vi "MC_8_9_12a_PD.vi"() -> ()   [LabVIEW 2011]
uses:
  <vilib>/Utility/file.llb/Read From Spreadsheet File (string).vi
  <vilib>/Utility/inputDevices.llb/keyboardAcquire.vi
  <vilib>/Utility/file.llb/Write To Spreadsheet File (DBL).vi
  <vilib>/Utility/file.llb/Write To Spreadsheet File (string).vi
  <vilib>/regexp/Match Regular Expression.xnode
panel:
  out "Opj X Axis":string
  in  "Room Temp":dbl=294.0
  out "No Image 2":path=path "\\\\acad1\\physics/Jurchescu-group/JW-PD/Image Not Found.png"
  out "Save1 Array":string[][](array[string])
  out "Lin Vd":dbl
  out "Lin-Vg Array-Used":dbl[](array[numeric])
  out "Lin Id-Used":dbl[](array[numeric])
  out "Comments":string
  out "Folder Index":dbl caption="Length"
  out "Current \nRecord":string[](array[string])
  out "Transformer \nHeaders":string[](array[string])
  out "Current Device ID":string
  out "Column":string
  out "Row":string
  out "Rec: Concentration":dbl
  out "Rec: Solvent":string
  out "Rec: Method":string
  in  "?":T1(tab)
  in  "Transport File":path
  out "Transport Folder":path
  out "Rec: Material":string
  in  "Treatment Concentration (mM):":dbl=nan
  in  "Surface Treatment:":string="NaN"
  in  "# Drops*:":dbl=inf
  in  "Solution Temp (C):":dbl=nan
  in  "Relative Humidity (%):":dbl=nan
  in  "Room Temp (F):":dbl=nan
  in  "Time (s):":dbl=nan
  out "Accel (RPM/s):":dbl
  in  "RPM:":dbl=nan
  in  "Wait Time (s):":dbl=nan
  in  "Sample #:":dbl=1.0
  in  "Fabricator:":string="NaN"
  in  "Transfer File":path
  out "Transfer Folder":path
  in  "Image Folder":path
  out "Image File":path=path "D:/UserData/Desktop/Jeremy/WFU/Research/Programs/VI mods/Image Not Found.png"
  in  "Ramp (s):":dbl=3.0
  out "Calc: On/Off":dbl caption="On/Off-Sat" format="%#.2e"
  out "Calc: Off I-Sat":dbl caption="Off I-Sat" format="%#.2e"
  in  "Manuel-Dielectric":bool
  in  "Manuel-Length":bool
  out "Calc: VT-Lin":dbl
  out "New: VT-Lin":dbl
  out "Rec: VT-Lin":dbl caption="VT-Lin" format="%#_3g"
  out "Calc: Trap Density-STS":dbl format="%#.2e"
  out "New: Trap Density-STS":dbl format="%#.2e"
  out "Rec: Trap Density-STS":dbl caption="N-Sat (STS)" format="%#.2e"
  out "Calc: Trap Density-VT":dbl format="%#.2e"
  out "New: Trap Density-VT":dbl format="%#.2e"
  out "Rec: Trap Density-VT":dbl caption="N-Sat (VT)" format="%#.2e"
  out "Calc: Mobility-Lin":dbl format="%#.2e"
  out "New: Mobility-Lin":dbl format="%#_4e"
  out "Rec: Mobility-Lin":dbl caption="Mobility-Lin" format="%#_3e"
  out "Calc: Mobility-Sat":dbl format="%#.2e"
  out "Rec: Length":dbl caption="Length" format="%#_3g"
  out "Rec: Width":dbl caption="Width" format="%#_4g"
  out "Rec: Dielectric (d)":dbl caption="Dielectric (d)" format="%#_3g"
  in  "Cancel Button":bool
  in  "Up Button":bool
  in  "Down Button":bool
  out "Data Name:":string
  in  "Save Changes?":bool
  in  "New: Dielectric":dbl
  in  "New: Length":dbl
  in  "New: Width":dbl
  out "New: Mobility-Sat":dbl format="%#.2e"
  in  "Blank Button":bool
  in  "Zoom":i16(slide)=-3 scale=-5.0..5.0
  out "Image Out 2":T2(plugin-control)
  out "Image Out":T2(plugin-control)
  in  "Magnification":u16(ring) items=["5x", "10x", "20x", "50x", "80x"]
  out "Total Width":dbl
  out "Distances":dbl[](array[numeric])
  in  "Undo Button":bool
  in  "Remove Button":bool
  out "Rec: Mobility-Sat":dbl caption="Mobility-Sat" format="%#.2e"
  out "Index":string
  out "Image Name":string
  in  "Export":bool
  out "Calc: VT-Sat":dbl format="%#.2g"
  out "New: VT-Sat":dbl format="%#.2g"
  in  "Manual-Width":bool caption="Manual"
  out "Calc: STS":dbl format="%#.2g"
  out "New: STS":dbl format="%#.2g"
  out "Rec: VT-Sat":dbl caption="VT-Sat" format="%#.2g"
  out "Rec: STS":dbl caption="STS-Sat" format="%#.2g"
  out "Rec: On/Off":dbl caption="On/Off-Sat" format="%#.2e"
  in  "Save Changes? 2":bool
  in  "Save Changes? 3":bool
  out "Date Recorded":string="Date Recorded" caption="Measured"
  out "Date Created":string caption="Fabricated"
  out "Rec: Temp":dbl caption="Sample Temp" format="%.1f"
  in  "New: Temp":dbl format="%.1f"
  out "Rec: Off I-Sat":dbl caption="Off I-Sat" format="%#.2e"
  in  "Independant Variable":string(combo)="Length (um):"
  in  "Transfer Plots":enum32{"Linear", "Saturation"}(tab)=enum."Saturation"
  out "XY Graph-Lin":cluster{dbl[], dbl[]}[](graph)
  in  "Slide":dbl(slide) step=1.0 scale=-22.0..89.0 scale format="%#_1p"
  out "XY Graph":cluster{dbl[], dbl[]}[](graph)
  in  "Previous Button":bool
  in  "Next Button":bool
  in  "NumPts":dbl=5.0
  in  "Log Plots":enum32{"Linear", "Saturation"}(tab)=enum."Saturation"
  in  "Slide 2":dbl(slide) step=1.0 scale=-1.0..82.0 scale format="%#_1p"
  out "XY Graph 2":cluster{dbl[], dbl[]}[](graph)
  in  "Previous Button 2":bool
  in  "Next Button 2":bool
  in  "NumPts 2":dbl=5.0 caption="NumPts"
  in  "Manual-Temp":bool caption="Manual"
  in  "Origin Project File":path=path "\\\\acad1\\physics/Jurchescu-group/JW-PD/Group Library/Origin Project Files/DeviceData_7_31_12b_JW.opj"
  in  "No Image File":path=path "\\\\acad1\\physics/Jurchescu-group/JW-PD/Mega Awesome/Image Not Found.png"
  out "String":string
  out "Index 2":dbl
  out "Sat Id-Log-Used":dbl[](array[numeric])
  out "Vg Array-Log-Used":dbl[](array[numeric])
  out "ROI Descriptor out":T3 {"Contours"."Type" items=["No Selection", "Point", "Line", "Rectangle", "Oval", "Polygon", "Freehand Region", "Annulus", "Unused2", "Unused3", "Broken Line", "Freehand Line", "Rotated Rectangle"]}
  out "ROI Descriptor":T3 {"Contours"."Type" items=["No Selection", "Point", "Line", "Rectangle", "Oval", "Polygon", "Freehand Region", "Annulus", "Unused2", "Unused3", "Broken Line", "Freehand Line", "Rotated Rectangle"]}
  out "Numeric 3":dbl
  out "Array 6":dbl[][](array[numeric])
  out "Cluster":T4
  out "Array 5":dbl[](array[numeric])
  out "Array 4":dbl[](array[numeric])
  out "Array 3":dbl[](array[numeric])
  out "Numeric 2":dbl
  out "Numeric":dbl
  out "Sat Id-Used":dbl[](array[numeric])
  out "Sat Vg Array-Used":dbl[](array[numeric])
  out "MobVi Index":dbl
  in  "Row Start":dbl=20.0
  # "Data Locations"
  # "Transport Location"
  # "Transfer Location"
  # "Image Location"
  # "Sample Properties"
  # "*     Inf = Full coverage\n   NaN = Unknown or Not Applicable"
  # "Recorded"
  # "Calculated"
  # "Re-Calculated"
  # "Manual"
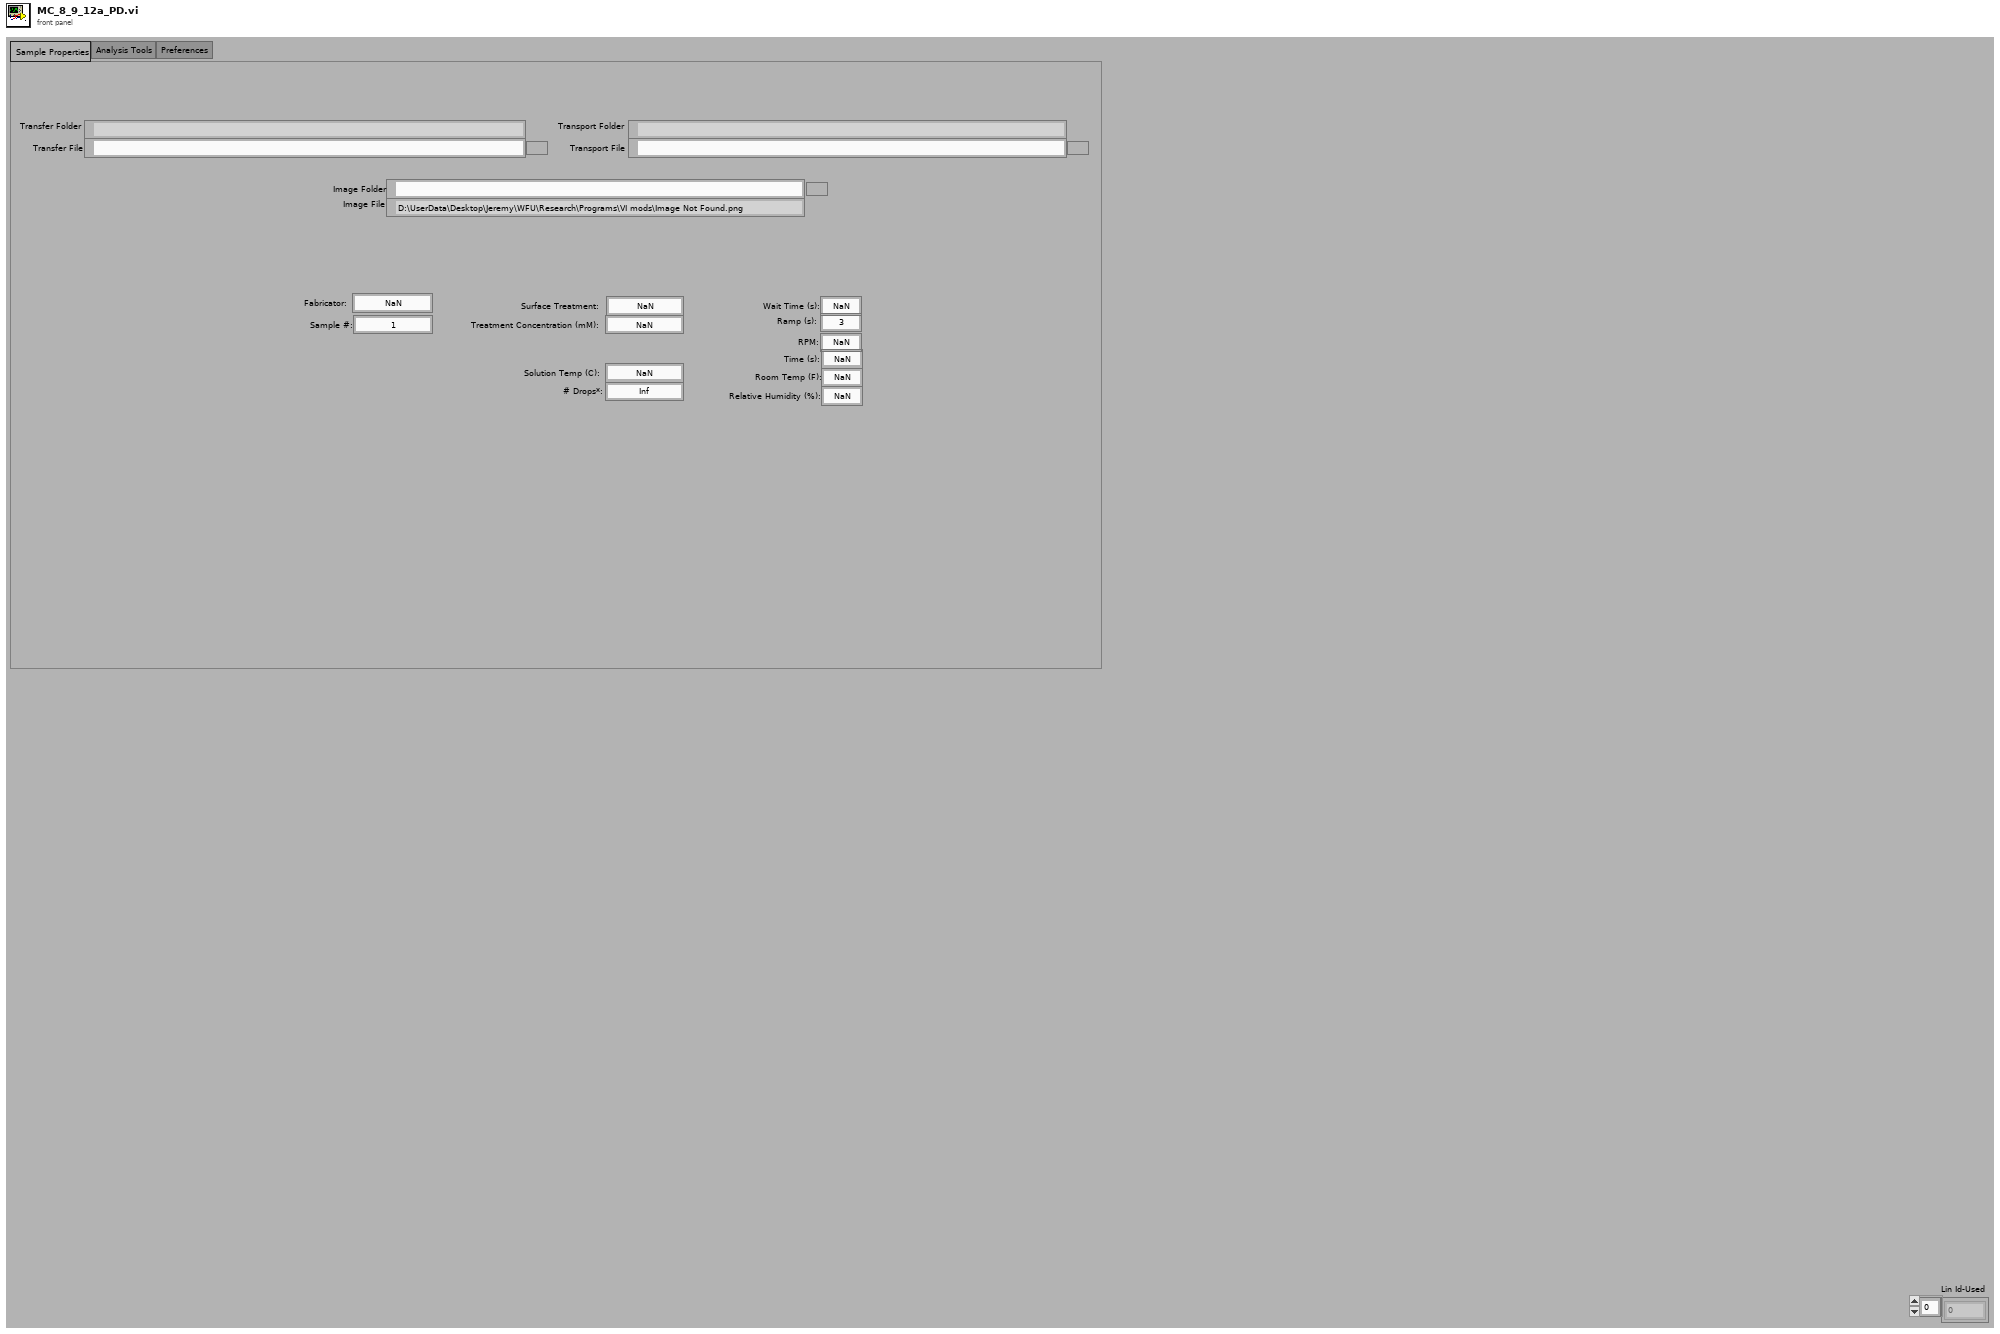
[diagram p1: front panel]
types:
  T1 = enum32{"Sample Properties", "Analysis Tools", "Preferences", "Current Database"}
  T2 = typedef "IMAQ Image.ctl" = refnum<image>
  T3 = typedef "ROI Descriptor" = cluster{"Global Rectangle":i32[], "Contours":cluster{"ID":enum32{"External", "Internal"}, "Type":u32, "Coordinates":i32[]}[]}
  T4 = cluster{"Numeric":dbl, "Numeric 2":dbl, "Numeric 3":dbl, "Numeric 4":dbl}
  T5 = cluster{"Mobility-Sat":dbl, "Moblitity-Lin":dbl, "On/Off":dbl, "Off Current":dbl, "Vt-Sat":dbl, "STS":dbl, "Trap Density-VT":dbl, "Trap Density-STS":dbl}
  T6 = cluster{"Date Recorded":string, "Index":string, "Length":dbl, "Width":dbl, "Sample Temp":dbl}
  T7 = cluster{"Date Created":string, "Material":string, "Solvent":string, "Concentration":dbl, "Method":string, "Dielectric (nm)":dbl, "Treatment":string, "Comments":string}
  T8 = cluster{"Mobility-Sat":dbl, "Vt-Sat":dbl, "Mobility-Lin":dbl, "Vt-Lin":dbl, "Off I-Sat":dbl, "On/Off I-Sat":dbl}
  T9 = cluster{"[0]":cluster{dbl[], dbl[]}, "[1]":cluster{dbl[], dbl[]}, "[2]":cluster{dbl[], dbl[]}, "[3]":cluster{dbl[], dbl[]}, "[4]":cluster{dbl[], dbl[]}, "[5]":cluster{dbl[], dbl[]}, "[6]":cluster{dbl[], dbl[]}, "[7]":cluster{dbl[], dbl[]}, "[8]":cluster{dbl[], dbl[]}}
  T10 = cluster{"Global Rectangle":i32[], "Contours":cluster{"Contour Type":u32, "ROI Type":u32, "Points":i32[]}[]}
  T11 = typedef "LVBoundsTypeDef.ctl" = cluster{"Width":u32, "Height":u32}
  T12 = enum16{"0", "1", "2", "3", "4", "5", "6", "7", "8", "9", "A", "B", "C", "D", "E", "F", "G", "H", "I", "J", "K", "L", "M", "N", "O", "P", "Q", "R", "S", "T", "U", "V", "W", "X", "Y", "Z", "F1", "F2", "F3", "F4", "F5", "F6", "F7", "F8", "F9", "F10", "F11", "F12", "F13", "F14", "F15", "ADD", "BACK", "BACKSLASH", "CAPITAL", "COMMA", "DECIMAL", "DELETE", "DIVIDE", "DOWN", "END", "EQUALS", "ESCAPE", "GRAVE (`)", "HOME", "INSERT", "LBRACKET", "LCONTROL", "LEFT", "L ALT", "LSHIFT", "LWIN", "MINUS", "MULTIPLY", "NEXT", "NUMLOCK", "NUMPAD_0", "NUMPAD_1", "NUMPAD_2", "NUMPAD_3", "NUMPAD_4", "NUMPAD_5", "NUMPAD_6", "NUMPAD_7", "NUMPAD_8", "NUMPAD_9", "PAUSE", "PERIOD", "PRIOR (PG UP)", "RBRACKET", "RCONTROL", "RETURN", "RIGHT", "R ALT", "RSHIFT", "RWIN", "SCROLL", "SEMICOLON", "SLASH", "SPACE", "SUBTRACT", "TAB", "UP", "ENTER (num pad)", "' (quote)"}[]
  T13 = enum16{"0", "1", "2", "3", "4", "5", "6", "7", "8", "9", "A", "B", "C", "D", "E", "F", "G", "H", "I", "J", "K", "L", "M", "N", "O", "P", "Q", "R", "S", "T", "U", "V", "W", "X", "Y", "Z", "F1", "F2", "F3", "F4", "F5", "F6", "F7", "F8", "F9", "F10", "F11", "F12", "F13", "F14", "F15", "ADD", "BACK", "BACKSLASH", "CAPITAL", "COMMA", "DECIMAL", "DELETE", "DIVIDE", "DOWN", "END", "EQUALS", "ESCAPE", "GRAVE (`)", "HOME", "INSERT", "LBRACKET", "LCONTROL", "LEFT", "L ALT", "LSHIFT", "LWIN", "MINUS", "MULTIPLY", "NEXT", "NUMLOCK", "NUMPAD_0", "NUMPAD_1", "NUMPAD_2", "NUMPAD_3", "NUMPAD_4", "NUMPAD_5", "NUMPAD_6", "NUMPAD_7", "NUMPAD_8", "NUMPAD_9", "PAUSE", "PERIOD", "PRIOR (PG UP)", "RBRACKET", "RCONTROL", "RETURN", "RIGHT", "R ALT", "RSHIFT", "RWIN", "SCROLL", "SEMICOLON", "SLASH", "SPACE", "SUBTRACT", "TAB", "UP", "ENTER (num pad)", "' (quote)"}
  T14 = cluster{"Contour Type":u32, "ROI Type":u32, "Points":i32[]}[]
  T15 = cluster{i32[], cluster{"Contour Type":u32, "ROI Type":u32, "Points":i32[]}[]}
  T16 = cluster{"Independant  Variable Indicator":string, "Parameter String Indicator":string}
  T17 = cluster{string, sgl, bool, bool, bool, bool, bool, bool, i32}
  T18 = cluster{i32, cluster{string, sgl, bool, bool, bool, bool, bool, bool, i32}, i32, i32}
  T19 = cluster{"Contour Type":u32, "ROI Type":u32, "Points":i32[]}
  T20 = cluster{"Points[0]":i32, "Points[1]":i32, "Points[2]":i32, "Points[3]":i32, "Points[4]":i32, "Points[5]":i32, "Points[6]":i32, "Points[7]":i32, "Points[8]":i32}
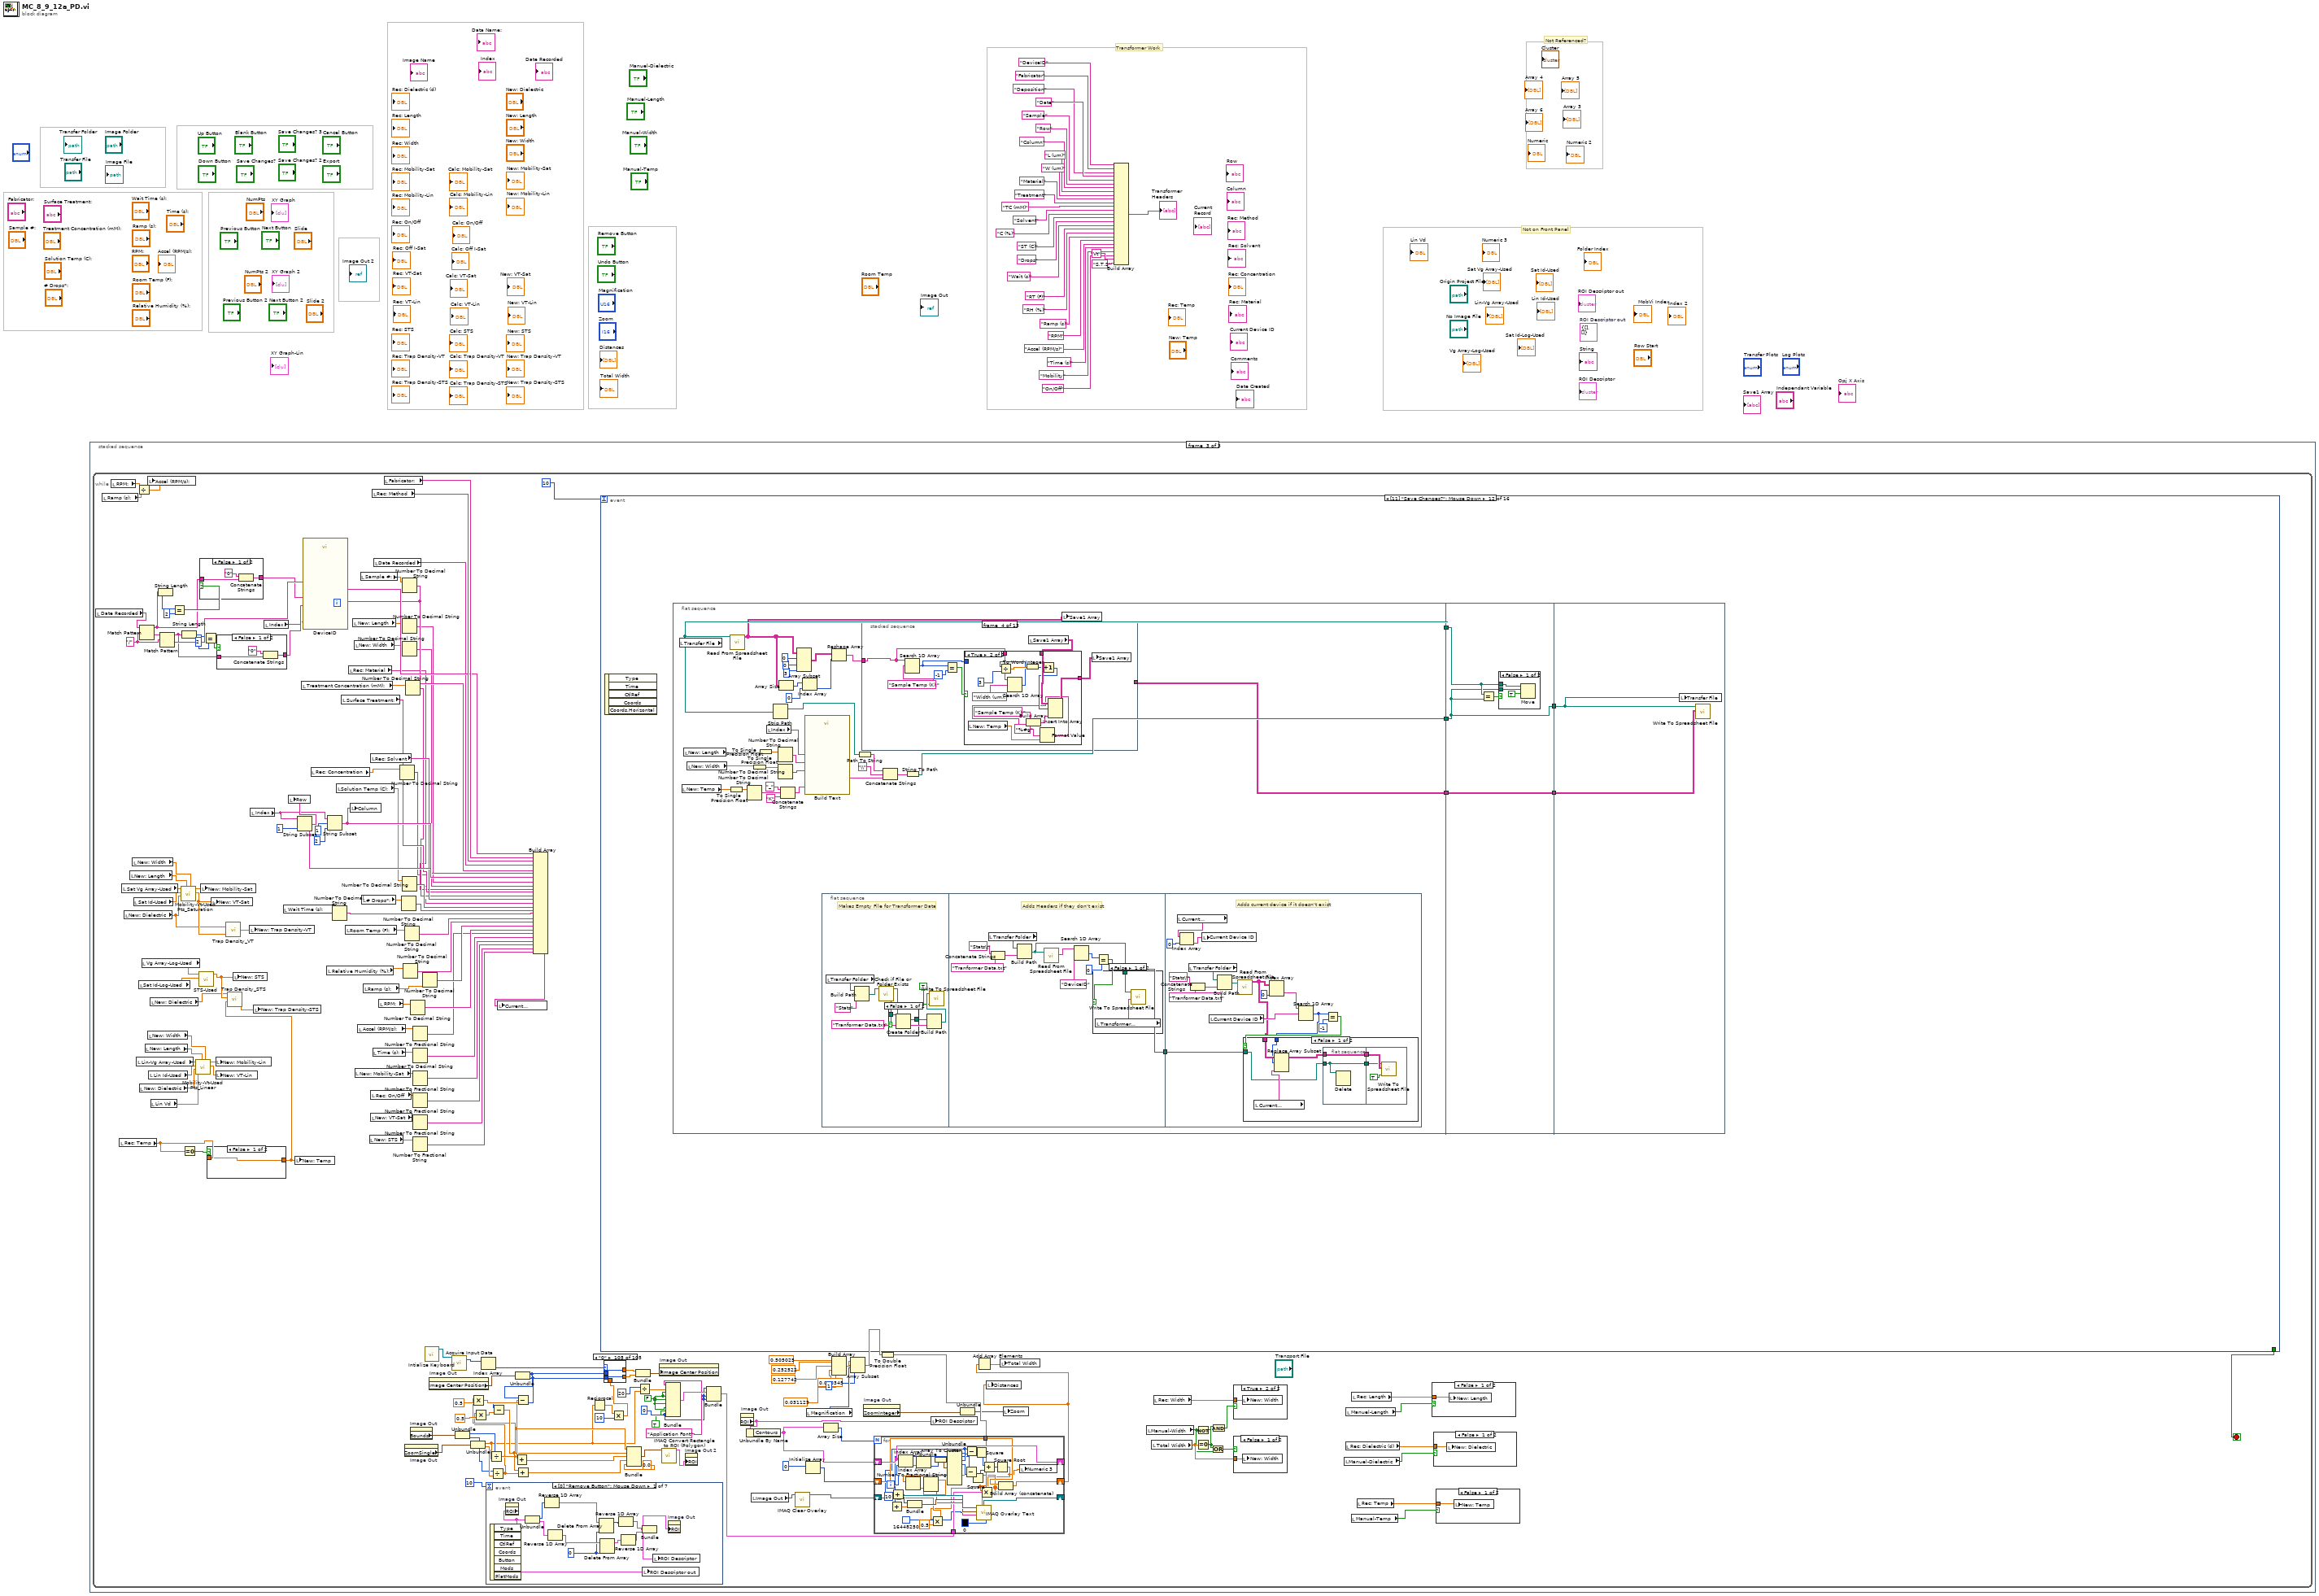
[diagram p0: block diagram]
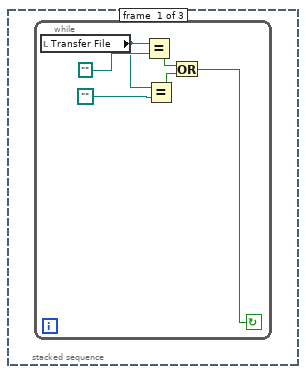
[diagram p2: hidden frame]
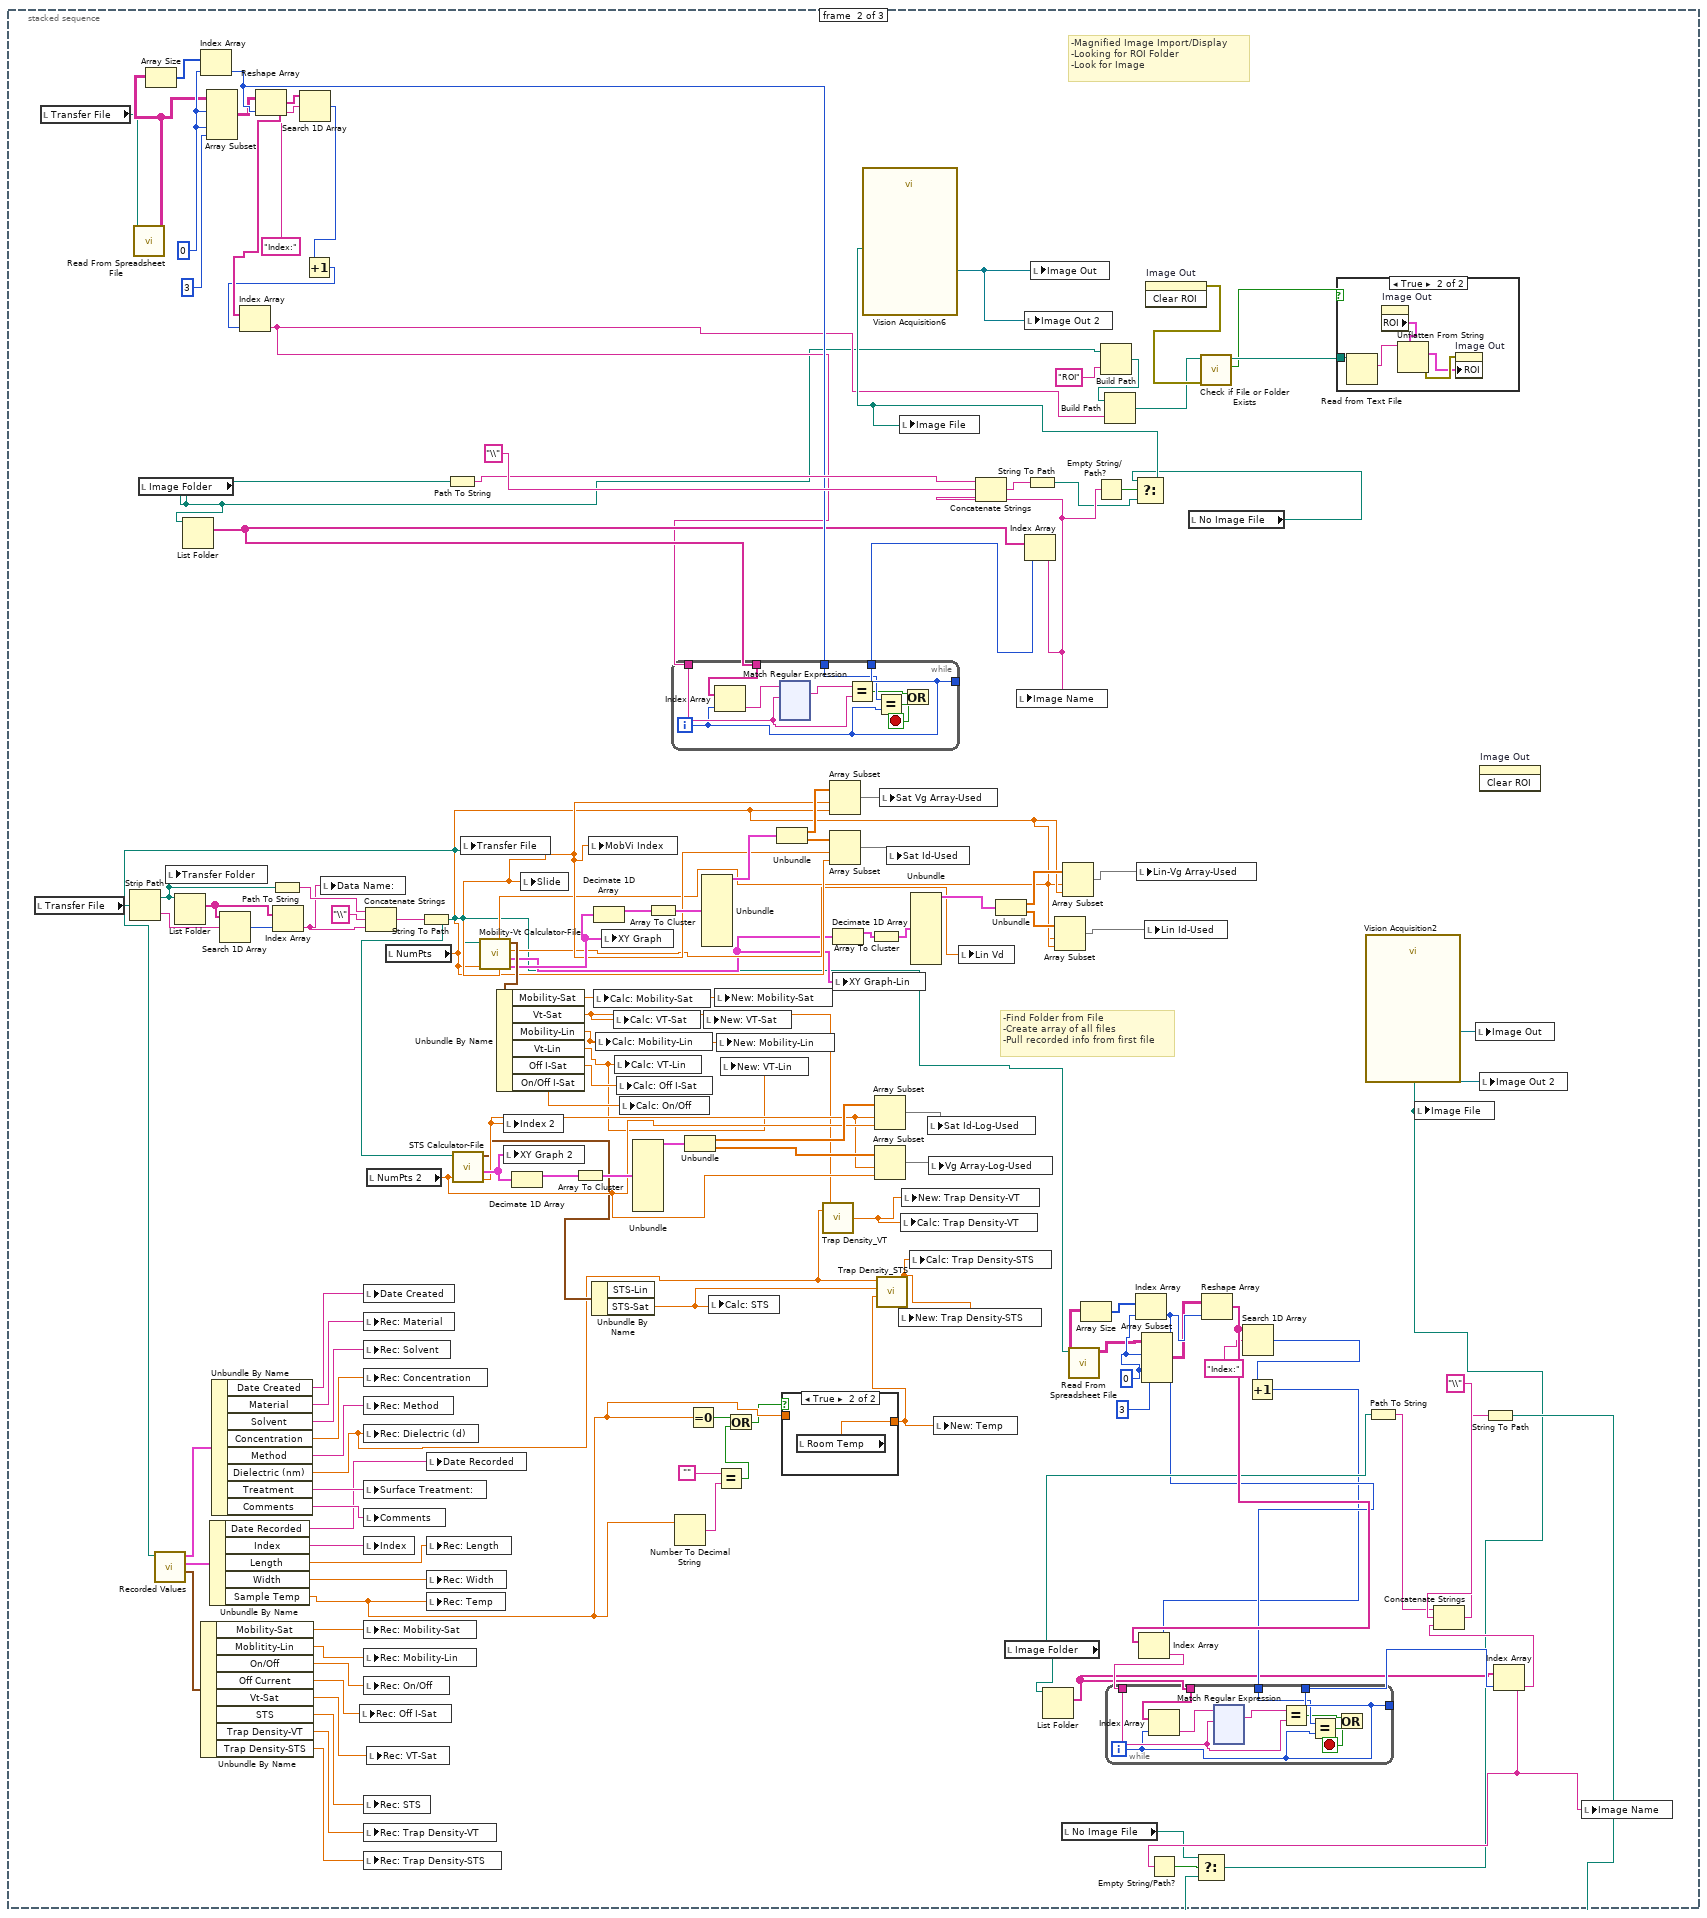
[diagram p3: hidden frame]
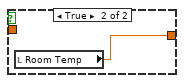
[diagram p7: hidden frame]
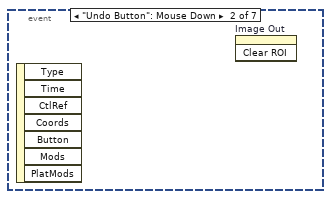
[diagram p14: hidden frame]
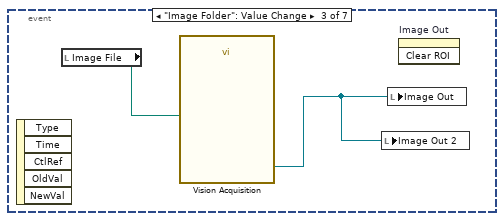
[diagram p15: hidden frame]
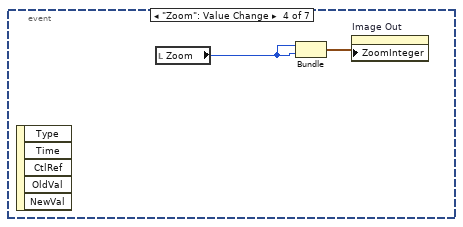
[diagram p16: hidden frame]
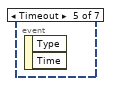
[diagram p17: hidden frame]
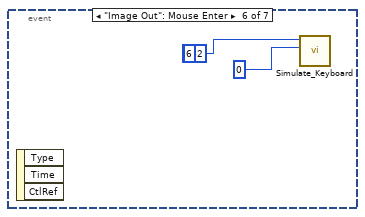
[diagram p18: hidden frame]
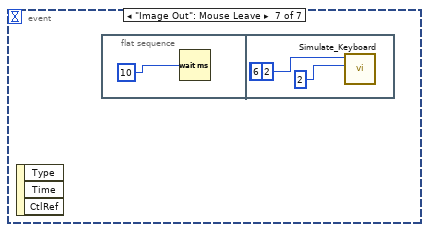
[diagram p19: hidden frame]
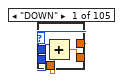
[diagram p20: hidden frame]
diagram:
  (unwired) T3 {"Global Rectangle"=[], "Contours"=[]}  # ROI Descriptor out
  # "Not Referenced?"
  # "Transformer Work"
  # "Not on Front Panel"
  n1 = stacked-sequence {
    frame #0 {
      n2 = while {
        stop <- w29 continue-if-true
        n3 = local read "Transfer File"() -> (w31:path)
        n4 = Equal?(x=w31, y=path "") -> (x = y?=w33:bool)
        n5 = Equal?(x=w31, y=path "") -> (x = y?=w32:bool)
        n6 = Or(x=w33, y=w32) -> (x .or. y?=w29:bool)
      }
    }
    frame #1 {
      w133 = 0
      w157 = 0
      # "-Find Folder from File\n-Create array of all files\n-Pull recorded info from first file"
      # "-Magnified Image Import/Display\n-Looking for ROI Folder\n-Look for Image"
      n7 = local read "Transfer File"() -> (w137:path)
      n8 = local read "Transfer File"() -> (w152:path)
      n9 = Strip Path(path=w137) -> (stripped path=w138:path, name=w124:string)
      n10 = call-poly <vilib>:"Read From Spreadsheet File.vi"("file path (dialog if empty)"=w152) -> ("all rows"=w155:string[][])  [unwired: 6 in, 4 out]
      n11 = local read "Image Folder"() -> (w94:path)
      n12 = Array Size(array=w155) -> (size(s)=w156:i32[])
      n13 = local write "Transfer Folder"(w138) -> ()
      n14 = List Folder(path=w138) -> (filenames=w128:string[])  [unwired: 3 in, 3 out]
      n15 = List Folder(path=w94) -> (filenames=w161:string[])  [unwired: 3 in, 3 out]
      n16 = Index Array(array=w156, index=w157) -> (element=w163:i32)
      n17 = Array Subset(array=w155, index (row)=w157, index (col)=w157, length (col)=3) -> (w154:string[][])  [unwired: 1 in]
      n18 = Search 1D Array(1D array=w128, element=w124) -> (index of element=w127:i32)  [unwired: 1 in]
      n19 = Reshape Array(w154, w163) -> (w168:string[])
      n20 = Path To String(path=w138) -> (string=w123:string)
      n21 = Index Array(array=w128, index=w127) -> (element=w93:string)
      n22 = Search 1D Array(1D array=w168, element="Index:") -> (index of element=w160:i32)  [unwired: 1 in]
      n23 = Increment(x=w160) -> (x+1=w159:i32)
      n24 = Index Array(array=w168, index=w159) -> (element=w95:string)
      n25 = local write "Data Name:"(w93) -> ()
      n26 = Concatenate Strings(w123, "\\", w93) -> (w125:string)
      n27 = local read "NumPts 2"() -> (w68:dbl)
      n28 = local read "NumPts"() -> (w59:dbl)
      n29 = String To Path(string=w125) -> (path=w52:path)
      n30 = call "Recorded Values.vi"("Path"=w52) -> ("Recorded Char"=w91:T5, "Recorded Prop"=w90:T6, "Fabrication Prop"=w92:T7)  [unwired: 8 in]
      n31 = Unbundle By Name(w91) -> ("Mobility-Sat"=w79:dbl, "Moblitity-Lin"=w78:dbl, "On/Off"=w77:dbl, "Off Current"=w76:dbl, "Vt-Sat"=w38:dbl, "STS"=w75:dbl, "Trap Density-VT"=w74:dbl, "Trap Density-STS"=w73:dbl)
      n32 = Unbundle By Name(w90) -> ("Date Recorded"=w83:string, "Index"=w82:string, "Length"=w81:dbl, "Width"=w80:dbl, "Sample Temp"=w44:dbl)
      n33 = Unbundle By Name(w92) -> ("Date Created"=w72:string, "Material"=w89:string, "Solvent"=w88:string, "Concentration"=w87:dbl, "Method"=w86:string, "Dielectric (nm)"=w48:dbl, "Treatment"=w85:string, "Comments"=w84:string)
      n34 = local write "Rec: Off I-Sat"(w76) -> ()
      n35 = local write "Date Created"(w72) -> ()
      n36 = local write "Rec: Material"(w89) -> ()
      n37 = local write "Rec: Solvent"(w88) -> ()
      n38 = local write "Rec: Concentration"(w87) -> ()
      n39 = local write "Rec: Method"(w86) -> ()
      n40 = local write "Rec: Dielectric (d)"(w48) -> ()
      n41 = local write "Surface Treatment:"(w85) -> ()
      n42 = local write "Comments"(w84) -> ()
      n43 = local write "Index"(w82) -> ()
      n44 = local write "Rec: Mobility-Sat"(w79) -> ()
      n45 = local write "Rec: Mobility-Lin"(w78) -> ()
      n46 = local write "Rec: On/Off"(w77) -> ()
      n47 = local write "Rec: STS"(w75) -> ()
      n48 = local write "Rec: Trap Density-VT"(w74) -> ()
      n49 = local write "Rec: Trap Density-STS"(w73) -> ()
      n50 = local write "Rec: VT-Sat"(w38) -> ()
      n51 = local write "Date Recorded"(w83) -> ()
      n52 = local write "Rec: Length"(w81) -> ()
      n53 = local write "Rec: Width"(w80) -> ()
      n54 = local write "Rec: Temp"(w44) -> ()
      n55 = Path To String(path=w94) -> (string=w165:string)
      n56 = call "STS Calculator-File.vi"("NumPts"=w68, "Path"=w52) -> ("STS Index-Sat"=w66:dbl, "XY Graph-Sat"=w67:cluster{dbl[], dbl[]}[], "Ouput"=w65:cluster{"STS-Sat":dbl, "STS-Lin":dbl})  [unwired: 5 in, 2 out]
      n57 = local write "Transfer File"(w52) -> ()
      n58 = call "Mobility-Vt Calculator-File.vi"("NumPts"=w59, "Path"=w52) -> ("XY Graph-Sat"=w70:cluster{dbl[], dbl[]}[], "XY Graph-Lin"=w54:cluster{dbl[], dbl[]}[], "Lin Vd"=w55:dbl, "Output"=w71:T8, "Index-Sat"=w69:dbl, "Index-Lin"=w58:dbl)  [unwired: 4 in]
      n59 = Unbundle By Name(w71) -> ("Mobility-Sat"=w47:dbl, "Vt-Sat"=w46:dbl, "Mobility-Lin"=w37:dbl, "Vt-Lin"=w35:dbl, "Off I-Sat"=w53:dbl, "On/Off I-Sat"=w36:dbl)
      n60 = local write "Index 2"(w66) -> ()
      n61 = local write "XY Graph 2"(w67) -> ()
      n62 = Decimate 1D Array(w67) -> (w115:cluster{dbl[], dbl[]}[])  [unwired: 1 out]
      n63 = local write "Slide"(w69) -> ()
      n64 = Array To Cluster(array=w115) -> (cluster=w117:T9)
      n65 = local write "MobVi Index"(w69) -> ()
      n66 = Unbundle By Name(w65) -> ("STS-Sat"=w51:dbl)  [unwired: 1 out]
      n67 = Decimate 1D Array(w70) -> (w151:cluster{dbl[], dbl[]}[])  [unwired: 1 out]
      n68 = local write "Calc: Mobility-Sat"(w47) -> ()
      n69 = local write "Calc: Mobility-Lin"(w37) -> ()
      n70 = local write "XY Graph"(w70) -> ()
      n71 = local write "Calc: VT-Sat"(w46) -> ()
      n72 = local write "Calc: VT-Lin"(w35) -> ()
      n73 = local write "Calc: Off I-Sat"(w53) -> ()
      n74 = local write "Calc: On/Off"(w36) -> ()
      n75 = Unbundle(w117) -> ("[0]"=w116:cluster{dbl[], dbl[]})  [unwired: 8 out]
      n76 = Array To Cluster(array=w151) -> (cluster=w149:T9)
      n77 = while {
        tunnel: w161 -> [w303]
        tunnel: w95 -> [w301]
        tunnel: [w300] -> _
        tunnel: [w300] -> w162
        tunnel: w163 -> [w299]
        i -> [w300]
        stop <- w296 stop-if-true
        n78 = Index Array(array=w303, index=w300) -> (element=w304:string)
        n79 = xnode "Match Regular Expression"("input string"=w304, "regular expression"=w301) -> ("whole match"=w302:string)  [unwired: 4 in, 4 out]
        n80 = Equal?(x=w302, y=w301) -> (x = y?=w298:bool)
        n81 = Equal?(x=w299, y=w300) -> (x = y?=w297:bool)
        n82 = Or(x=w298, y=w297) -> (x .or. y?=w296:bool)
      }
      n83 = Number To Decimal String(number=w44) -> (decimal integer string=w42:string)  [unwired: 1 in]
      n84 = Unbundle(w116) -> (w113:dbl[], w112:dbl[])
      n85 = Equal To 0?(x=w44) -> (x = 0?=w43:bool)
      n86 = Unbundle(w149) -> ("[0]"=w150:cluster{dbl[], dbl[]})  [unwired: 8 out]
      n87 = local write "New: VT-Sat"(w46) -> ()
      n88 = local write "Calc: STS"(w51) -> ()
      n89 = local write "New: Mobility-Sat"(w47) -> ()
      n90 = Equal?(x="", y=w42) -> (x = y?=w40:bool)
      n91 = local write "New: Mobility-Lin"(w37) -> ()
      n92 = local write "New: VT-Lin"(w35) -> ()
      n93 = Or(x=w43, y=w40) -> (x .or. y?=w39:bool)
      n94 = Unbundle(w150) -> (w114:dbl[], w118:dbl[])
      n95 = case shown="True" w39 {
        tunnel: [w169 w170] -> w50
        tunnel: w44 -> [w169 _]
        frame False {
        }
        frame True {
          n96 = local read "Room Temp"() -> (w170:dbl)
        }
      }
      n97 = call "Trap Density_VT.vi"("VT"=w46, "Dielectric"=w48) -> ("Trap Density-VT"=w45:dbl)
      n98 = Array Subset(array=w114, index=w69, length=w59) -> (w121:dbl[])
      n99 = Array Subset(array=w118, index=w69, length=w59) -> (w122:dbl[])
      n100 = Decimate 1D Array(w54) -> (w64:cluster{dbl[], dbl[]}[])  [unwired: 1 out]
      n101 = local write "XY Graph-Lin"(w54) -> ()
      n102 = Array To Cluster(array=w64) -> (cluster=w63:T9)
      n103 = Array Subset(array=w113, index=w66, length=w68) -> (w120:dbl[])
      n104 = Array Subset(array=w112, index=w66, length=w68) -> (w119:dbl[])
      n105 = call "Trap Density_STS.vi"("Temp (T) [K]"=w50, "S.T.S. (S)"=w51, "Dielectric"=w48) -> ("Trap Density (N)"=w49:dbl)  [unwired: 8 in]
      n106 = local write "Sat Vg Array-Used"(w121) -> ()
      n107 = local write "Sat Id-Used"(w122) -> ()
      n108 = local write "New: Trap Density-STS"(w49) -> ()
      n109 = local write "Calc: Trap Density-VT"(w45) -> ()
      n110 = local write "New: Trap Density-VT"(w45) -> ()
      n111 = local write "Calc: Trap Density-STS"(w49) -> ()
      n112 = Unbundle(w63) -> ("[0]"=w62:cluster{dbl[], dbl[]})  [unwired: 8 out]
      n113 = local write "Sat Id-Log-Used"(w120) -> ()
      n114 = local write "Vg Array-Log-Used"(w119) -> ()
      n115 = local write "New: Temp"(w50) -> ()
      n116 = local write "Lin Vd"(w55) -> ()
      n117 = Unbundle(w62) -> (w61:dbl[], w60:dbl[])
      n118 = local read "Image Folder"() -> (w144:path)
      n119 = Index Array(array=w161, index=w162) -> (element=w111:string)
      n120 = Concatenate Strings(w165, "\\", w111) -> (w166:string)
      n121 = local write "Image Name"(w111) -> ()
      n122 = String To Path(string=w166) -> (path=w109:path)
      n123 = List Folder(path=w144) -> (filenames=w140:string[])  [unwired: 3 in, 3 out]
      n124 = Array Subset(array=w60, index=w58, length=w59) -> (w56:dbl[])
      n125 = local read "No Image File"() -> (w103:path)
      n126 = Array Subset(array=w61, index=w58, length=w59) -> (w57:dbl[])
      n127 = call-poly <vilib>:"Read From Spreadsheet File.vi"("file path (dialog if empty)"=w52) -> ("all rows"=w131:string[][])  [unwired: 6 in, 4 out]
      n128 = Array Size(array=w131) -> (size(s)=w132:i32[])
      n129 = Empty String/Path?(string/path=w111) -> (empty?=w110:bool)
      n130 = Build Path(base path=w94, name or relative path="ROI") -> (appended path=w97:path)
      n131 = Build Path(base path=w97, name or relative path=w95) -> (appended path=w96:path)
      n132 = Index Array(array=w132, index=w133) -> (element=w143:i32)
      n133 = local write "Lin-Vg Array-Used"(w57) -> ()
      n134 = Array Subset(array=w131, index (row)=w133, index (col)=w133, length (col)=3) -> (w130:string[][])  [unwired: 1 in]
      n135 = local write "Lin Id-Used"(w56) -> ()
      n136 = invoke on="Image Out" class="ImageControl" method="Clear ROI"() -> (error out=w101:errorcluster)  [unwired: 3 in, 2 out]
      n137 = local read "No Image File"() -> (w102:path)
      n138 = Select(t=w102, s=w110, f=w109) -> (s? t:f=w108:path)
      n139 = call "Vision Acquisition6"("Image Path"=w108) -> ("Image Out"=w164:T2)  [unwired: 25 in, 1 out]
      n140 = local write "Image File"(w108) -> ()
      n141 = local write "Image Out 2"(w164) -> ()
      n142 = local write "Image Out"(w164) -> ()
      n143 = call <vilib>:"Check if File or Folder Exists.vi"("error in (no error)"=w101, "path"=w96) -> ("file or folder exists?"=w99:bool, "dup path"=w100:path)  [unwired: 7 in, 1 out]
      n144 = Reshape Array(w130, w143) -> (w148:string[])
      n145 = Search 1D Array(1D array=w148, element="Index:") -> (index of element=w136:i32)  [unwired: 1 in]
      n146 = Increment(x=w136) -> (x+1=w135:i32)
      n147 = Index Array(array=w148, index=w135) -> (element=w141:string)
      n148 = while {
        tunnel: w140 -> [w183]
        tunnel: w141 -> [w181]
        tunnel: [w180] -> _
        tunnel: [w180] -> w142
        tunnel: w143 -> [w179]
        i -> [w180]
        stop <- w176 stop-if-true
        n149 = Index Array(array=w183, index=w180) -> (element=w184:string)
        n150 = xnode "Match Regular Expression"("input string"=w184, "regular expression"=w181) -> ("whole match"=w182:string)  [unwired: 4 in, 4 out]
        n151 = Equal?(x=w182, y=w181) -> (x = y?=w178:bool)
        n152 = Equal?(x=w179, y=w180) -> (x = y?=w177:bool)
        n153 = Or(x=w178, y=w177) -> (x .or. y?=w176:bool)
      }
      n154 = case shown="True" w99 {
        tunnel: w100 -> [_ w171]
        frame False {
        }
        frame True {
          n155 = Read from Text File(file (use dialog)=w171) -> (text=w175:string)  [unwired: 3 in, 3 out]
          n156 = property on="Image Out" class="ImageControl"() -> ("ROI"=w172:T10)  [unwired: 2 in, 2 out]
          n157 = Unflatten From String(type=w172, binary string=w175) -> (value=w173:T10, error out=w174:errorcluster)  [unwired: 3 in, 1 out]
          n158 = property on="Image Out" class="ImageControl"(error in=w174, "ROI"=w173) -> ()  [unwired: 1 in, 2 out]
        }
      }
      n159 = Path To String(path=w144) -> (string=w145:string)
      n160 = invoke on="Image Out" class="ImageControl" method="Clear ROI"() -> ()  [unwired: 3 in, 3 out]
      n161 = Index Array(array=w140, index=w142) -> (element=w106:string)
      n162 = Empty String/Path?(string/path=w106) -> (empty?=w107:bool)
      n163 = Concatenate Strings(w145, "\\", w106) -> (w146:string)
      n164 = String To Path(string=w146) -> (path=w105:path)
      n165 = Select(t=w103, s=w107, f=w105) -> (s? t:f=w104:path)
      n166 = call "Vision Acquisition2"("Image Path"=w104) -> ("Image Out"=w139:T2)  [unwired: 25 in, 1 out]
      n167 = local write "Image File"(w104) -> ()
      n168 = local write "Image Out"(w139) -> ()
      n169 = local write "Image Out 2"(w139) -> ()
      n170 = local write "Image Name"(w106) -> ()
    }
    frame #2 {
      n171 = while {
        stop <- w583 stop-if-true
        w479 = "/"
        w533 = FALSE
        w531 = 0
        n172 = local read "Date Recorded"() -> (w482:string)
        n173 = local read "Ramp (s):"() -> (w449:dbl)
        n174 = local read "RPM:"() -> (w450:dbl)
        n175 = local read "Rec: Temp"() -> (w421:dbl)
        n176 = local read "Sat Vg Array-Used"() -> (w438:dbl[])
        n177 = local read "New: Dielectric"() -> (w423:dbl)
        n178 = local read "New: Length"() -> (w439:dbl)
        n179 = local read "New: Width"() -> (w441:dbl)
        n180 = local read "Sat Id-Used"() -> (w437:dbl[])
        n181 = local read "Lin-Vg Array-Used"() -> (w432:dbl[])
        n182 = Divide(x=w450, y=w449) -> (x/y=w448:dbl)
        n183 = local read "Sat Id-Log-Used"() -> (w436:dbl[])
        n184 = local read "New: Dielectric"() -> (w429:dbl)
        n185 = Match Pattern(string=w482, regular expression=w479) -> (before substring=w473:string, after substring=w480:string)  [unwired: 1 in, 2 out]
        n186 = local read "Vg Array-Log-Used"() -> (w435:dbl[])
        n187 = local read "New: Length"() -> (w431:dbl)
        n188 = local write "Accel (RPM/s):"(w448) -> ()
        n189 = local read "New: Width"() -> (w428:dbl)
        n190 = local read "Lin Id-Used"() -> (w433:dbl[])
        n191 = local read "New: Dielectric"() -> (w425:dbl)
        n192 = local read "Lin Vd"() -> (w427:dbl)
        n193 = String Length(string=w473) -> (length=w476:i32)
        n194 = Match Pattern(string=w480, regular expression=w479) -> (before substring=w467:string, after substring=w478:string)  [unwired: 1 in, 2 out]
        n195 = Equal?(x=w476, y=2) -> (x = y?=w474:bool)
        n196 = call "Mobility-Vt-Used Pts_Saturation.vi"("Width"=w441, "Length"=w439, "Dielectric (d)"=w423, "Sat Id Used"=w437, "Vg Used"=w438) -> ("Vt"=w424:dbl, "Mobility"=w440:dbl)  [unwired: 4 in, 1 out]
        n197 = String Length(string=w467) -> (length=w469:i32)
        n198 = Equal To 0?(x=w421) -> (x = 0?=w420:bool)
        n199 = call "Mobility-Vt-Used Pts_Linear.vi"("Width"=w428, "Length"=w431, "Vd"=w427, "Dielectric (d)"=w429, "Sat Id Used"=w433, "Vg Used"=w432) -> ("Vt"=w434:dbl, "Mobility"=w430:dbl)  [unwired: 3 in, 1 out]
        n200 = call "STS-Used.vi"("Id Used"=w436, "Vg-Used"=w435) -> ("STS"=w426:dbl)  [unwired: 9 in]
        n201 = case shown="False" w474 {
          tunnel: w473 -> [w594 w596]
          tunnel: [w593 w596] -> w472
          frame False {
            n202 = Concatenate Strings("0", w594) -> (w593:string)
          }
          frame True {
          }
        }
        n203 = local write "New: Mobility-Sat"(w440) -> ()
        n204 = Equal?(x=w469, y=2) -> (x = y?=w471:bool)
        n205 = case shown="False" w420 {
          tunnel: [w585 w586] -> w418
          tunnel: w421 -> [w585 _]
          frame False {
          }
          frame True {
            n206 = local read "Room Temp"() -> (w586:dbl)
          }
        }
        n207 = local write "New: VT-Sat"(w424) -> ()
        n208 = local write "New: Mobility-Lin"(w430) -> ()
        n209 = local write "New: VT-Lin"(w434) -> ()
        n210 = case shown="False" w471 {
          tunnel: w467 -> [w590 w592]
          tunnel: [w589 w592] -> w468
          frame False {
            n211 = Concatenate Strings("0", w590) -> (w589:string)
          }
          frame True {
          }
        }
        n212 = call "Trap Density_VT.vi"("VT"=w424, "Dielectric"=w423) -> ("Trap Density-VT"=w422:dbl)
        n213 = call "Trap Density_STS.vi"("Temp (T) [K]"=w418, "S.T.S. (S)"=w426, "Dielectric"=w425) -> ("Trap Density (N)"=w419:dbl)  [unwired: 8 in]
        n214 = local write "New: STS"(w426) -> ()
        n215 = local write "New: Trap Density-VT"(w422) -> ()
        n216 = local read "Index"() -> (w452:string)
        n217 = local write "New: Trap Density-STS"(w419) -> ()
        n218 = local read "Index"() -> (w466:string)
        n219 = local read "Wait Time (s):"() -> (w512:dbl)
        n220 = local write "New: Temp"(w418) -> ()
        n221 = String Subset(string=w452, length (rest)=1) -> (substring=w507:string)  [unwired: 1 in]
        n222 = local write "Row"(w507) -> ()
        n223 = local read "Treatment Concentration (mM):"() -> (w460:dbl)
        n224 = local read "Rec: Concentration"() -> (w447:dbl)
        n225 = local read "Relative Humidity (%):"() -> (w457:dbl)
        n226 = String Subset(string=w452, offset (0)=1, length (rest)=2) -> (substring=w508:string)
        n227 = Number To Decimal String(number=w512) -> (decimal integer string=w513:string)  [unwired: 1 in]
        n228 = local read "Solution Temp (C):"() -> (w501:dbl)
        n229 = local read "Surface Treatment:"() -> (w459:string)
        n230 = local read "Room Temp (F):"() -> (w505:dbl)
        n231 = local read "Rec: Material"() -> (w455:string)
        n232 = local write "Column"(w508) -> ()
        n233 = local read "New: Length"() -> (w465:dbl)
        n234 = local read "New: Width"() -> (w464:dbl)
        n235 = local read "New: Mobility-Sat"() -> (w494:dbl)
        n236 = local read "Accel (RPM/s):"() -> (w492:dbl)
        n237 = local read "Sample #:"() -> (w484:dbl)
        n238 = local read "# Drops*:"() -> (w502:dbl)
        n239 = local read "Ramp (s):"() -> (w510:dbl)
        n240 = local read "New: STS"() -> (w486:dbl)
        n241 = local read "Rec: Solvent"() -> (w461:string)
        n242 = local read "New: VT-Sat"() -> (w488:dbl)
        n243 = local read "Rec: On/Off"() -> (w490:dbl)
        n244 = local read "Rec: Method"() -> (w485:string)
        n245 = local read "Time (s):"() -> (w497:dbl)
        n246 = local read "Date Recorded"() -> (w481:string)
        n247 = local read "RPM:"() -> (w498:dbl)
        n248 = local read "Fabricator:"() -> (w506:string)
        n249 = Number To Decimal String(number=w447) -> (decimal integer string=w446:string)  [unwired: 1 in]
        n250 = Number To Decimal String(number=w502) -> (decimal integer string=w503:string)  [unwired: 1 in]
        n251 = Number To Decimal String(number=w484) -> (decimal integer string=w477:string)  [unwired: 1 in]
        n252 = call "DeviceID"("Sample"=w477, "Year"=w478, "Month"=w472, "Day"=w468, "Index"=w466) -> ("Result"=w483:string)  [unwired: 9 in, 1 out]
        n253 = Number To Decimal String(number=w465) -> (decimal integer string=w463:string)  [unwired: 1 in]
        n254 = Number To Decimal String(number=w464) -> (decimal integer string=w462:string)  [unwired: 1 in]
        n255 = Number To Decimal String(number=w501) -> (decimal integer string=w500:string)  [unwired: 1 in]
        n256 = Number To Decimal String(number=w457) -> (decimal integer string=w456:string)  [unwired: 1 in]
        n257 = Number To Decimal String(number=w505) -> (decimal integer string=w504:string)  [unwired: 1 in]
        n258 = property on="Image Out" class="ImageControl"() -> ("ZoomSingle"=w551:cluster{"X":sgl, "Y":sgl})  [unwired: 2 in, 2 out]
        n259 = Number To Decimal String(number=w460) -> (decimal integer string=w458:string)  [unwired: 1 in]
        n260 = property on="Image Out" class="ImageControl"() -> ("Bounds"=w552:T11)  [unwired: 2 in, 2 out]
        n261 = Number To Decimal String(number=w498) -> (decimal integer string=w499:string)  [unwired: 1 in]
        n262 = Number To Fractional String(number=w492) -> (F-format string=w493:string)  [unwired: 3 in]
        n263 = Number To Decimal String(number=w497) -> (decimal integer string=w496:string)  [unwired: 1 in]
        n264 = Number To Fractional String(number=w494) -> (F-format string=w495:string)  [unwired: 3 in]
        n265 = Number To Fractional String(number=w490) -> (F-format string=w491:string)  [unwired: 3 in]
        n266 = Number To Fractional String(number=w488) -> (F-format string=w489:string)  [unwired: 3 in]
        n267 = Number To Fractional String(number=w486) -> (F-format string=w487:string)  [unwired: 3 in]
        n268 = Number To Decimal String(number=w510) -> (decimal integer string=w511:string)  [unwired: 1 in]
        n269 = call <vilib>:"Intialize Keyboard.vi"() -> ("device ID"=w563:refnum<k1>)  [unwired: 10 in, 1 out]
        n270 = property on="Image Out" class="ImageControl"() -> ("Image Center Position"=w558:cluster{"X":u32, "Y":u32})  [unwired: 2 in, 2 out]
        n271 = call-poly <vilib>:"Acquire Input Data.vi"("device ID"=w563) -> ("keys pressed"=w562:T12)  [unwired: 16 in, 2 out]
        n272 = Unbundle(w552) -> ("Width"=w549:u32, "Height"=w548:u32)
        n273 = Unbundle(w551) -> ("X"=w526:sgl, "Y"=w550:sgl)
        n274 = Index Array(array=w562) -> (element=w566:T13)  [unwired: 1 in]
        n275 = event shown="[0] \"Remove Button\": Mouse Down" {
          selector: _ -> [_ _ _ _ _ _ _]
          dyn-events: _ -> [_ _ _ _ _ _ _]
          timeout: 10 -> [_ _ _ _ _ _ _]
          event "Remove Button": Mouse Down {
            w601 = 0
            n276 = event-data() -> ()  [unwired: 1 in, 7 out]
            n277 = property on="Image Out" class="ImageControl"() -> ("ROI"=w599:T10)  [unwired: 2 in, 2 out]
            n278 = Unbundle(w599) -> ("Global Rectangle"=w602:i32[], "Contours"=w604:T14)
            n279 = Reverse 1D Array(array=w602) -> (reversed array=w603:i32[])
            n280 = Reverse 1D Array(array=w604) -> (reversed array=w605:T14)
            n281 = Delete From Array(array=w603, index=w601) -> (array with subset deleted=w606:i32[])  [unwired: 1 in, 1 out]
            n282 = Delete From Array(array=w605, index=w601) -> (array with subset deleted=w607:T14)  [unwired: 1 in, 1 out]
            n283 = Reverse 1D Array(array=w606) -> (reversed array=w608:i32[])
            n284 = Reverse 1D Array(array=w607) -> (reversed array=w609:T14)
            n285 = Bundle(w608, w609) -> (w600:T15)  [unwired: 1 in]
            n286 = local write "ROI Descriptor out"(w599) -> ()
            n287 = local write "ROI Descriptor"(w600) -> ()
            n288 = property on="Image Out" class="ImageControl"("ROI"=w600) -> ()  [unwired: 2 in, 2 out]
          }
          event "Undo Button": Mouse Down {
            n289 = event-data() -> ()  [unwired: 1 in, 7 out]
            n290 = invoke on="Image Out" class="ImageControl" method="Clear ROI"() -> ()  [unwired: 3 in, 3 out]
          }
          event "Image Folder": Value Change {
            n291 = event-data() -> ()  [unwired: 1 in, 5 out]
            n292 = local read "Image File"() -> (w611:path)
            n293 = call "Vision Acquisition"("Image Path"=w611) -> ("Image Out"=w610:T2)  [unwired: 25 in, 1 out]
            n294 = local write "Image Out 2"(w610) -> ()
            n295 = local write "Image Out"(w610) -> ()
            n296 = invoke on="Image Out" class="ImageControl" method="Clear ROI"() -> ()  [unwired: 3 in, 3 out]
          }
          event "Zoom": Value Change {
            n297 = event-data() -> ()  [unwired: 1 in, 5 out]
            n298 = local read "Zoom"() -> (w612:i16)
            n299 = Bundle("Zoom"=w612, "Zoom"=w612) -> (w613:cluster{"Zoom":i16, "Zoom":i16})  [unwired: 1 in]
            n300 = property on="Image Out" class="ImageControl"("ZoomInteger"=w613) -> ()  [unwired: 2 in, 2 out]
          }
          event Timeout {
            n301 = event-data() -> ()  [unwired: 1 in, 2 out]
          }
          event "Image Out": Mouse Enter {
            (unwired) 6
            n302 = event-data() -> ()  [unwired: 1 in, 3 out]
            n303 = call "Simulate_Keyboard.vi"("Action"=0, "Virtual Key"=162) -> ()  [unwired: 7 in, 1 out]
          }
          event "Image Out": Mouse Leave {
            n304 = event-data() -> ()  [unwired: 1 in, 3 out]
            n305 = flat-sequence {
              frame #0 {
                n306 = Wait (ms)(milliseconds to wait=10) -> ()  [unwired: 1 out]
              }
              frame #1 {
                (unwired) 6
                n307 = call "Simulate_Keyboard.vi"("Action"=2, "Virtual Key"=162) -> ()  [unwired: 7 in, 1 out]
              }
            }
          }
        }
        n308 = Divide(x=w549, y=w526) -> (x/y=w539:sgl)
        n309 = Multiply(x=w539, y=0.5) -> (x*y=w545:dbl)
        n310 = Divide(x=w548, y=w550) -> (x/y=w538:sgl)
        n311 = Multiply(x=w538, y=0.5) -> (x*y=w544:dbl)
        n312 = Unbundle(w558) -> ("X"=w540:u32, "Y"=w541:u32)
        n313 = Subtract(x=w541, y=w544) -> (x-y=w542:dbl)
        n314 = Subtract(x=w540, y=w545) -> (x-y=w543:dbl)
        n315 = Add(x=w543, y=w539) -> (x+y=w557:dbl)
        n316 = Add(x=w542, y=w538) -> (x+y=w556:dbl)
        n317 = Build Array(w483, w506, w485, w481, w477, w507, w508, w463, w462, w455, w459, w458, w461, w446, w500, w503, w513, w504, w456, w511, w499, w493, w496, w495, w491, w489, w487) -> (w509:string[])
        n318 = local write "Current \nRecord"(w509) -> ()
        n319 = Reciprocal(x=w526) -> (1/x=w525:sgl)
        n320 = event shown="[11] \"Save Changes?\": Mouse Down" {
          selector: _ -> [_ _ _ _ _ _ _ _ _ _ _ _ _ _ _ _]
          dyn-events: _ -> [_ _ _ _ _ _ _ _ _ _ _ _ _ _ _ _]
          timeout: 10 -> [_ _ _ _ _ _ _ _ _ _ _ _ _ _ _ _]
          tunnel: [_ _ _ _ _ _ _ _ _ _ _ _ _ TRUE _ TRUE] -> w583
          event Timeout {
            n321 = event-data() -> ()  [unwired: 1 in, 2 out]
          }
          event "Down Button": Mouse Down {
            w953 = 0
            n322 = event-data() -> ()  [unwired: 1 in, 7 out]
            n323 = local read "Transfer File"() -> (w958:path)
            n324 = Strip Path(path=w958) -> (stripped path=w949:path, name=w967:string)
            n325 = local write "Transfer Folder"(w949) -> ()
            n326 = List Folder(path=w949) -> (filenames=w963:string[], error out=w903:errorcluster)  [unwired: 3 in, 2 out]
            n327 = local read "Folder Index"() -> (w905:dbl)
            n328 = property on="Image Out" class="ImageControl"() -> (error out=w906:errorcluster, "Image Center Position"=w910:cluster{"X":u32, "Y":u32})  [unwired: 2 in, 1 out]
            n329 = Array Size(array=w963) -> (size(s)=w959:i32)
            n330 = Search 1D Array(1D array=w963, element=w967) -> (index of element=w960:i32)  [unwired: 1 in]
            n331 = Decrement(x=w959) -> (x-1=w961:i32)
            n332 = Equal?(x=w960, y=w961) -> (x = y?=w962:bool)
            n333 = invoke on="Image Out" class="ImageControl" method="Clear ROI"() -> ()  [unwired: 3 in, 3 out]
            n334 = case shown="False" w962 {
              tunnel: w905 -> [w1120 _]
              tunnel: [w1119 0] -> w904
              tunnel: w903 -> [w1118 w1121]
              tunnel: [w1118 w1121] -> w902
              frame False {
                n335 = Increment(x=w1120) -> (x+1=w1119:dbl)
              }
              frame True {
              }
            }
            n336 = Unbundle(w910) -> ("X"=w908:u32)  [unwired: 1 out]
            n337 = local write "Folder Index"(w904) -> ()
            n338 = Bundle("X"=w908, 0) -> (w909:cluster{"X":u32, i32})  [unwired: 1 in]
            n339 = property on="Image Out" class="ImageControl"(error in=w906, "Image Center Position"=w909) -> ()  [unwired: 1 in, 2 out]
            n340 = Path To String(path=w949) -> (string=w968:string)
            n341 = Index Array(array=w963, index=w904) -> (element=w964:string)
            n342 = local write "Data Name:"(w964) -> ()
            n343 = Concatenate Strings(w968, "\\", w964) -> (w966:string)
            n344 = String To Path(string=w966) -> (path=w876:path)
            n345 = call "Recorded Values.vi"("Path"=w876) -> ("Recorded Char"=w970:T5, "Recorded Prop"=w971:T6, "Fabrication Prop"=w969:T7)  [unwired: 8 in]
            n346 = Unbundle By Name(w970) -> ("Mobility-Sat"=w983:dbl, "Moblitity-Lin"=w984:dbl, "On/Off"=w985:dbl, "Off Current"=w986:dbl, "Vt-Sat"=w871:dbl, "STS"=w987:dbl, "Trap Density-VT"=w988:dbl, "Trap Density-STS"=w989:dbl)
            n347 = Unbundle By Name(w969) -> ("Date Created"=w990:string, "Material"=w972:string, "Solvent"=w973:string, "Concentration"=w974:dbl, "Method"=w975:string, "Dielectric (nm)"=w976:dbl, "Treatment"=w977:string, "Comments"=w978:string)
            n348 = Unbundle By Name(w971) -> ("Date Recorded"=w979:string, "Index"=w980:string, "Length"=w981:dbl, "Width"=w982:dbl, "Sample Temp"=w873:dbl)
            n349 = local write "Date Created"(w990) -> ()
            n350 = local write "Rec: Off I-Sat"(w986) -> ()
            n351 = local write "Rec: Material"(w972) -> ()
            n352 = local write "Rec: VT-Sat"(w871) -> ()
            n353 = local write "Rec: Concentration"(w974) -> ()
            n354 = local write "Rec: Method"(w975) -> ()
            n355 = local write "Rec: Dielectric (d)"(w976) -> ()
            n356 = local write "Surface Treatment:"(w977) -> ()
            n357 = local write "Comments"(w978) -> ()
            n358 = local write "Index"(w980) -> ()
            n359 = local write "Rec: Mobility-Sat"(w983) -> ()
            n360 = local write "Rec: Mobility-Lin"(w984) -> ()
            n361 = local write "Rec: On/Off"(w985) -> ()
            n362 = local write "Rec: STS"(w987) -> ()
            n363 = local write "Rec: Trap Density-VT"(w988) -> ()
            n364 = local write "Rec: Trap Density-STS"(w989) -> ()
            n365 = local write "Rec: Solvent"(w973) -> ()
            n366 = local write "Date Recorded"(w979) -> ()
            n367 = local write "Rec: Length"(w981) -> ()
            n368 = local write "Rec: Width"(w982) -> ()
            n369 = local write "Rec: Temp"(w873) -> ()
            n370 = Equal To 0?(x=w873) -> (x = 0?=w874:bool)
            n371 = case shown="True" w874 {
              tunnel: [w991 w992] -> w872
              tunnel: w873 -> [w991 _]
              frame False {
              }
              frame True {
                n372 = local read "Room Temp"() -> (w992:dbl)
              }
            }
            n373 = local read "NumPts 2"() -> (w897:dbl)
            n374 = local write "Transfer File"(w876) -> ()
            n375 = local read "NumPts"() -> (w901:dbl)
            n376 = call-poly <vilib>:"Read From Spreadsheet File.vi"("file path (dialog if empty)"=w876) -> ("all rows"=w955:string[][])  [unwired: 6 in, 4 out]
            n377 = call "Mobility-Vt Calculator-File.vi"("NumPts"=w901, "Path"=w876) -> ("XY Graph-Sat"=w899:cluster{dbl[], dbl[]}[], "XY Graph-Lin"=w870:cluster{dbl[], dbl[]}[], "Output"=w900:T8, "Index-Sat"=w898:dbl, "Index-Lin"=w884:dbl)  [unwired: 4 in, 1 out]
            n378 = local read "New: Dielectric"() -> (w881:dbl)
            n379 = call "STS Calculator-File.vi"("NumPts"=w897, "Path"=w876) -> ("STS Index-Sat"=w896:dbl, "XY Graph-Sat"=w895:cluster{dbl[], dbl[]}[], "Ouput"=w894:cluster{"STS-Sat":dbl, "STS-Lin":dbl})  [unwired: 5 in, 2 out]
            n380 = Unbundle By Name(w900) -> ("Mobility-Sat"=w893:dbl, "Vt-Sat"=w880:dbl, "Mobility-Lin"=w892:dbl, "Vt-Lin"=w891:dbl, "Off I-Sat"=w877:dbl, "On/Off I-Sat"=w869:dbl)
            n381 = Unbundle By Name(w894) -> ("STS-Sat"=w875:dbl)  [unwired: 1 out]
            n382 = local write "Index 2"(w896) -> ()
            n383 = local write "XY Graph 2"(w895) -> ()
            n384 = local write "MobVi Index"(w898) -> ()
            n385 = local write "Slide"(w898) -> ()
            n386 = local write "XY Graph"(w899) -> ()
            n387 = Array Size(array=w955) -> (size(s)=w954:i32[])
            n388 = call "Trap Density_VT.vi"("VT"=w880, "Dielectric"=w881) -> ("Trap Density-VT"=w879:dbl)
            n389 = call "Trap Density_STS.vi"("Temp (T) [K]"=w872, "S.T.S. (S)"=w875, "Dielectric"=w881) -> ("Trap Density (N)"=w878:dbl)  [unwired: 8 in]
            n390 = local write "New: STS"(w875) -> ()
            n391 = local write "Calc: STS"(w875) -> ()
            n392 = local write "Calc: Mobility-Sat"(w893) -> ()
            n393 = local write "Calc: Off I-Sat"(w891) -> ()
            n394 = local write "Calc: Mobility-Lin"(w892) -> ()
            n395 = Index Array(array=w954, index=w953) -> (element=w935:i32)
            n396 = Decimate 1D Array(w895) -> (w929:cluster{dbl[], dbl[]}[])  [unwired: 1 out]
            n397 = Decimate 1D Array(w899) -> (w939:cluster{dbl[], dbl[]}[])  [unwired: 1 out]
            n398 = local write "Calc: Off I-Sat"(w877) -> ()
            n399 = local write "Calc: On/Off"(w869) -> ()
            n400 = Decimate 1D Array(w870) -> (w890:cluster{dbl[], dbl[]}[])  [unwired: 1 out]
            n401 = local write "Calc: VT-Sat"(w880) -> ()
            n402 = Array Subset(array=w955, index (row)=w953, index (col)=w953, length (col)=3) -> (w956:string[][])  [unwired: 1 in]
            n403 = local write "Calc: Trap Density-VT"(w879) -> ()
            n404 = local write "Calc: Trap Density-STS"(w878) -> ()
            n405 = local write "New: Trap Density-STS"(w878) -> ()
            n406 = local write "New: Trap Density-VT"(w879) -> ()
            n407 = local write "XY Graph-Lin"(w870) -> ()
            n408 = Array To Cluster(array=w929) -> (cluster=w927:T9)
            n409 = Array To Cluster(array=w939) -> (cluster=w941:T9)
            n410 = local write "New: VT-Lin"(w891) -> ()
            n411 = local write "New: VT-Sat"(w880) -> ()
            n412 = local write "New: Mobility-Sat"(w893) -> ()
            n413 = local write "New: Mobility-Lin"(w892) -> ()
            n414 = Reshape Array(w956, w935) -> (w942:string[])
            n415 = Array To Cluster(array=w890) -> (cluster=w889:T9)
            n416 = Subtract(x=w935, y=20) -> (x-y=w934:i32)
            n417 = property on="Slide" class="Slide (strict)"("Scale.Maximum"=w934) -> ()  [unwired: 2 in, 2 out]
            n418 = Unbundle(w927) -> ("[0]"=w928:cluster{dbl[], dbl[]})  [unwired: 8 out]
            n419 = Unbundle(w941) -> ("[0]"=w940:cluster{dbl[], dbl[]})  [unwired: 8 out]
            n420 = Unbundle(w889) -> ("[0]"=w886:cluster{dbl[], dbl[]})  [unwired: 8 out]
            n421 = Search 1D Array(1D array=w942, element="Index:") -> (index of element=w950:i32)  [unwired: 1 in]
            n422 = local read "NumPts"() -> (w885:dbl)
            n423 = Unbundle(w886) -> (w888:dbl[], w887:dbl[])
            n424 = Increment(x=w950) -> (x+1=w951:i32)
            n425 = Unbundle(w928) -> (w926:dbl[], w925:dbl[])
            n426 = Unbundle(w940) -> (w931:dbl[], w930:dbl[])
            n427 = Array Subset(array=w888, index=w884, length=w885) -> (w883:dbl[])
            n428 = Array Subset(array=w887, index=w884, length=w885) -> (w882:dbl[])
            n429 = Array Subset(array=w926, index=w896, length=w897) -> (w933:dbl[])
            n430 = Array Subset(array=w925, index=w896, length=w897) -> (w932:dbl[])
            n431 = Array Subset(array=w931, index=w898, length=w901) -> (w938:dbl[])
            n432 = Array Subset(array=w930, index=w898, length=w901) -> (w937:dbl[])
            n433 = Index Array(array=w942, index=w951) -> (element=w914:string)
            n434 = local write "Lin-Vg Array-Used"(w883) -> ()
            n435 = local write "Sat Vg Array-Used"(w938) -> ()
            n436 = local write "Vg Array-Log-Used"(w932) -> ()
            n437 = local write "Lin Id-Used"(w882) -> ()
            n438 = local read "Image Folder"() -> (w912:path)
            n439 = local write "Sat Id-Used"(w937) -> ()
            n440 = local write "Sat Id-Log-Used"(w933) -> ()
            n441 = List Folder(path=w912, error in=w902) -> (filenames=w948:string[], error out=w915:errorcluster)  [unwired: 2 in, 2 out]
            n442 = while {
              tunnel: w948 -> [w1005]
              tunnel: w914 -> [w1003]
              tunnel: [w1002] -> _
              tunnel: [w1002] -> w947
              tunnel: w935 -> [w1001]
              i -> [w1002]
              stop <- w998 stop-if-true
              n443 = Index Array(array=w1005, index=w1002) -> (element=w1006:string)
              n444 = xnode "Match Regular Expression"("input string"=w1006, "regular expression"=w1003) -> ("whole match"=w1004:string)  [unwired: 4 in, 4 out]
              n445 = Equal?(x=w1004, y=w1003) -> (x = y?=w1000:bool)
              n446 = Equal?(x=w1001, y=w1002) -> (x = y?=w999:bool)
              n447 = Or(x=w1000, y=w999) -> (x .or. y?=w998:bool)
            }
            n448 = Build Path(base path=w912, name or relative path="ROI") -> (appended path=w911:path)
            n449 = Path To String(path=w912) -> (string=w945:string)
            n450 = Index Array(array=w948, index=w947) -> (element=w923:string)
            n451 = invoke on="Image Out" class="ImageControl" method="Clear ROI"(error in=w915) -> (error out=w918:errorcluster)  [unwired: 2 in, 2 out]
            n452 = local write "Image Name"(w923) -> ()
            n453 = Build Path(base path=w911, name or relative path=w914) -> (appended path=w919:path)
            n454 = call <vilib>:"Check if File or Folder Exists.vi"("error in (no error)"=w918, "path"=w919) -> ("file or folder exists?"=w916:bool, "dup path"=w917:path)  [unwired: 7 in, 1 out]
            n455 = Concatenate Strings(w945, "\\", w923) -> (w944:string)
            n456 = case shown="False" w916 {
              tunnel: w917 -> [_ w993]
              frame False {
              }
              frame True {
                n457 = Read from Text File(file (use dialog)=w993) -> (text=w997:string)  [unwired: 3 in, 3 out]
                n458 = property on="Image Out" class="ImageControl"() -> ("ROI"=w994:T10)  [unwired: 2 in, 2 out]
                n459 = Unflatten From String(type=w994, binary string=w997) -> (value=w995:T10, error out=w996:errorcluster)  [unwired: 3 in, 1 out]
                n460 = property on="Image Out" class="ImageControl"(error in=w996, "ROI"=w995) -> ()  [unwired: 1 in, 2 out]
              }
            }
            n461 = String To Path(string=w944) -> (path=w922:path)
            n462 = Empty String/Path?(string/path=w923) -> (empty?=w924:bool)
            n463 = local read "No Image File"() -> (w920:path)
            n464 = Select(t=w920, s=w924, f=w922) -> (s? t:f=w921:path)
            n465 = local write "Image File"(w921) -> ()
            n466 = call "Vision Acquisition4"("Image Path"=w921) -> ("Image Out"=w946:T2)  [unwired: 25 in, 1 out]
            n467 = local write "Image Out"(w946) -> ()
            n468 = local write "Image Out 2"(w946) -> ()
          }
          event "Transfer File": Value Change {
            w1229 = 0
            n469 = event-data() -> ()  [unwired: 1 in, 5 out]
            n470 = local read "Transfer File"() -> (w1225:path)
            n471 = Strip Path(path=w1225) -> (stripped path=w1224:path, name=w1238:string)
            n472 = local write "Transfer Folder"(w1224) -> ()
            n473 = property on="Image Out" class="ImageControl"() -> (error out=w1180:errorcluster, "Image Center Position"=w1184:cluster{"X":u32, "Y":u32})  [unwired: 2 in, 1 out]
            n474 = List Folder(path=w1224) -> (filenames=w1234:string[], error out=w1190:errorcluster)  [unwired: 3 in, 2 out]
            n475 = Search 1D Array(1D array=w1234, element=w1238) -> (index of element=w1179:i32)  [unwired: 1 in]
            n476 = local write "Folder Index"(w1179) -> ()
            n477 = Unbundle(w1184) -> ("X"=w1182:u32)  [unwired: 1 out]
            n478 = Path To String(path=w1224) -> (string=w1239:string)
            n479 = Index Array(array=w1234, index=w1179) -> (element=w1235:string)
            n480 = Bundle("X"=w1182, 0) -> (w1183:cluster{"X":u32, i32})  [unwired: 1 in]
            n481 = local write "Data Name:"(w1235) -> ()
            n482 = property on="Image Out" class="ImageControl"(error in=w1180, "Image Center Position"=w1183) -> ()  [unwired: 1 in, 2 out]
            n483 = Concatenate Strings(w1239, "\\", w1235) -> (w1237:string)
            n484 = String To Path(string=w1237) -> (path=w1130:path)
            n485 = call "Recorded Values.vi"("Path"=w1130) -> ("Recorded Char"=w1177:T5, "Recorded Prop"=w1176:T6, "Fabrication Prop"=w1178:T7)  [unwired: 8 in]
            n486 = Unbundle By Name(w1177) -> ("Mobility-Sat"=w1164:dbl, "Moblitity-Lin"=w1163:dbl, "On/Off"=w1162:dbl, "Off Current"=w1161:dbl, "Vt-Sat"=w1126:dbl, "STS"=w1160:dbl, "Trap Density-VT"=w1159:dbl, "Trap Density-STS"=w1158:dbl)
            n487 = Unbundle By Name(w1178) -> ("Date Created"=w1157:string, "Material"=w1175:string, "Solvent"=w1174:string, "Concentration"=w1173:dbl, "Method"=w1172:string, "Dielectric (nm)"=w1171:dbl, "Treatment"=w1170:string, "Comments"=w1169:string)
            n488 = Unbundle By Name(w1176) -> ("Date Recorded"=w1168:string, "Index"=w1167:string, "Length"=w1166:dbl, "Width"=w1165:dbl, "Sample Temp"=w1128:dbl)
            n489 = local write "Date Created"(w1157) -> ()
            n490 = local write "Rec: Material"(w1175) -> ()
            n491 = local write "Rec: Off I-Sat"(w1161) -> ()
            n492 = local write "Rec: VT-Sat"(w1126) -> ()
            n493 = local write "Rec: Concentration"(w1173) -> ()
            n494 = local write "Rec: Method"(w1172) -> ()
            n495 = local write "Rec: Dielectric (d)"(w1171) -> ()
            n496 = local write "Surface Treatment:"(w1170) -> ()
            n497 = local write "Comments"(w1169) -> ()
            n498 = local write "Index"(w1167) -> ()
            n499 = local write "Rec: Mobility-Sat"(w1164) -> ()
            n500 = local write "Rec: Mobility-Lin"(w1163) -> ()
            n501 = local write "Rec: On/Off"(w1162) -> ()
            n502 = local write "Rec: STS"(w1160) -> ()
            n503 = local write "Rec: Trap Density-VT"(w1159) -> ()
            n504 = local write "Rec: Trap Density-STS"(w1158) -> ()
            n505 = local write "Rec: Solvent"(w1174) -> ()
            n506 = local write "Date Recorded"(w1168) -> ()
            n507 = local write "Rec: Length"(w1166) -> ()
            n508 = local write "Rec: Width"(w1165) -> ()
            n509 = local write "Rec: Temp"(w1128) -> ()
            n510 = Equal To 0?(x=w1128) -> (x = 0?=w1129:bool)
            n511 = case shown="False" w1129 {
              tunnel: [w1240 w1241] -> w1127
              tunnel: w1128 -> [w1240 _]
              frame False {
              }
              frame True {
                n512 = local read "Room Temp"() -> (w1241:dbl)
              }
            }
            n513 = local write "Transfer File"(w1130) -> ()
            n514 = local read "NumPts 2"() -> (w1152:dbl)
            n515 = local read "NumPts"() -> (w1153:dbl)
            n516 = call-poly <vilib>:"Read From Spreadsheet File.vi"("file path (dialog if empty)"=w1130) -> ("all rows"=w1231:string[][])  [unwired: 6 in, 4 out]
            n517 = local read "New: Dielectric"() -> (w1136:dbl)
            n518 = call "STS Calculator-File.vi"("NumPts"=w1152, "Path"=w1130) -> ("STS Index-Sat"=w1150:dbl, "XY Graph-Sat"=w1151:cluster{dbl[], dbl[]}[], "Ouput"=w1149:cluster{"STS-Sat":dbl, "STS-Lin":dbl})  [unwired: 5 in, 2 out]
            n519 = call "Mobility-Vt Calculator-File.vi"("NumPts"=w1153, "Path"=w1130) -> ("XY Graph-Sat"=w1156:cluster{dbl[], dbl[]}[], "XY Graph-Lin"=w1125:cluster{dbl[], dbl[]}[], "Output"=w1154:T8, "Index-Sat"=w1155:dbl, "Index-Lin"=w1142:dbl)  [unwired: 4 in, 1 out]
            n520 = Unbundle By Name(w1154) -> ("Mobility-Sat"=w1138:dbl, "Vt-Sat"=w1132:dbl, "Mobility-Lin"=w1137:dbl, "Vt-Lin"=w1123:dbl, "Off I-Sat"=w1131:dbl, "On/Off I-Sat"=w1124:dbl)
            n521 = local write "Index 2"(w1150) -> ()
            n522 = local write "XY Graph 2"(w1151) -> ()
            n523 = Unbundle By Name(w1149) -> ("STS-Sat"=w1133:dbl)  [unwired: 1 out]
            n524 = local write "MobVi Index"(w1155) -> ()
            n525 = Array Size(array=w1231) -> (size(s)=w1230:i32[])
            n526 = call "Trap Density_VT.vi"("VT"=w1132, "Dielectric"=w1136) -> ("Trap Density-VT"=w1135:dbl)
            n527 = call "Trap Density_STS.vi"("Temp (T) [K]"=w1127, "S.T.S. (S)"=w1133, "Dielectric"=w1136) -> ("Trap Density (N)"=w1134:dbl)  [unwired: 8 in]
            n528 = local write "Slide"(w1155) -> ()
            n529 = local write "Calc: Mobility-Lin"(w1137) -> ()
            n530 = local write "Calc: Mobility-Sat"(w1138) -> ()
            n531 = local write "Calc: VT-Sat"(w1132) -> ()
            n532 = local write "Calc: Off I-Sat"(w1131) -> ()
            n533 = local write "Calc: VT-Lin"(w1123) -> ()
            n534 = local write "Calc: On/Off"(w1124) -> ()
            n535 = local write "Calc: STS"(w1133) -> ()
            n536 = Decimate 1D Array(w1125) -> (w1148:cluster{dbl[], dbl[]}[])  [unwired: 1 out]
            n537 = local write "Calc: Trap Density-VT"(w1135) -> ()
            n538 = local write "Calc: Trap Density-STS"(w1134) -> ()
            n539 = local write "New: Trap Density-STS"(w1134) -> ()
            n540 = local write "New: Trap Density-VT"(w1135) -> ()
            n541 = local write "XY Graph-Lin"(w1125) -> ()
            n542 = local write "New: VT-Sat"(w1132) -> ()
            n543 = Decimate 1D Array(w1151) -> (w1205:cluster{dbl[], dbl[]}[])  [unwired: 1 out]
            n544 = Index Array(array=w1230, index=w1229) -> (element=w1211:i32)
            n545 = Decimate 1D Array(w1156) -> (w1214:cluster{dbl[], dbl[]}[])  [unwired: 1 out]
            n546 = local write "XY Graph"(w1156) -> ()
            n547 = local write "New: Mobility-Lin"(w1137) -> ()
            n548 = Array Subset(array=w1231, index (row)=w1229, index (col)=w1229, length (col)=3) -> (w1232:string[][])  [unwired: 1 in]
            n549 = local write "New: VT-Lin"(w1123) -> ()
            n550 = Array To Cluster(array=w1148) -> (cluster=w1147:T9)
            n551 = local write "New: STS"(w1133) -> ()
            n552 = local write "New: Mobility-Sat"(w1138) -> ()
            n553 = Array To Cluster(array=w1205) -> (cluster=w1203:T9)
            n554 = Array To Cluster(array=w1214) -> (cluster=w1216:T9)
            n555 = Reshape Array(w1232, w1211) -> (w1217:string[])
            n556 = Subtract(x=w1211, y=20) -> (x-y=w1209:i32)
            n557 = Unbundle(w1147) -> ("[0]"=w1146:cluster{dbl[], dbl[]})  [unwired: 8 out]
            n558 = property on="Slide" class="Slide (strict)"("Scale.Maximum"=w1209) -> ()  [unwired: 2 in, 2 out]
            n559 = local read "NumPts"() -> (w1143:dbl)
            n560 = Unbundle(w1146) -> (w1145:dbl[], w1144:dbl[])
            n561 = Unbundle(w1203) -> ("[0]"=w1204:cluster{dbl[], dbl[]})  [unwired: 8 out]
            n562 = Unbundle(w1216) -> ("[0]"=w1215:cluster{dbl[], dbl[]})  [unwired: 8 out]
            n563 = Search 1D Array(1D array=w1217, element="Index:") -> (index of element=w1226:i32)  [unwired: 1 in]
            n564 = local read "NumPts"() -> (w1139:dbl)
            n565 = Array Subset(array=w1145, index=w1142, length=w1143) -> (w1141:dbl[])
            n566 = Array Subset(array=w1144, index=w1142, length=w1143) -> (w1140:dbl[])
            n567 = Increment(x=w1226) -> (x+1=w1227:i32)
            n568 = Unbundle(w1204) -> (w1201:dbl[], w1200:dbl[])
            n569 = Unbundle(w1215) -> (w1202:dbl[], w1206:dbl[])
            n570 = local read "Image Folder"() -> (w1186:path)
            n571 = local write "Lin-Vg Array-Used"(w1141) -> ()
            n572 = Array Subset(array=w1201, index=w1150, length=w1152) -> (w1208:dbl[])
            n573 = Array Subset(array=w1200, index=w1150, length=w1152) -> (w1207:dbl[])
            n574 = Array Subset(array=w1202, index=w1155, length=w1139) -> (w1213:dbl[])
            n575 = Array Subset(array=w1206, index=w1155, length=w1139) -> (w1212:dbl[])
            n576 = Index Array(array=w1217, index=w1227) -> (element=w1188:string)
            n577 = local write "Lin Id-Used"(w1140) -> ()
            n578 = local write "Sat Vg Array-Used"(w1213) -> ()
            n579 = local write "Vg Array-Log-Used"(w1207) -> ()
            n580 = local write "Sat Id-Log-Used"(w1208) -> ()
            n581 = local write "Sat Id-Used"(w1212) -> ()
            n582 = local write "Index"(w1188) -> ()
            n583 = List Folder(path=w1186, error in=w1190) -> (filenames=w1222:string[], error out=w1189:errorcluster)  [unwired: 2 in, 2 out]
            n584 = Build Path(base path=w1186, name or relative path="ROI") -> (appended path=w1185:path)
            n585 = invoke on="Image Out" class="ImageControl" method="Clear ROI"(error in=w1189) -> (error out=w1193:errorcluster)  [unwired: 2 in, 2 out]
            n586 = Build Path(base path=w1185, name or relative path=w1188) -> (appended path=w1194:path)
            n587 = while {
              tunnel: w1222 -> [w1254]
              tunnel: w1188 -> [w1252]
              tunnel: [w1251] -> _
              tunnel: [w1251] -> w1221
              tunnel: w1211 -> [w1250]
              i -> [w1251]
              stop <- w1247 stop-if-true
              n588 = Index Array(array=w1254, index=w1251) -> (element=w1255:string)
              n589 = xnode "Match Regular Expression"("input string"=w1255, "regular expression"=w1252) -> ("whole match"=w1253:string)  [unwired: 4 in, 4 out]
              n590 = Equal?(x=w1253, y=w1252) -> (x = y?=w1249:bool)
              n591 = Equal?(x=w1250, y=w1251) -> (x = y?=w1248:bool)
              n592 = Or(x=w1249, y=w1248) -> (x .or. y?=w1247:bool)
            }
            n593 = call <vilib>:"Check if File or Folder Exists.vi"("error in (no error)"=w1193, "path"=w1194) -> ("file or folder exists?"=w1191:bool, "dup path"=w1192:path)  [unwired: 7 in, 1 out]
            n594 = case shown="True" w1191 {
              tunnel: w1192 -> [_ w1242]
              frame False {
              }
              frame True {
                n595 = Read from Text File(file (use dialog)=w1242) -> (text=w1246:string)  [unwired: 3 in, 3 out]
                n596 = property on="Image Out" class="ImageControl"() -> ("ROI"=w1243:T10)  [unwired: 2 in, 2 out]
                n597 = Unflatten From String(type=w1243, binary string=w1246) -> (value=w1244:T10, error out=w1245:errorcluster)  [unwired: 3 in, 1 out]
                n598 = property on="Image Out" class="ImageControl"(error in=w1245, "ROI"=w1244) -> ()  [unwired: 1 in, 2 out]
              }
            }
            n599 = invoke on="Image Out" class="ImageControl" method="Clear ROI"() -> ()  [unwired: 3 in, 3 out]
            n600 = Path To String(path=w1186) -> (string=w1220:string)
            n601 = Index Array(array=w1222, index=w1221) -> (element=w1198:string)
            n602 = Concatenate Strings(w1220, "\\", w1198) -> (w1219:string)
            n603 = local write "Image Name"(w1198) -> ()
            n604 = String To Path(string=w1219) -> (path=w1197:path)
            n605 = Empty String/Path?(string/path=w1198) -> (empty?=w1199:bool)
            n606 = local read "No Image File"() -> (w1195:path)
            n607 = Select(t=w1195, s=w1199, f=w1197) -> (s? t:f=w1196:path)
            n608 = local write "Image File"(w1196) -> ()
            n609 = call "Vision Acquisition3"("Image Path"=w1196) -> ("Image Out"=w1223:T2)  [unwired: 25 in, 1 out]
            n610 = local write "Image Out"(w1223) -> ()
            n611 = local write "Image Out 2"(w1223) -> ()
          }
          event "Up Button": Mouse Down {
            w1474 = 0
            n612 = event-data() -> ()  [unwired: 1 in, 5 out]
            n613 = local read "Transfer File"() -> (w1470:path)
            n614 = Strip Path(path=w1470) -> (stripped path=w1469:path, name=w1485:string)
            n615 = local write "Transfer Folder"(w1469) -> ()
            n616 = List Folder(path=w1469) -> (filenames=w1479:string[], error out=w1436:errorcluster)  [unwired: 3 in, 2 out]
            n617 = Array Size(array=w1479) -> (size(s)=w1424:i32)
            n618 = Search 1D Array(1D array=w1479, element=w1485) -> (index of element=w1480:i32)  [unwired: 1 in]
            n619 = Equal To 0?(x=w1480) -> (x = 0?=w1481:bool)
            n620 = local read "Folder Index"() -> (w1423:dbl)
            n621 = property on="Image Out" class="ImageControl"() -> (error out=w1426:errorcluster, "Image Center Position"=w1430:cluster{"X":u32, "Y":u32})  [unwired: 2 in, 1 out]
            n622 = case shown="True" w1481 {
              tunnel: w1423 -> [w1615 _]
              tunnel: [w1614 w1616] -> w1422
              tunnel: w1424 -> [_ w1617]
              frame False {
                n623 = Decrement(x=w1615) -> (x-1=w1614:dbl)
              }
              frame True {
                n624 = Decrement(x=w1617) -> (x-1=w1616:i32)
              }
            }
            n625 = Unbundle(w1430) -> ("X"=w1428:u32)  [unwired: 1 out]
            n626 = local write "Folder Index"(w1422) -> ()
            n627 = Bundle("X"=w1428, 0) -> (w1429:cluster{"X":u32, i32})  [unwired: 1 in]
            n628 = Path To String(path=w1469) -> (string=w1486:string)
            n629 = Index Array(array=w1479, index=w1422) -> (element=w1482:string)
            n630 = local write "Data Name:"(w1482) -> ()
            n631 = property on="Image Out" class="ImageControl"(error in=w1426, "Image Center Position"=w1429) -> ()  [unwired: 1 in, 2 out]
            n632 = Concatenate Strings(w1486, "\\", w1482) -> (w1484:string)
            n633 = String To Path(string=w1484) -> (path=w1373:path)
            n634 = call "Recorded Values.vi"("Path"=w1373) -> ("Recorded Char"=w1420:T5, "Recorded Prop"=w1419:T6, "Fabrication Prop"=w1421:T7)  [unwired: 8 in]
            n635 = Unbundle By Name(w1420) -> ("Mobility-Sat"=w1407:dbl, "Moblitity-Lin"=w1406:dbl, "On/Off"=w1405:dbl, "Off Current"=w1404:dbl, "Vt-Sat"=w1369:dbl, "STS"=w1403:dbl, "Trap Density-VT"=w1402:dbl, "Trap Density-STS"=w1401:dbl)
            n636 = Unbundle By Name(w1421) -> ("Date Created"=w1400:string, "Material"=w1418:string, "Solvent"=w1417:string, "Concentration"=w1416:dbl, "Method"=w1415:string, "Dielectric (nm)"=w1414:dbl, "Treatment"=w1413:string, "Comments"=w1412:string)
            n637 = Unbundle By Name(w1419) -> ("Date Recorded"=w1411:string, "Index"=w1410:string, "Length"=w1409:dbl, "Width"=w1408:dbl, "Sample Temp"=w1370:dbl)
            n638 = local write "Date Created"(w1400) -> ()
            n639 = local write "Rec: Material"(w1418) -> ()
            n640 = local write "Rec: Off I-Sat"(w1404) -> ()
            n641 = local write "Rec: VT-Sat"(w1369) -> ()
            n642 = local write "Rec: Solvent"(w1417) -> ()
            n643 = local write "Rec: Concentration"(w1416) -> ()
            n644 = local write "Rec: Method"(w1415) -> ()
            n645 = local write "Rec: Dielectric (d)"(w1414) -> ()
            n646 = local write "Surface Treatment:"(w1413) -> ()
            n647 = local write "Comments"(w1412) -> ()
            n648 = local write "Index"(w1410) -> ()
            n649 = local write "Rec: Mobility-Sat"(w1407) -> ()
            n650 = local write "Rec: Mobility-Lin"(w1406) -> ()
            n651 = local write "Rec: On/Off"(w1405) -> ()
            n652 = local write "Rec: STS"(w1403) -> ()
            n653 = local write "Rec: Trap Density-VT"(w1402) -> ()
            n654 = local write "Rec: Trap Density-STS"(w1401) -> ()
            n655 = local write "Date Recorded"(w1411) -> ()
            n656 = local write "Rec: Length"(w1409) -> ()
            n657 = local write "Rec: Width"(w1408) -> ()
            n658 = local write "Rec: Temp"(w1370) -> ()
            n659 = Equal To 0?(x=w1370) -> (x = 0?=w1372:bool)
            n660 = case shown="False" w1372 {
              tunnel: [w1487 w1488] -> w1371
              tunnel: w1370 -> [w1487 _]
              frame False {
              }
              frame True {
                n661 = local read "Room Temp"() -> (w1488:dbl)
              }
            }
            n662 = local write "Transfer File"(w1373) -> ()
            n663 = local read "NumPts 2"() -> (w1395:dbl)
            n664 = local read "NumPts"() -> (w1399:dbl)
            n665 = local read "New: Dielectric"() -> (w1379:dbl)
            n666 = call "Mobility-Vt Calculator-File.vi"("NumPts"=w1399, "Path"=w1373) -> ("XY Graph-Sat"=w1397:cluster{dbl[], dbl[]}[], "XY Graph-Lin"=w1368:cluster{dbl[], dbl[]}[], "Output"=w1398:T8, "Index-Sat"=w1396:dbl, "Index-Lin"=w1383:dbl)  [unwired: 4 in, 1 out]
            n667 = call "STS Calculator-File.vi"("NumPts"=w1395, "Path"=w1373) -> ("STS Index-Sat"=w1394:dbl, "XY Graph-Sat"=w1393:cluster{dbl[], dbl[]}[], "Ouput"=w1392:cluster{"STS-Sat":dbl, "STS-Lin":dbl})  [unwired: 5 in, 2 out]
            n668 = call-poly <vilib>:"Read From Spreadsheet File.vi"("file path (dialog if empty)"=w1373) -> ("all rows"=w1476:string[][])  [unwired: 6 in, 4 out]
            n669 = Unbundle By Name(w1398) -> ("Mobility-Sat"=w1382:dbl, "Vt-Sat"=w1375:dbl, "Mobility-Lin"=w1381:dbl, "Vt-Lin"=w1380:dbl, "Off I-Sat"=w1374:dbl, "On/Off I-Sat"=w1367:dbl)
            n670 = Unbundle By Name(w1392) -> ("STS-Sat"=w1376:dbl)  [unwired: 1 out]
            n671 = local write "Index 2"(w1394) -> ()
            n672 = local write "XY Graph 2"(w1393) -> ()
            n673 = local write "MobVi Index"(w1396) -> ()
            n674 = local write "Slide"(w1396) -> ()
            n675 = local write "XY Graph"(w1397) -> ()
            n676 = local write "Calc: Mobility-Sat"(w1382) -> ()
            n677 = local write "Calc: VT-Sat"(w1375) -> ()
            n678 = local write "Calc: Mobility-Lin"(w1381) -> ()
            n679 = local write "Calc: Off I-Sat"(w1374) -> ()
            n680 = local write "Calc: On/Off"(w1367) -> ()
            n681 = Array Size(array=w1476) -> (size(s)=w1475:i32[])
            n682 = local write "Calc: VT-Lin"(w1380) -> ()
            n683 = call "Trap Density_VT.vi"("VT"=w1375, "Dielectric"=w1379) -> ("Trap Density-VT"=w1378:dbl)
            n684 = call "Trap Density_STS.vi"("Temp (T) [K]"=w1371, "S.T.S. (S)"=w1376, "Dielectric"=w1379) -> ("Trap Density (N)"=w1377:dbl)  [unwired: 8 in]
            n685 = local write "Calc: STS"(w1376) -> ()
            n686 = local write "New: STS"(w1376) -> ()
            n687 = Decimate 1D Array(w1368) -> (w1391:cluster{dbl[], dbl[]}[])  [unwired: 1 out]
            n688 = local write "Calc: Trap Density-VT"(w1378) -> ()
            n689 = local write "New: VT-Sat"(w1375) -> ()
            n690 = local write "Calc: Trap Density-STS"(w1377) -> ()
            n691 = local write "New: Trap Density-STS"(w1377) -> ()
            n692 = local write "New: Trap Density-VT"(w1378) -> ()
            n693 = local write "XY Graph-Lin"(w1368) -> ()
            n694 = local write "New: VT-Lin"(w1380) -> ()
            n695 = local write "New: Mobility-Sat"(w1382) -> ()
            n696 = local write "New: Mobility-Lin"(w1381) -> ()
            n697 = Decimate 1D Array(w1393) -> (w1453:cluster{dbl[], dbl[]}[])  [unwired: 1 out]
            n698 = Index Array(array=w1475, index=w1474) -> (element=w1459:i32)
            n699 = Decimate 1D Array(w1397) -> (w1463:cluster{dbl[], dbl[]}[])  [unwired: 1 out]
            n700 = Array To Cluster(array=w1391) -> (cluster=w1390:T9)
            n701 = Array Subset(array=w1476, index (row)=w1474, index (col)=w1474, length (col)=3) -> (w1477:string[][])  [unwired: 1 in]
            n702 = Array To Cluster(array=w1453) -> (cluster=w1451:T9)
            n703 = Array To Cluster(array=w1463) -> (cluster=w1465:T9)
            n704 = Reshape Array(w1477, w1459) -> (w1466:string[])
            n705 = Subtract(x=w1459, y=20) -> (x-y=w1458:i32)
            n706 = Unbundle(w1390) -> ("[0]"=w1387:cluster{dbl[], dbl[]})  [unwired: 8 out]
            n707 = property on="Slide" class="Slide (strict)"("Scale.Maximum"=w1458) -> ()  [unwired: 2 in, 2 out]
            n708 = Unbundle(w1451) -> ("[0]"=w1452:cluster{dbl[], dbl[]})  [unwired: 8 out]
            n709 = Unbundle(w1465) -> ("[0]"=w1464:cluster{dbl[], dbl[]})  [unwired: 8 out]
            n710 = local read "NumPts"() -> (w1384:dbl)
            n711 = Unbundle(w1387) -> (w1386:dbl[], w1385:dbl[])
            n712 = Search 1D Array(1D array=w1466, element="Index:") -> (index of element=w1471:i32)  [unwired: 1 in]
            n713 = Increment(x=w1471) -> (x+1=w1472:i32)
            n714 = Unbundle(w1452) -> (w1450:dbl[], w1449:dbl[])
            n715 = Unbundle(w1464) -> (w1457:dbl[], w1456:dbl[])
            n716 = Array Subset(array=w1386, index=w1383, length=w1384) -> (w1388:dbl[])
            n717 = Array Subset(array=w1385, index=w1383, length=w1384) -> (w1389:dbl[])
            n718 = local read "Image Folder"() -> (w1425:path)
            n719 = local write "Lin-Vg Array-Used"(w1388) -> ()
            n720 = Array Subset(array=w1450, index=w1394, length=w1395) -> (w1455:dbl[])
            n721 = Array Subset(array=w1449, index=w1394, length=w1395) -> (w1454:dbl[])
            n722 = Array Subset(array=w1457, index=w1396, length=w1399) -> (w1462:dbl[])
            n723 = Array Subset(array=w1456, index=w1396, length=w1399) -> (w1461:dbl[])
            n724 = local write "Lin Id-Used"(w1389) -> ()
            n725 = Index Array(array=w1466, index=w1472) -> (element=w1432:string)
            n726 = local write "Sat Vg Array-Used"(w1462) -> ()
            n727 = local write "Vg Array-Log-Used"(w1454) -> ()
            n728 = local write "Sat Id-Log-Used"(w1455) -> ()
            n729 = local write "Sat Id-Used"(w1461) -> ()
            n730 = local write "Index"(w1432) -> ()
            n731 = List Folder(path=w1425, error in=w1436) -> (filenames=w1468:string[], error out=w1435:errorcluster)  [unwired: 2 in, 2 out]
            n732 = Build Path(base path=w1425, name or relative path="ROI") -> (appended path=w1433:path)
            n733 = while {
              tunnel: w1468 -> [w1501]
              tunnel: w1432 -> [w1499]
              tunnel: [w1498] -> w1467
              tunnel: w1459 -> [w1497]
              i -> [w1498]
              stop <- w1494 stop-if-true
              n734 = Index Array(array=w1501, index=w1498) -> (element=w1502:string)
              n735 = xnode "Match Regular Expression"("input string"=w1502, "regular expression"=w1499) -> ("whole match"=w1500:string)  [unwired: 4 in, 4 out]
              n736 = Equal?(x=w1500, y=w1499) -> (x = y?=w1496:bool)
              n737 = Equal?(x=w1497, y=w1498) -> (x = y?=w1495:bool)
              n738 = Or(x=w1496, y=w1495) -> (x .or. y?=w1494:bool)
            }
            n739 = invoke on="Image Out" class="ImageControl" method="Clear ROI"(error in=w1435) -> (error out=w1439:errorcluster)  [unwired: 2 in, 2 out]
            n740 = Build Path(base path=w1433, name or relative path=w1432) -> (appended path=w1431:path)
            n741 = call <vilib>:"Check if File or Folder Exists.vi"("error in (no error)"=w1439, "path"=w1431) -> ("file or folder exists?"=w1437:bool, "dup path"=w1438:path)  [unwired: 7 in, 1 out]
            n742 = case shown="True" w1437 {
              tunnel: w1438 -> [_ w1489]
              frame False {
              }
              frame True {
                n743 = Read from Text File(file (use dialog)=w1489) -> (text=w1493:string)  [unwired: 3 in, 3 out]
                n744 = property on="Image Out" class="ImageControl"() -> ("ROI"=w1490:T10)  [unwired: 2 in, 2 out]
                n745 = Unflatten From String(type=w1490, binary string=w1493) -> (value=w1491:T10, error out=w1492:errorcluster)  [unwired: 3 in, 1 out]
                n746 = property on="Image Out" class="ImageControl"(error in=w1492, "ROI"=w1491) -> ()  [unwired: 1 in, 2 out]
              }
            }
            n747 = Index Array(array=w1468, index=w1467) -> (element=w1441:string)
            n748 = local write "Image Name"(w1441) -> ()
            n749 = Empty String/Path?(string/path=w1441) -> (empty?=w1448:bool)
            n750 = Build Path(base path=w1425, name or relative path=w1441) -> (appended path=w1440:path)
            n751 = local read "No Image File"() -> (w1447:path)
            n752 = Select(t=w1447, s=w1448, f=w1440) -> (s? t:f=w1442:path)
            n753 = call <vilib>:"Get File Extension.vi"("file"=w1442) -> ("lowercase file extension"=w1444:string)  [unwired: 7 in, 3 out]
            n754 = local write "Image File"(w1442) -> ()
            n755 = local write "String"(w1444) -> ()
            n756 = Search 1D Array(1D array=string[] ["bmp", "jpeg", "png", "jpg", "gif"], element=w1444) -> (index of element=w1443:i32)  [unwired: 1 in]
            n757 = call "Vision Acquisition5"("Image Path"=w1442) -> ("Image Out"=w1446:T2)  [unwired: 25 in, 1 out]
            n758 = Less Than 0?(x=w1443) -> ()  [unwired: 1 out]
            n759 = local write "Image Out"(w1446) -> ()
            n760 = local write "Image Out 2"(w1446) -> ()
          }
          event "Save Changes? 3": Mouse Down {
            n761 = event-data() -> ()  [unwired: 1 in, 7 out]
            n762 = local read "Image Folder"() -> (w1618:path)
            n763 = Build Path(base path=w1618, name or relative path="ROI") -> (appended path=w1625:path)
            n764 = call <vilib>:"Check if File or Folder Exists.vi"("path"=w1625) -> ("file or folder exists?"=w1627:bool, "dup path"=w1624:path)  [unwired: 8 in, 1 out]
            n765 = case shown="False" w1627 {
              tunnel: w1624 -> [w1629 w1630]
              tunnel: [w1628 w1630] -> w1619
              frame False {
                n766 = Create Folder(path (use dialog)=w1629) -> (created path=w1628:path)  [unwired: 2 in, 2 out]
              }
              frame True {
              }
            }
            n767 = local read "Index"() -> (w1621:string)
            n768 = property on="Image Out" class="ImageControl"() -> ("ROI"=w1623:T10)  [unwired: 2 in, 2 out]
            n769 = Build Path(base path=w1619, name or relative path=w1621) -> (appended path=w1620:path)
            n770 = Flatten To String(anything=w1623) -> (data string=w1622:string)  [unwired: 3 in, 2 out]
            n771 = Write to Text File(file (use dialog)=w1620, text=w1622) -> ()  [unwired: 2 in, 3 out]
          }
          event "Next Button": Mouse Down {
            n772 = event-data() -> ()  [unwired: 1 in, 5 out]
            n773 = local read "XY Graph"() -> (w1643:cluster{dbl[], dbl[]}[])
            n774 = Decimate 1D Array(w1643) -> (w1639:cluster{dbl[], dbl[]}[], w1638:cluster{dbl[], dbl[]}[])
            n775 = Array To Cluster(array=w1639) -> (cluster=w1649:T9)
            n776 = local read "MobVi Index"() -> (w1645:dbl)
            n777 = Unbundle(w1649) -> ("[0]"=w1648:cluster{dbl[], dbl[]})  [unwired: 8 out]
            n778 = local read "NumPts"() -> (w1644:dbl)
            n779 = Unbundle(w1648) -> (w1647:dbl[], w1646:dbl[])
            n780 = Increment(x=w1645) -> (x+1=w1640:dbl)
            n781 = local read "New: Dielectric"() -> (w1634:dbl)
            n782 = local read "New: Length"() -> (w1633:dbl)
            n783 = local read "New: Width"() -> (w1632:dbl)
            n784 = local write "MobVi Index"(w1640) -> ()
            n785 = Array Subset(array=w1647, index=w1640, length=w1644) -> (w1636:dbl[])
            n786 = Array Subset(array=w1646, index=w1640, length=w1644) -> (w1635:dbl[])
            n787 = local write "Sat Vg Array-Used"(w1636) -> ()
            n788 = local write "Sat Id-Used"(w1635) -> ()
            n789 = call "Mobility-Vt-Used Pts_Saturation.vi"("Width"=w1632, "Length"=w1633, "Dielectric (d)"=w1634, "Sat Id Used"=w1635, "Vg Used"=w1636) -> ("Vt"=w1631:dbl, "Mobility"=w1637:dbl)  [unwired: 4 in, 1 out]
            n790 = Bundle(w1636, w1635) -> (w1642:cluster{dbl[], dbl[]})  [unwired: 1 in]
            n791 = Build Array (concatenate)(w1639, w1638, w1642) -> (w1641:cluster{dbl[], dbl[]}[])
            n792 = local write "New: Mobility-Sat"(w1637) -> ()
            n793 = local write "New: VT-Sat"(w1631) -> ()
            n794 = local write "XY Graph"(w1641) -> ()
          }
          event "Next Button 2": Mouse Down {
            n795 = event-data() -> ()  [unwired: 1 in, 7 out]
            n796 = local read "XY Graph 2"() -> (w1658:cluster{dbl[], dbl[]}[])
            n797 = Decimate 1D Array(w1658) -> (w1654:cluster{dbl[], dbl[]}[], w1653:cluster{dbl[], dbl[]}[])
            n798 = Array To Cluster(array=w1654) -> (cluster=w1664:T9)
            n799 = local read "Index 2"() -> (w1660:dbl)
            n800 = Unbundle(w1664) -> ("[0]"=w1663:cluster{dbl[], dbl[]})  [unwired: 8 out]
            n801 = local read "NumPts 2"() -> (w1659:dbl)
            n802 = Unbundle(w1663) -> (w1662:dbl[], w1661:dbl[])
            n803 = Increment(x=w1660) -> (x+1=w1655:dbl)
            n804 = local write "Index 2"(w1655) -> ()
            n805 = Array Subset(array=w1661, index=w1655, length=w1659) -> (w1650:dbl[])
            n806 = Array Subset(array=w1662, index=w1655, length=w1659) -> (w1651:dbl[])
            n807 = call "STS-Used.vi"("Id Used"=w1651, "Vg-Used"=w1650) -> ("STS"=w1652:dbl)  [unwired: 9 in]
            n808 = Bundle(w1651, w1650) -> (w1657:cluster{dbl[], dbl[]})  [unwired: 1 in]
            n809 = local write "Vg Array-Log-Used"(w1650) -> ()
            n810 = local write "Sat Id-Log-Used"(w1651) -> ()
            n811 = local write "New: STS"(w1652) -> ()
            n812 = Build Array (concatenate)(w1654, w1653, w1657) -> (w1656:cluster{dbl[], dbl[]}[])
            n813 = local write "XY Graph 2"(w1656) -> ()
          }
          event "Previous Button 2": Mouse Down {
            n814 = event-data() -> ()  [unwired: 1 in, 7 out]
            n815 = local read "XY Graph 2"() -> (w1674:cluster{dbl[], dbl[]}[])
            n816 = Decimate 1D Array(w1674) -> (w1671:cluster{dbl[], dbl[]}[], w1670:cluster{dbl[], dbl[]}[])
            n817 = Array To Cluster(array=w1671) -> (cluster=w1679:T9)
            n818 = local read "Index 2"() -> (w1667:dbl)
            n819 = Unbundle(w1679) -> ("[0]"=w1678:cluster{dbl[], dbl[]})  [unwired: 8 out]
            n820 = local read "NumPts 2"() -> (w1675:dbl)
            n821 = Unbundle(w1678) -> (w1677:dbl[], w1676:dbl[])
            n822 = Decrement(x=w1667) -> (x-1=w1668:dbl)
            n823 = local write "Index 2"(w1668) -> ()
            n824 = Array Subset(array=w1677, index=w1668, length=w1675) -> (w1665:dbl[])
            n825 = Array Subset(array=w1676, index=w1668, length=w1675) -> (w1666:dbl[])
            n826 = local write "Vg Array-Log-Used"(w1666) -> ()
            n827 = local write "Sat Id-Log-Used"(w1665) -> ()
            n828 = Bundle(w1665, w1666) -> (w1673:cluster{dbl[], dbl[]})  [unwired: 1 in]
            n829 = call "STS-Used.vi"("Id Used"=w1665, "Vg-Used"=w1666) -> ("STS"=w1669:dbl)  [unwired: 9 in]
            n830 = Build Array (concatenate)(w1671, w1670, w1673) -> (w1672:cluster{dbl[], dbl[]}[])
            n831 = local write "New: STS"(w1669) -> ()
            n832 = local write "XY Graph 2"(w1672) -> ()
          }
          event "Previous Button": Mouse Down {
            n833 = event-data() -> ()  [unwired: 1 in, 5 out]
            n834 = local read "XY Graph"() -> (w1693:cluster{dbl[], dbl[]}[])
            n835 = Decimate 1D Array(w1693) -> (w1690:cluster{dbl[], dbl[]}[], w1689:cluster{dbl[], dbl[]}[])
            n836 = Array To Cluster(array=w1690) -> (cluster=w1698:T9)
            n837 = local read "MobVi Index"() -> (w1688:dbl)
            n838 = Unbundle(w1698) -> ("[0]"=w1697:cluster{dbl[], dbl[]})  [unwired: 8 out]
            n839 = local read "NumPts"() -> (w1694:dbl)
            n840 = Unbundle(w1697) -> (w1696:dbl[], w1695:dbl[])
            n841 = Decrement(x=w1688) -> (x-1=w1687:dbl)
            n842 = local read "New: Dielectric"() -> (w1681:dbl)
            n843 = local read "New: Length"() -> (w1682:dbl)
            n844 = local read "New: Width"() -> (w1683:dbl)
            n845 = local write "MobVi Index"(w1687) -> ()
            n846 = Array Subset(array=w1696, index=w1687, length=w1694) -> (w1686:dbl[])
            n847 = Array Subset(array=w1695, index=w1687, length=w1694) -> (w1685:dbl[])
            n848 = local write "Sat Vg Array-Used"(w1686) -> ()
            n849 = local write "Sat Id-Used"(w1685) -> ()
            n850 = call "Mobility-Vt-Used Pts_Linear.vi"("Width"=w1683, "Length"=w1682, "Dielectric (d)"=w1681, "Sat Id Used"=w1685, "Vg Used"=w1686) -> ("Vt"=w1680:dbl, "Mobility"=w1684:dbl)  [unwired: 4 in, 1 out]
            n851 = Bundle(w1686, w1685) -> (w1692:cluster{dbl[], dbl[]})  [unwired: 1 in]
            n852 = local write "New: VT-Sat"(w1680) -> ()
            n853 = Build Array (concatenate)(w1690, w1689, w1692) -> (w1691:cluster{dbl[], dbl[]}[])
            n854 = local write "New: Mobility-Sat"(w1684) -> ()
            n855 = local write "XY Graph"(w1691) -> ()
          }
          event "Slide": Value Change {
            n856 = event-data() -> ()  [unwired: 1 in, 5 out]
            n857 = local read "XY Graph"() -> (w1711:cluster{dbl[], dbl[]}[])
            n858 = Decimate 1D Array(w1711) -> (w1708:cluster{dbl[], dbl[]}[], w1707:cluster{dbl[], dbl[]}[])
            n859 = Array To Cluster(array=w1708) -> (cluster=w1716:T9)
            n860 = Unbundle(w1716) -> ("[0]"=w1715:cluster{dbl[], dbl[]})  [unwired: 8 out]
            n861 = local read "NumPts"() -> (w1712:dbl)
            n862 = local read "Slide"() -> (w1700:dbl)
            n863 = Unbundle(w1715) -> (w1714:dbl[], w1713:dbl[])
            n864 = local read "New: Dielectric"() -> (w1701:dbl)
            n865 = local read "New: Length"() -> (w1702:dbl)
            n866 = local read "New: Width"() -> (w1703:dbl)
            n867 = local write "MobVi Index"(w1700) -> ()
            n868 = Array Subset(array=w1714, index=w1700, length=w1712) -> (w1706:dbl[])
            n869 = Array Subset(array=w1713, index=w1700, length=w1712) -> (w1705:dbl[])
            n870 = local write "Sat Vg Array-Used"(w1706) -> ()
            n871 = local write "Sat Id-Used"(w1705) -> ()
            n872 = call "Mobility-Vt-Used Pts_Linear.vi"("Width"=w1703, "Length"=w1702, "Dielectric (d)"=w1701, "Sat Id Used"=w1705, "Vg Used"=w1706) -> ("Vt"=w1699:dbl, "Mobility"=w1704:dbl)  [unwired: 4 in, 1 out]
            n873 = Bundle(w1706, w1705) -> (w1710:cluster{dbl[], dbl[]})  [unwired: 1 in]
            n874 = local write "New: VT-Sat"(w1699) -> ()
            n875 = Build Array (concatenate)(w1708, w1707, w1710) -> (w1709:cluster{dbl[], dbl[]}[])
            n876 = local write "New: Mobility-Sat"(w1704) -> ()
            n877 = local write "XY Graph"(w1709) -> ()
          }
          event "Slide 2": Value Change {
            n878 = event-data() -> ()  [unwired: 1 in, 5 out]
            n879 = local read "XY Graph 2"() -> (w1725:cluster{dbl[], dbl[]}[])
            n880 = Decimate 1D Array(w1725) -> (w1722:cluster{dbl[], dbl[]}[], w1721:cluster{dbl[], dbl[]}[])
            n881 = Array To Cluster(array=w1722) -> (cluster=w1730:T9)
            n882 = Unbundle(w1730) -> ("[0]"=w1729:cluster{dbl[], dbl[]})  [unwired: 8 out]
            n883 = local read "NumPts 2"() -> (w1726:dbl)
            n884 = local read "Slide 2"() -> (w1720:dbl)
            n885 = Unbundle(w1729) -> (w1728:dbl[], w1727:dbl[])
            n886 = local write "Index 2"(w1720) -> ()
            n887 = Array Subset(array=w1728, index=w1720, length=w1726) -> (w1718:dbl[])
            n888 = Array Subset(array=w1727, index=w1720, length=w1726) -> (w1717:dbl[])
            n889 = local write "Vg Array-Log-Used"(w1717) -> ()
            n890 = local write "Sat Id-Log-Used"(w1718) -> ()
            n891 = call "STS-Used.vi"("Id Used"=w1718, "Vg-Used"=w1717) -> ("STS"=w1719:dbl)  [unwired: 9 in]
            n892 = Bundle(w1718, w1717) -> (w1724:cluster{dbl[], dbl[]})  [unwired: 1 in]
            n893 = local write "New: STS"(w1719) -> ()
            n894 = Build Array (concatenate)(w1722, w1721, w1724) -> (w1723:cluster{dbl[], dbl[]}[])
            n895 = local write "XY Graph 2"(w1723) -> ()
          }
          event "Save Changes?": Mouse Down {
            n896 = event-data() -> ()  [unwired: 1 in, 5 out]
            n897 = flat-sequence {
              tunnel: [w1758] -> w1735
              tunnel: [w1752] -> w1734
              tunnel: [w1738] -> w1733
              tunnel: w1735 -> [w2070]
              tunnel: w1734 -> [w2067]
              tunnel: [w2068] -> w1732
              tunnel: w1733 -> [w2068]
              tunnel: [w2067] -> w1731
              tunnel: w1732 -> [w2075]
              tunnel: w1731 -> [w2074]
              frame #0 {
                n898 = local read "Transfer File"() -> (w1758:path)
                n899 = local read "New: Temp"() -> (w1739:dbl)
                n900 = local read "New: Length"() -> (w1743:dbl)
                n901 = local read "New: Width"() -> (w1741:dbl)
                n902 = To Single Precision Float(number=w1739) -> (single precision float=w1740:sgl)
                n903 = call-poly <vilib>:"Read From Spreadsheet File.vi"("file path (dialog if empty)"=w1758) -> ("all rows"=w1736:string[][])  [unwired: 6 in, 4 out]
                n904 = Number To Decimal String(number=w1740) -> (decimal integer string=w1755:string)  [unwired: 1 in]
                n905 = To Single Precision Float(number=w1741) -> (single precision float=w1742:sgl)
                n906 = To Single Precision Float(number=w1743) -> (single precision float=w1744:sgl)
                n907 = local read "Index"() -> (w1761:string)
                n908 = Strip Path(path=w1758) -> (stripped path=w1766:path)  [unwired: 1 out]
                n909 = Number To Decimal String(number=w1744) -> (decimal integer string=w1759:string)  [unwired: 1 in]
                n910 = Number To Decimal String(number=w1742) -> (decimal integer string=w1760:string)  [unwired: 1 in]
                n911 = Array Size(array=w1736) -> (size(s)=w1749:i32[])
                n912 = Concatenate Strings("_", w1755, "K") -> (w1753:string)
                n913 = Array Subset(array=w1736, index (row)=0, index (col)=0, length (col)=3) -> (w1745:string[][])  [unwired: 1 in]
                n914 = Index Array(array=w1749, index=0) -> (element=w1751:i32)
                n915 = call "Build Text"("Temp"=w1753, "Index"=w1761, "Length"=w1759, "Width"=w1760) -> ("Result"=w1762:string)  [unwired: 10 in, 1 out]
                n916 = flat-sequence {
                  tunnel: [w2024] -> w1757
                  tunnel: w1757 -> [w2041]
                  frame #0 {
                    # "Makes Empty File for Transformer Data"
                    n917 = local read "Transfer Folder"() -> (w2013:path)
                    n918 = Build Path(base path=w2013, name or relative path="Stats") -> (appended path=w2015:path)
                    n919 = call <vilib>:"Check if File or Folder Exists.vi"("path"=w2015) -> ("file or folder exists?"=w2016:bool, "dup path"=w2017:path)  [unwired: 8 in, 1 out]
                    n920 = case shown="False" w2016 {
                      tunnel: [w2021 w2023] -> w2018
                      tunnel: w2017 -> [w2022 w2023]
                      frame False {
                        n921 = Create Folder(path (use dialog)=w2022) -> (created path=w2021:path)  [unwired: 2 in, 2 out]
                      }
                      frame True {
                      }
                    }
                    n922 = Build Path(base path=w2018, name or relative path="Tranformer Data.txt") -> (appended path=w2020:path)
                    n923 = call-poly <vilib>:"Write To Spreadsheet File.vi"("append to file? (new file:F)"=TRUE, "file path (dialog if empty)"=w2020) -> ()  [unwired: 6 in, 1 out]
                  }
                  frame #1 {
                    # "Adds Headers if they don't exist"
                    n924 = local read "Transfer Folder"() -> (w2030:path)
                    n925 = Concatenate Strings("Stats\\", "Tranformer Data.txt") -> (w2031:string)
                    n926 = Build Path(base path=w2030, name or relative path=w2031) -> (appended path=w2024:path)
                    n927 = call-poly <vilib>:"Read From Spreadsheet File.vi"("file path (dialog if empty)"=w2024) -> ("first row"=w2029:string[])  [unwired: 6 in, 4 out]
                    n928 = Search 1D Array(1D array=w2029, element="DeviceID") -> (index of element=w2027:i32)  [unwired: 1 in]
                    n929 = Equal?(x=w2027, y=0) -> (x = y?=w2025:bool)
                    n930 = case shown="False" w2025 {
                      tunnel: w2024 -> [w2035 _]
                      frame False {
                        n931 = local read "Transformer \nHeaders"() -> (w2034:string[])
                        n932 = call-poly <vilib>:"Write To Spreadsheet File.vi"("1D data"=w2034, "file path (dialog if empty)"=w2035) -> ()  [unwired: 6 in, 1 out]
                      }
                      frame True {
                      }
                    }
                  }
                  frame #2 {
                    # "Adds current device if it doesn't exist"
                    n933 = local read "Current \nRecord"() -> (w2040:string[])
                    n934 = Index Array(array=w2040, index=0) -> (element=w2039:string)
                    n935 = local read "Transfer Folder"() -> (w2043:path)
                    n936 = Concatenate Strings("Stats\\", "Tranformer Data.txt") -> (w2044:string)
                    n937 = local write "Current Device ID"(w2039) -> ()
                    n938 = local read "Current Device ID"() -> (w2049:string)
                    n939 = Build Path(base path=w2043, name or relative path=w2044) -> (appended path=w2042:path)
                    n940 = call-poly <vilib>:"Read From Spreadsheet File.vi"("file path (dialog if empty)"=w2042) -> ("all rows"=w2036:string[][])  [unwired: 6 in, 4 out]
                    n941 = Index Array(array=w2036, index (col)=0) -> (element=w2037:string[])  [unwired: 1 in]
                    n942 = Search 1D Array(1D array=w2037, element=w2049) -> (index of element=w2038:i32)  [unwired: 1 in]
                    n943 = Equal?(x=w2038, y=-1) -> (x = y?=w2051:bool)
                    n944 = case shown="False" w2051 {
                      tunnel: w2041 -> [w2054 w2065]
                      tunnel: w2038 -> [w2057 _]
                      tunnel: w2036 -> [w2058 _]
                      frame False {
                        n945 = local read "Current \nRecord"() -> (w2056:string[])
                        n946 = Replace Array Subset(array=w2058, new element=w2056, index (row)=w2057) -> (w2055:string[][])  [unwired: 1 in]
                        n947 = flat-sequence {
                          tunnel: w2054 -> [w2059]
                          tunnel: w2055 -> [w2060]
                          tunnel: [w2060] -> w2053
                          tunnel: [w2059] -> w2052
                          tunnel: w2053 -> [w2062]
                          tunnel: w2052 -> [w2061]
                          frame #0 {
                            n948 = Delete(path (use dialog)=w2059) -> ()  [unwired: 4 in, 3 out]
                          }
                          frame #1 {
                            n949 = call-poly <vilib>:"Write To Spreadsheet File.vi"("append to file? (new file:F)"=TRUE, "2D data"=w2062, "file path (dialog if empty)"=w2061) -> ()  [unwired: 5 in, 1 out]
                          }
                        }
                      }
                      frame True {
                        n950 = local read "Current \nRecord"() -> (w2064:string[])
                        n951 = call-poly <vilib>:"Write To Spreadsheet File.vi"("append to file? (new file:F)"=TRUE, "1D data"=w2064, "file path (dialog if empty)"=w2065) -> ()  [unwired: 5 in, 1 out]
                      }
                    }
                  }
                }
                n952 = Reshape Array(w1745, w1751) -> (w1737:string[])
                n953 = Path To String(path=w1766) -> (string=w1764:string)
                n954 = stacked-sequence {
                  tunnel: w1737 -> [w1773 w1786 w1804 w1820 w1853 w1871 w1887 w1907 w1925 w1942 w1960 w1978 w1996]
                  tunnel: [_ _ _ _ _ _ _ _ _ _ _ _ w1994] -> w1738
                  frame #0 {
                    n955 = Search 1D Array(1D array=w1773, element="Dielectric (nm):") -> (index of element=w1770:i32)  [unwired: 1 in]
                    n956 = Equal?(x=w1770, y=-1) -> (x = y?=w1769:bool)
                    n957 = local read "Save1 Array"() -> (w1768:string[][])
                    n958 = case shown="False" w1769 {
                      tunnel: w1768 -> [w1779 w1783]
                      tunnel: w1770 -> [w1775 _]
                      tunnel: [w1774 w1783] -> w1767
                      frame False {
                        n959 = local read "New: Dielectric"() -> (w1781:dbl)
                        n960 = Number To Fractional String(number=w1781) -> (F-format string=w1776:string)  [unwired: 3 in]
                        n961 = Divide(x=w1775, y=3) -> (x/y=w1778:dbl)
                        n962 = To Word Integer(number=w1778) -> (16bit integer=w1777:i16)
                        n963 = Replace Array Subset(array=w1779, new element=w1776, index (row)=w1777, index (col)=1) -> (w1774:string[][])
                      }
                      frame True {
                      }
                    }
                    n964 = local write "Save1 Array"(w1767) -> ()
                  }
                  frame #1 {
                    n965 = Search 1D Array(1D array=w1786, element="Length (um):") -> (index of element=w1788:i32)  [unwired: 1 in]
                    n966 = Equal?(x=w1788, y=-1) -> (x = y?=w1787:bool)
                    n967 = local read "Save1 Array"() -> (w1785:string[][])
                    n968 = case shown="False" w1787 {
                      tunnel: w1785 -> [w1798 w1801]
                      tunnel: w1788 -> [w1795 _]
                      tunnel: [w1794 w1801] -> w1784
                      frame False {
                        n969 = local read "New: Length"() -> (w1791:dbl)
                        n970 = Divide(x=w1795, y=3) -> (x/y=w1797:dbl)
                        n971 = Format Value(format string="%#g", value (0)=w1791) -> (output string=w1792:string)  [unwired: 1 in]
                        n972 = To Word Integer(number=w1797) -> (16bit integer=w1796:i16)
                        n973 = Replace Array Subset(array=w1798, new element=w1792, index (row)=w1796, index (col)=1) -> (w1794:string[][])
                      }
                      frame True {
                      }
                    }
                    n974 = local write "Save1 Array"(w1784) -> ()
                  }
                  frame #2 {
                    n975 = Search 1D Array(1D array=w1804, element="Width (um):") -> (index of element=w1806:i32)  [unwired: 1 in]
                    n976 = Equal?(x=w1806, y=-1) -> (x = y?=w1805:bool)
                    n977 = local read "Save1 Array"() -> (w1803:string[][])
                    n978 = case shown="False" w1805 {
                      tunnel: w1806 -> [w1814 _]
                      tunnel: w1803 -> [w1813 w1819]
                      tunnel: [w1812 w1819] -> w1802
                      frame False {
                        n979 = local read "New: Width"() -> (w1809:dbl)
                        n980 = Divide(x=w1814, y=3) -> (x/y=w1816:dbl)
                        n981 = To Word Integer(number=w1816) -> (16bit integer=w1815:i16)
                        n982 = Format Value(format string="%#g", value (0)=w1809) -> (output string=w1810:string)  [unwired: 1 in]
                        n983 = Replace Array Subset(array=w1813, new element=w1810, index (row)=w1815, index (col)=1) -> (w1812:string[][])
                      }
                      frame True {
                      }
                    }
                    n984 = local write "Save1 Array"(w1802) -> ()
                  }
                  frame #3 {
                    n985 = Search 1D Array(1D array=w1820, element="Sample Temp (K):") -> (index of element=w1824:i32)  [unwired: 1 in]
                    n986 = Equal?(x=w1824, y=-1) -> (x = y?=w1823:bool)
                    n987 = local read "Save1 Array"() -> (w1822:string[][])
                    n988 = case shown="True" w1823 {
                      tunnel: w1822 -> [w1834 w1848]
                      tunnel: w1824 -> [w1831 _]
                      tunnel: [w1830 w1847] -> w1821
                      tunnel: w1820 -> [_ w1850]
                      frame False {
                        n989 = local read "New: Temp"() -> (w1828:dbl)
                        n990 = Divide(x=w1831, y=3) -> (x/y=w1833:dbl)
                        n991 = Format Value(format string="%#g", value (0)=w1828) -> (output string=w1827:string)  [unwired: 1 in]
                        n992 = To Word Integer(number=w1833) -> (16bit integer=w1832:i16)
                        n993 = Replace Array Subset(array=w1834, new element=w1827, index (row)=w1832, index (col)=1) -> (w1830:string[][])
                      }
                      frame True {
                        n994 = local read "New: Temp"() -> (w1838:dbl)
                        n995 = Search 1D Array(1D array=w1850, element="Width (um):") -> (index of element=w1844:i32)  [unwired: 1 in]
                        n996 = Divide(x=w1844, y=3) -> (x/y=w1845:dbl)
                        n997 = To Word Integer(number=w1845) -> (16bit integer=w1843:i16)
                        n998 = Format Value(format string="%#g", value (0)=w1838) -> (output string=w1837:string)  [unwired: 1 in]
                        n999 = Build Array("Sample Temp (K):", w1837) -> (w1840:string[])
                        n1000 = Increment(x=w1843) -> (x+1=w1842:i16)
                        n1001 = Insert Into Array(array=w1848, index (row)=w1842, new element=w1840) -> (w1847:string[][])  [unwired: 1 in]
                      }
                    }
                    n1002 = local write "Save1 Array"(w1821) -> ()
                  }
                  frame #4 {
                    n1003 = Search 1D Array(1D array=w1853, element="Mobility-Sat (cm^2/Vs):") -> (index of element=w1855:i32)  [unwired: 1 in]
                    n1004 = Equal?(x=w1855, y=-1) -> (x = y?=w1854:bool)
                    n1005 = local read "Save1 Array"() -> (w1851:string[][])
                    n1006 = case shown="False" w1854 {
                      tunnel: w1851 -> [w1865 w1868]
                      tunnel: w1855 -> [w1862 _]
                      tunnel: [w1861 w1868] -> w1852
                      frame False {
                        n1007 = local read "New: Mobility-Sat"() -> (w1858:dbl)
                        n1008 = Divide(x=w1862, y=3) -> (x/y=w1864:dbl)
                        n1009 = To Word Integer(number=w1864) -> (16bit integer=w1863:i16)
                        n1010 = Format Value(format string="%#g", value (0)=w1858) -> (output string=w1859:string)  [unwired: 1 in]
                        n1011 = Replace Array Subset(array=w1865, new element=w1859, index (row)=w1863, index (col)=1) -> (w1861:string[][])
                      }
                      frame True {
                      }
                    }
                    n1012 = local write "Save1 Array"(w1852) -> ()
                  }
                  frame #5 {
                    n1013 = Search 1D Array(1D array=w1871, element="On/Off I-Sat:") -> (index of element=w1873:i32)  [unwired: 1 in]
                    n1014 = Equal?(x=w1873, y=-1) -> (x = y?=w1872:bool)
                    n1015 = local read "Save1 Array"() -> (w1870:string[][])
                    n1016 = case shown="False" w1872 {
                      tunnel: w1870 -> [w1883 w1886]
                      tunnel: w1873 -> [w1880 _]
                      tunnel: [w1879 w1886] -> w1869
                      frame False {
                        n1017 = local read "Calc: On/Off"() -> (w1876:dbl)
                        n1018 = Divide(x=w1880, y=3) -> (x/y=w1882:dbl)
                        n1019 = To Word Integer(number=w1882) -> (16bit integer=w1881:i16)
                        n1020 = Format Value(format string="%#g", value (0)=w1876) -> (output string=w1877:string)  [unwired: 1 in]
                        n1021 = Replace Array Subset(array=w1883, new element=w1877, index (row)=w1881, index (col)=1) -> (w1879:string[][])
                      }
                      frame True {
                      }
                    }
                    n1022 = local write "Save1 Array"(w1869) -> ()
                  }
                  frame #6 {
                    n1023 = Search 1D Array(1D array=w1887, element="Mobility-Lin (cm^2/Vs):") -> (index of element=w1891:i32)  [unwired: 1 in]
                    n1024 = Equal?(x=w1891, y=-1) -> (x = y?=w1890:bool)
                    n1025 = local read "Save1 Array"() -> (w1889:string[][])
                    n1026 = case shown="False" w1890 {
                      tunnel: w1889 -> [w1901 w1904]
                      tunnel: w1891 -> [w1898 _]
                      tunnel: [w1897 w1904] -> w1888
                      frame False {
                        n1027 = local read "Calc: Mobility-Lin"() -> (w1894:dbl)
                        n1028 = Divide(x=w1898, y=3) -> (x/y=w1900:dbl)
                        n1029 = To Word Integer(number=w1900) -> (16bit integer=w1899:i16)
                        n1030 = Format Value(format string="%#g", value (0)=w1894) -> (output string=w1895:string)  [unwired: 1 in]
                        n1031 = Replace Array Subset(array=w1901, new element=w1895, index (row)=w1899, index (col)=1) -> (w1897:string[][])
                      }
                      frame True {
                      }
                    }
                    n1032 = local write "Save1 Array"(w1888) -> ()
                  }
                  frame #7 {
                    n1033 = Search 1D Array(1D array=w1907, element="Off I-Sat (A):") -> (index of element=w1909:i32)  [unwired: 1 in]
                    n1034 = Equal?(x=w1909, y=-1) -> (x = y?=w1908:bool)
                    n1035 = local read "Save1 Array"() -> (w1906:string[][])
                    n1036 = case shown="False" w1908 {
                      tunnel: w1906 -> [w1919 w1922]
                      tunnel: w1909 -> [w1916 _]
                      tunnel: [w1915 w1922] -> w1905
                      frame False {
                        n1037 = local read "Calc: Off I-Sat"() -> (w1914:dbl)
                        n1038 = Divide(x=w1916, y=3) -> (x/y=w1918:dbl)
                        n1039 = Format Value(format string="%#g", value (0)=w1914) -> (output string=w1912:string)  [unwired: 1 in]
                        n1040 = To Word Integer(number=w1918) -> (16bit integer=w1917:i16)
                        n1041 = Replace Array Subset(array=w1919, new element=w1912, index (row)=w1917, index (col)=1) -> (w1915:string[][])
                      }
                      frame True {
                      }
                    }
                    n1042 = local write "Save1 Array"(w1905) -> ()
                  }
                  frame #8 {
                    n1043 = Search 1D Array(1D array=w1925, element="Vt-Sat (V):") -> (index of element=w1927:i32)  [unwired: 1 in]
                    n1044 = Equal?(x=w1927, y=-1) -> (x = y?=w1926:bool)
                    n1045 = local read "Save1 Array"() -> (w1924:string[][])
                    n1046 = case shown="False" w1926 {
                      tunnel: w1924 -> [w1935 w1939]
                      tunnel: w1927 -> [w1931 _]
                      tunnel: [w1930 w1939] -> w1923
                      frame False {
                        n1047 = local read "New: VT-Sat"() -> (w1937:dbl)
                        n1048 = Number To Fractional String(number=w1937) -> (F-format string=w1932:string)  [unwired: 3 in]
                        n1049 = Divide(x=w1931, y=3) -> (x/y=w1934:dbl)
                        n1050 = To Word Integer(number=w1934) -> (16bit integer=w1933:i16)
                        n1051 = Replace Array Subset(array=w1935, new element=w1932, index (row)=w1933, index (col)=1) -> (w1930:string[][])
                      }
                      frame True {
                      }
                    }
                    n1052 = local write "Save1 Array"(w1923) -> ()
                  }
                  frame #9 {
                    n1053 = Search 1D Array(1D array=w1942, element="VT-Lin (V):") -> (index of element=w1944:i32)  [unwired: 1 in]
                    n1054 = Equal?(x=w1944, y=-1) -> (x = y?=w1943:bool)
                    n1055 = local read "Save1 Array"() -> (w1941:string[][])
                    n1056 = case shown="False" w1943 {
                      tunnel: w1941 -> [w1954 w1957]
                      tunnel: w1944 -> [w1951 _]
                      tunnel: [w1950 w1957] -> w1940
                      frame False {
                        n1057 = local read "New: VT-Lin"() -> (w1948:dbl)
                        n1058 = Divide(x=w1951, y=3) -> (x/y=w1953:dbl)
                        n1059 = Format Value(format string="%#g", value (0)=w1948) -> (output string=w1947:string)  [unwired: 1 in]
                        n1060 = To Word Integer(number=w1953) -> (16bit integer=w1952:i16)
                        n1061 = Replace Array Subset(array=w1954, new element=w1947, index (row)=w1952, index (col)=1) -> (w1950:string[][])
                      }
                      frame True {
                      }
                    }
                    n1062 = local write "Save1 Array"(w1940) -> ()
                  }
                  frame #10 {
                    n1063 = Search 1D Array(1D array=w1960, element="STS-Sat (V/decade):") -> (index of element=w1962:i32)  [unwired: 1 in]
                    n1064 = Equal?(x=w1962, y=-1) -> (x = y?=w1961:bool)
                    n1065 = local read "Save1 Array"() -> (w1959:string[][])
                    n1066 = case shown="False" w1961 {
                      tunnel: w1959 -> [w1972 w1975]
                      tunnel: w1962 -> [w1969 _]
                      tunnel: [w1968 w1975] -> w1958
                      frame False {
                        n1067 = local read "New: STS"() -> (w1966:dbl)
                        n1068 = Divide(x=w1969, y=3) -> (x/y=w1971:dbl)
                        n1069 = Format Value(format string="%#g", value (0)=w1966) -> (output string=w1965:string)  [unwired: 1 in]
                        n1070 = To Word Integer(number=w1971) -> (16bit integer=w1970:i16)
                        n1071 = Replace Array Subset(array=w1972, new element=w1965, index (row)=w1970, index (col)=1) -> (w1968:string[][])
                      }
                      frame True {
                      }
                    }
                    n1072 = local write "Save1 Array"(w1958) -> ()
                  }
                  frame #11 {
                    n1073 = Search 1D Array(1D array=w1978, element="Trap Density-VT (Traps/Vcm^2):") -> (index of element=w1980:i32)  [unwired: 1 in]
                    n1074 = Equal?(x=w1980, y=-1) -> (x = y?=w1979:bool)
                    n1075 = local read "Save1 Array"() -> (w1977:string[][])
                    n1076 = case shown="False" w1979 {
                      tunnel: w1977 -> [w1990 w1993]
                      tunnel: w1980 -> [w1986 _]
                      tunnel: [w1985 w1993] -> w1976
                      frame False {
                        n1077 = local read "New: Trap Density-VT"() -> (w1984:dbl)
                        n1078 = Format Value(format string="%#g", value (0)=w1984) -> (output string=w1987:string)  [unwired: 1 in]
                        n1079 = Divide(x=w1986, y=3) -> (x/y=w1989:dbl)
                        n1080 = To Word Integer(number=w1989) -> (16bit integer=w1988:i16)
                        n1081 = Replace Array Subset(array=w1990, new element=w1987, index (row)=w1988, index (col)=1) -> (w1985:string[][])
                      }
                      frame True {
                      }
                    }
                    n1082 = local write "Save1 Array"(w1976) -> ()
                  }
                  frame #12 {
                    n1083 = Search 1D Array(1D array=w1996, element="Trap Density-STS (Traps/Vcm^2):") -> (index of element=w1998:i32)  [unwired: 1 in]
                    n1084 = Equal?(x=w1998, y=-1) -> (x = y?=w1997:bool)
                    n1085 = local read "Save1 Array"() -> (w1995:string[][])
                    n1086 = case shown="False" w1997 {
                      tunnel: w1995 -> [w2008 w2011]
                      tunnel: w1998 -> [w2005 _]
                      tunnel: [w2004 w2011] -> w1994
                      frame False {
                        n1087 = local read "New: Trap Density-STS"() -> (w2002:dbl)
                        n1088 = Divide(x=w2005, y=3) -> (x/y=w2007:dbl)
                        n1089 = To Word Integer(number=w2007) -> (16bit integer=w2006:i16)
                        n1090 = Format Value(format string="%#g", value (0)=w2002) -> (output string=w2001:string)  [unwired: 1 in]
                        n1091 = Replace Array Subset(array=w2008, new element=w2001, index (row)=w2006, index (col)=1) -> (w2004:string[][])
                      }
                      frame True {
                      }
                    }
                    n1092 = local write "Save1 Array"(w1994) -> ()
                  }
                }
                n1093 = Concatenate Strings(w1764, "\\", w1762) -> (w1763:string)
                n1094 = String To Path(string=w1763) -> (path=w1752:path)
                n1095 = local write "Save1 Array"(w1736) -> ()
              }
              frame #1 {
                n1096 = Equal?(x=w2070, y=w2067) -> (x = y?=w2069:bool)
                n1097 = case shown="False" w2069 {
                  tunnel: w2070 -> [w2073 _]
                  tunnel: w2067 -> [w2072 _]
                  frame False {
                    n1098 = Move(source path=w2073, 9:TRUE, 10:w2072) -> ()  [unwired: 2 in, 3 out]
                  }
                  frame True {
                  }
                }
              }
              frame #2 {
                n1099 = local write "Transfer File"(w2074) -> ()
                n1100 = call-poly <vilib>:"Write To Spreadsheet File.vi"("2D data"=w2075, "file path (dialog if empty)"=w2074) -> ()  [unwired: 6 in, 1 out]
              }
            }
          }
          event "Save Changes? 2": Mouse Down {
            n1101 = event-data() -> ()  [unwired: 1 in, 5 out]
            n1102 = stacked-sequence {
              seq-local: [w2135 _ _ _ _] -> [_ w2387 _ _ _]
              seq-local: [w2138 _ _ _ _] -> [_ w2388 _ _ _]
              seq-local: [w2135 _ _ _ _] -> [_ w2386 _ _ _]
              seq-local: [w2133 _ _ _ _] -> [_ w2384 _ _ _]
              seq-local: [_ w2388 _ _ _] -> [_ _ w2393 _ _]
              seq-local: [_ w2384 _ _ _] -> [_ _ w2392 _ _]
              frame #0 {
                n1103 = local read "Transfer File"() -> (w2138:path)
                n1104 = local read "New: Temp"() -> (w2137:dbl)
                n1105 = local read "New: Length"() -> (w2141:dbl)
                n1106 = local read "New: Width"() -> (w2139:dbl)
                n1107 = To Word Integer(number=w2137) -> (16bit integer=w2136:i16)
                n1108 = call-poly <vilib>:"Read From Spreadsheet File.vi"("file path (dialog if empty)"=w2138) -> ("all rows"=w2132:string[][])  [unwired: 6 in, 4 out]
                n1109 = Number To Decimal String(number=w2136) -> (decimal integer string=w2152:string)  [unwired: 1 in]
                n1110 = To Single Precision Float(number=w2139) -> (single precision float=w2140:sgl)
                n1111 = To Single Precision Float(number=w2141) -> (single precision float=w2142:sgl)
                n1112 = local read "Index"() -> (w2156:string)
                n1113 = Strip Path(path=w2138) -> (stripped path=w2161:path)  [unwired: 1 out]
                n1114 = Number To Decimal String(number=w2142) -> (decimal integer string=w2154:string)  [unwired: 1 in]
                n1115 = Number To Decimal String(number=w2140) -> (decimal integer string=w2155:string)  [unwired: 1 in]
                n1116 = Array Size(array=w2132) -> (size(s)=w2147:i32[])
                n1117 = Concatenate Strings("_", w2152, "K") -> (w2150:string)
                n1118 = Array Subset(array=w2132, index (row)=0, index (col)=0, length (col)=3) -> (w2143:string[][])  [unwired: 1 in]
                n1119 = Index Array(array=w2147, index=0) -> (element=w2149:i32)
                n1120 = call "Build Text2"("Temp"=w2150, "Index"=w2156, "Length"=w2154, "Width"=w2155) -> ("Result"=w2157:string)  [unwired: 10 in, 1 out]
                n1121 = Reshape Array(w2143, w2149) -> (w2134:string[])
                n1122 = Path To String(path=w2161) -> (string=w2159:string)
                n1123 = stacked-sequence {
                  tunnel: w2134 -> [w2168 w2181 w2198 w2215 w2232 w2249 w2264 w2283 w2301 w2318 w2335 w2352 w2369]
                  tunnel: [_ _ _ _ _ _ _ _ _ _ _ _ w2367] -> w2133
                  frame #0 {
                    n1124 = Search 1D Array(1D array=w2168, element="Dielectric (nm):") -> (index of element=w2165:i32)  [unwired: 1 in]
                    n1125 = Equal?(x=w2165, y=-1) -> (x = y?=w2164:bool)
                    n1126 = local read "Save1 Array"() -> (w2163:string[][])
                    n1127 = case shown="False" w2164 {
                      tunnel: w2163 -> [w2174 w2178]
                      tunnel: w2165 -> [w2170 _]
                      tunnel: [w2169 w2178] -> w2162
                      frame False {
                        n1128 = local read "New: Dielectric"() -> (w2176:dbl)
                        n1129 = Number To Fractional String(number=w2176) -> (F-format string=w2171:string)  [unwired: 3 in]
                        n1130 = Divide(x=w2170, y=3) -> (x/y=w2173:dbl)
                        n1131 = To Word Integer(number=w2173) -> (16bit integer=w2172:i16)
                        n1132 = Replace Array Subset(array=w2174, new element=w2171, index (row)=w2172, index (col)=1) -> (w2169:string[][])
                      }
                      frame True {
                      }
                    }
                    n1133 = local write "Save1 Array"(w2162) -> ()
                  }
                  frame #1 {
                    n1134 = Search 1D Array(1D array=w2181, element="Length (um):") -> (index of element=w2183:i32)  [unwired: 1 in]
                    n1135 = Equal?(x=w2183, y=-1) -> (x = y?=w2182:bool)
                    n1136 = local read "Save1 Array"() -> (w2180:string[][])
                    n1137 = case shown="True" w2182 {
                      tunnel: w2180 -> [w2191 w2195]
                      tunnel: w2183 -> [w2187 _]
                      tunnel: [w2186 w2195] -> w2179
                      frame False {
                        n1138 = local read "New: Length"() -> (w2193:dbl)
                        n1139 = Number To Fractional String(number=w2193) -> (F-format string=w2188:string)  [unwired: 3 in]
                        n1140 = Divide(x=w2187, y=3) -> (x/y=w2190:dbl)
                        n1141 = To Word Integer(number=w2190) -> (16bit integer=w2189:i16)
                        n1142 = Replace Array Subset(array=w2191, new element=w2188, index (row)=w2189, index (col)=1) -> (w2186:string[][])
                      }
                      frame True {
                      }
                    }
                    n1143 = local write "Save1 Array"(w2179) -> ()
                  }
                  frame #2 {
                    n1144 = Search 1D Array(1D array=w2198, element="Width (um):") -> (index of element=w2200:i32)  [unwired: 1 in]
                    n1145 = Equal?(x=w2200, y=-1) -> (x = y?=w2199:bool)
                    n1146 = local read "Save1 Array"() -> (w2197:string[][])
                    n1147 = case shown="False" w2199 {
                      tunnel: w2200 -> [w2205 _]
                      tunnel: w2197 -> [w2204 w2212]
                      tunnel: [w2203 w2212] -> w2196
                      frame False {
                        n1148 = local read "New: Width"() -> (w2210:dbl)
                        n1149 = Number To Fractional String(number=w2210) -> (F-format string=w2206:string)  [unwired: 3 in]
                        n1150 = Divide(x=w2205, y=3) -> (x/y=w2208:dbl)
                        n1151 = To Word Integer(number=w2208) -> (16bit integer=w2207:i16)
                        n1152 = Replace Array Subset(array=w2204, new element=w2206, index (row)=w2207, index (col)=1) -> (w2203:string[][])
                      }
                      frame True {
                      }
                    }
                    n1153 = local write "Save1 Array"(w2196) -> ()
                  }
                  frame #3 {
                    n1154 = Search 1D Array(1D array=w2215, element="Sample Temp (K):") -> (index of element=w2217:i32)  [unwired: 1 in]
                    n1155 = Equal?(x=w2217, y=-1) -> (x = y?=w2216:bool)
                    n1156 = local read "Save1 Array"() -> (w2214:string[][])
                    n1157 = case shown="False" w2216 {
                      tunnel: w2214 -> [w2225 w2229]
                      tunnel: w2217 -> [w2221 _]
                      tunnel: [w2220 w2229] -> w2213
                      frame False {
                        n1158 = local read "New: Temp"() -> (w2227:dbl)
                        n1159 = Number To Fractional String(number=w2227) -> (F-format string=w2222:string)  [unwired: 3 in]
                        n1160 = Divide(x=w2221, y=3) -> (x/y=w2224:dbl)
                        n1161 = To Word Integer(number=w2224) -> (16bit integer=w2223:i16)
                        n1162 = Replace Array Subset(array=w2225, new element=w2222, index (row)=w2223, index (col)=1) -> (w2220:string[][])
                      }
                      frame True {
                      }
                    }
                    n1163 = local write "Save1 Array"(w2213) -> ()
                  }
                  frame #4 {
                    n1164 = Search 1D Array(1D array=w2232, element="Mobility-Sat (cm^2/Vs):") -> (index of element=w2234:i32)  [unwired: 1 in]
                    n1165 = Equal?(x=w2234, y=-1) -> (x = y?=w2233:bool)
                    n1166 = local read "Save1 Array"() -> (w2230:string[][])
                    n1167 = case shown="False" w2233 {
                      tunnel: w2230 -> [w2242 w2246]
                      tunnel: w2234 -> [w2238 _]
                      tunnel: [w2237 w2246] -> w2231
                      frame False {
                        n1168 = local read "New: Mobility-Sat"() -> (w2244:dbl)
                        n1169 = Number To Fractional String(number=w2244) -> (F-format string=w2239:string)  [unwired: 3 in]
                        n1170 = Divide(x=w2238, y=3) -> (x/y=w2241:dbl)
                        n1171 = To Word Integer(number=w2241) -> (16bit integer=w2240:i16)
                        n1172 = Replace Array Subset(array=w2242, new element=w2239, index (row)=w2240, index (col)=1) -> (w2237:string[][])
                      }
                      frame True {
                      }
                    }
                    n1173 = local write "Save1 Array"(w2231) -> ()
                  }
                  frame #5 {
                    n1174 = Search 1D Array(1D array=w2249, element="Mobility-Lin (cm^2/Vs):") -> (index of element=w2251:i32)  [unwired: 1 in]
                    n1175 = Equal?(x=w2251, y=-1) -> (x = y?=w2250:bool)
                    n1176 = local read "Save1 Array"() -> (w2248:string[][])
                    n1177 = case shown="False" w2250 {
                      tunnel: w2248 -> [w2259 w2263]
                      tunnel: w2251 -> [w2255 _]
                      tunnel: [w2254 w2263] -> w2247
                      frame False {
                        n1178 = local read "Calc: Mobility-Lin"() -> (w2261:dbl)
                        n1179 = Number To Fractional String(number=w2261) -> (F-format string=w2256:string)  [unwired: 3 in]
                        n1180 = Divide(x=w2255, y=3) -> (x/y=w2258:dbl)
                        n1181 = To Word Integer(number=w2258) -> (16bit integer=w2257:i16)
                        n1182 = Replace Array Subset(array=w2259, new element=w2256, index (row)=w2257, index (col)=1) -> (w2254:string[][])
                      }
                      frame True {
                      }
                    }
                    n1183 = local write "Save1 Array"(w2247) -> ()
                  }
                  frame #6 {
                    n1184 = Search 1D Array(1D array=w2264, element="On/Off I-Sat:") -> (index of element=w2268:i32)  [unwired: 1 in]
                    n1185 = Equal?(x=w2268, y=-1) -> (x = y?=w2267:bool)
                    n1186 = local read "Save1 Array"() -> (w2266:string[][])
                    n1187 = case shown="False" w2267 {
                      tunnel: w2266 -> [w2276 w2280]
                      tunnel: w2268 -> [w2272 _]
                      tunnel: [w2271 w2280] -> w2265
                      frame False {
                        n1188 = local read "Calc: On/Off"() -> (w2278:dbl)
                        n1189 = Number To Fractional String(number=w2278) -> (F-format string=w2273:string)  [unwired: 3 in]
                        n1190 = Divide(x=w2272, y=3) -> (x/y=w2275:dbl)
                        n1191 = To Word Integer(number=w2275) -> (16bit integer=w2274:i16)
                        n1192 = Replace Array Subset(array=w2276, new element=w2273, index (row)=w2274, index (col)=1) -> (w2271:string[][])
                      }
                      frame True {
                      }
                    }
                    n1193 = local write "Save1 Array"(w2265) -> ()
                  }
                  frame #7 {
                    n1194 = Search 1D Array(1D array=w2283, element="Off I-Sat (A):") -> (index of element=w2285:i32)  [unwired: 1 in]
                    n1195 = Equal?(x=w2285, y=-1) -> (x = y?=w2284:bool)
                    n1196 = local read "Save1 Array"() -> (w2282:string[][])
                    n1197 = case shown="False" w2284 {
                      tunnel: w2282 -> [w2295 w2298]
                      tunnel: w2285 -> [w2292 _]
                      tunnel: [w2291 w2298] -> w2281
                      frame False {
                        n1198 = local read "Calc: Off I-Sat"() -> (w2290:dbl)
                        n1199 = Format Value(format string="%#g", value (0)=w2290) -> (output string=w2289:string)  [unwired: 1 in]
                        n1200 = Divide(x=w2292, y=3) -> (x/y=w2294:dbl)
                        n1201 = To Word Integer(number=w2294) -> (16bit integer=w2293:i16)
                        n1202 = Replace Array Subset(array=w2295, new element=w2289, index (row)=w2293, index (col)=1) -> (w2291:string[][])
                      }
                      frame True {
                      }
                    }
                    n1203 = local write "Save1 Array"(w2281) -> ()
                  }
                  frame #8 {
                    n1204 = Search 1D Array(1D array=w2301, element="Vt-Sat (V):") -> (index of element=w2303:i32)  [unwired: 1 in]
                    n1205 = Equal?(x=w2303, y=-1) -> (x = y?=w2302:bool)
                    n1206 = local read "Save1 Array"() -> (w2300:string[][])
                    n1207 = case shown="False" w2302 {
                      tunnel: w2300 -> [w2311 w2315]
                      tunnel: w2303 -> [w2307 _]
                      tunnel: [w2306 w2315] -> w2299
                      frame False {
                        n1208 = local read "New: VT-Sat"() -> (w2313:dbl)
                        n1209 = Number To Fractional String(number=w2313) -> (F-format string=w2308:string)  [unwired: 3 in]
                        n1210 = Divide(x=w2307, y=3) -> (x/y=w2310:dbl)
                        n1211 = To Word Integer(number=w2310) -> (16bit integer=w2309:i16)
                        n1212 = Replace Array Subset(array=w2311, new element=w2308, index (row)=w2309, index (col)=1) -> (w2306:string[][])
                      }
                      frame True {
                      }
                    }
                    n1213 = local write "Save1 Array"(w2299) -> ()
                  }
                  frame #9 {
                    n1214 = Search 1D Array(1D array=w2318, element="VT-Lin (V):") -> (index of element=w2320:i32)  [unwired: 1 in]
                    n1215 = Equal?(x=w2320, y=-1) -> (x = y?=w2319:bool)
                    n1216 = local read "Save1 Array"() -> (w2317:string[][])
                    n1217 = case shown="True" w2319 {
                      tunnel: w2317 -> [w2328 w2332]
                      tunnel: w2320 -> [w2324 _]
                      tunnel: [w2323 w2332] -> w2316
                      frame False {
                        n1218 = local read "New: VT-Lin"() -> (w2330:dbl)
                        n1219 = Number To Fractional String(number=w2330) -> (F-format string=w2325:string)  [unwired: 3 in]
                        n1220 = Divide(x=w2324, y=3) -> (x/y=w2327:dbl)
                        n1221 = To Word Integer(number=w2327) -> (16bit integer=w2326:i16)
                        n1222 = Replace Array Subset(array=w2328, new element=w2325, index (row)=w2326, index (col)=1) -> (w2323:string[][])
                      }
                      frame True {
                      }
                    }
                    n1223 = local write "Save1 Array"(w2316) -> ()
                  }
                  frame #10 {
                    n1224 = Search 1D Array(1D array=w2335, element="STS-Sat (V/decade):") -> (index of element=w2337:i32)  [unwired: 1 in]
                    n1225 = Equal?(x=w2337, y=-1) -> (x = y?=w2336:bool)
                    n1226 = local read "Save1 Array"() -> (w2334:string[][])
                    n1227 = case shown="False" w2336 {
                      tunnel: w2334 -> [w2345 w2349]
                      tunnel: w2337 -> [w2341 _]
                      tunnel: [w2340 w2349] -> w2333
                      frame False {
                        n1228 = local read "New: STS"() -> (w2347:dbl)
                        n1229 = Number To Fractional String(number=w2347) -> (F-format string=w2342:string)  [unwired: 3 in]
                        n1230 = Divide(x=w2341, y=3) -> (x/y=w2344:dbl)
                        n1231 = To Word Integer(number=w2344) -> (16bit integer=w2343:i16)
                        n1232 = Replace Array Subset(array=w2345, new element=w2342, index (row)=w2343, index (col)=1) -> (w2340:string[][])
                      }
                      frame True {
                      }
                    }
                    n1233 = local write "Save1 Array"(w2333) -> ()
                  }
                  frame #11 {
                    n1234 = Search 1D Array(1D array=w2352, element="Trap Density-VT (Traps/Vcm^2):") -> (index of element=w2354:i32)  [unwired: 1 in]
                    n1235 = Equal?(x=w2354, y=-1) -> (x = y?=w2353:bool)
                    n1236 = local read "Save1 Array"() -> (w2351:string[][])
                    n1237 = case shown="False" w2353 {
                      tunnel: w2351 -> [w2362 w2366]
                      tunnel: w2354 -> [w2358 _]
                      tunnel: [w2357 w2366] -> w2350
                      frame False {
                        n1238 = local read "New: Trap Density-VT"() -> (w2364:dbl)
                        n1239 = Number To Fractional String(number=w2364) -> (F-format string=w2359:string)  [unwired: 3 in]
                        n1240 = Divide(x=w2358, y=3) -> (x/y=w2361:dbl)
                        n1241 = To Word Integer(number=w2361) -> (16bit integer=w2360:i16)
                        n1242 = Replace Array Subset(array=w2362, new element=w2359, index (row)=w2360, index (col)=1) -> (w2357:string[][])
                      }
                      frame True {
                      }
                    }
                    n1243 = local write "Save1 Array"(w2350) -> ()
                  }
                  frame #12 {
                    n1244 = Search 1D Array(1D array=w2369, element="Trap Density-STS (Traps/Vcm^2):") -> (index of element=w2371:i32)  [unwired: 1 in]
                    n1245 = Equal?(x=w2371, y=-1) -> (x = y?=w2370:bool)
                    n1246 = local read "Save1 Array"() -> (w2368:string[][])
                    n1247 = case shown="False" w2370 {
                      tunnel: w2368 -> [w2379 w2383]
                      tunnel: w2371 -> [w2375 _]
                      tunnel: [w2374 w2383] -> w2367
                      frame False {
                        n1248 = local read "New: Trap Density-STS"() -> (w2381:dbl)
                        n1249 = Number To Fractional String(number=w2381) -> (F-format string=w2376:string)  [unwired: 3 in]
                        n1250 = Divide(x=w2375, y=3) -> (x/y=w2378:dbl)
                        n1251 = To Word Integer(number=w2378) -> (16bit integer=w2377:i16)
                        n1252 = Replace Array Subset(array=w2379, new element=w2376, index (row)=w2377, index (col)=1) -> (w2374:string[][])
                      }
                      frame True {
                      }
                    }
                    n1253 = local write "Save1 Array"(w2367) -> ()
                  }
                }
                n1254 = Concatenate Strings(w2159, "\\", w2157) -> (w2158:string)
                n1255 = String To Path(string=w2158) -> (path=w2135:path)
                "No Image 2" <- w2135
                n1256 = local write "Save1 Array"(w2132) -> ()
              }
              frame #1 {
                n1257 = Equal?(x=w2387, y=w2386) -> (x = y?=w2385:bool)
                n1258 = case shown="False" w2385 {
                  tunnel: w2387 -> [w2391 _]
                  tunnel: w2386 -> [w2390 _]
                  frame False {
                    n1259 = Move(source path=w2391, 9:TRUE, 10:w2390) -> ()  [unwired: 2 in, 3 out]
                  }
                  frame True {
                  }
                }
              }
              frame #2 {
                n1260 = local write "Transfer File"(w2393) -> ()
                n1261 = call-poly <vilib>:"Write To Spreadsheet File.vi"("2D data"=w2392, "file path (dialog if empty)"=w2393) -> ()  [unwired: 6 in, 1 out]
              }
              frame #3 {
                w2493 = 0
                # "Moves to next file and displays new image/data"
                n1262 = property on="Image Out" class="ImageControl"() -> (error out=w2455:errorcluster, "Image Center Position"=w2459:cluster{"X":u32, "Y":u32})  [unwired: 2 in, 1 out]
                n1263 = local read "Transfer File"() -> (w2498:path)
                n1264 = Strip Path(path=w2498) -> (stripped path=w2489:path, name=w2507:string)
                n1265 = Unbundle(w2459) -> ("X"=w2457:u32)  [unwired: 1 out]
                n1266 = local write "Transfer Folder"(w2489) -> ()
                n1267 = Bundle("X"=w2457, 0) -> (w2458:cluster{"X":u32, i32})  [unwired: 1 in]
                n1268 = property on="Image Out" class="ImageControl"(error in=w2455, "Image Center Position"=w2458) -> ()  [unwired: 1 in, 2 out]
                n1269 = List Folder(path=w2489) -> (filenames=w2503:string[])  [unwired: 3 in, 3 out]
                n1270 = Search 1D Array(1D array=w2503, element=w2507) -> (index of element=w2500:i32)  [unwired: 1 in]
                n1271 = Array Size(array=w2503) -> (size(s)=w2499:i32)
                n1272 = Decrement(x=w2499) -> (x-1=w2501:i32)
                n1273 = Equal?(x=w2500, y=w2501) -> (x = y?=w2502:bool)
                n1274 = local read "Folder Index"() -> (w2451:dbl)
                n1275 = case shown="False" w2502 {
                  tunnel: w2451 -> [w2632 _]
                  tunnel: [w2631 0] -> w2450
                  frame False {
                    n1276 = Increment(x=w2632) -> (x+1=w2631:dbl)
                  }
                  frame True {
                  }
                }
                n1277 = invoke on="Image Out" class="ImageControl" method="Clear ROI"() -> ()  [unwired: 3 in, 3 out]
                n1278 = local write "Folder Index"(w2450) -> ()
                n1279 = Path To String(path=w2489) -> (string=w2508:string)
                n1280 = Index Array(array=w2503, index=w2450) -> (element=w2504:string)
                n1281 = local write "Data Name:"(w2504) -> ()
                n1282 = Concatenate Strings(w2508, "\\", w2504) -> (w2506:string)
                n1283 = String To Path(string=w2506) -> (path=w2402:path)
                n1284 = call "Recorded Values.vi"("Path"=w2402) -> ("Recorded Char"=w2404:T5, "Recorded Prop"=w2405:T6, "Fabrication Prop"=w2403:T7)  [unwired: 8 in]
                n1285 = Unbundle By Name(w2404) -> ("Mobility-Sat"=w2417:dbl, "Moblitity-Lin"=w2418:dbl, "On/Off"=w2419:dbl, "Off Current"=w2420:dbl, "Vt-Sat"=w2396:dbl, "STS"=w2421:dbl, "Trap Density-VT"=w2422:dbl, "Trap Density-STS"=w2423:dbl)
                n1286 = Unbundle By Name(w2405) -> ("Date Recorded"=w2413:string, "Index"=w2414:string, "Length"=w2415:dbl, "Width"=w2416:dbl, "Sample Temp"=w2399:dbl)
                n1287 = Unbundle By Name(w2403) -> ("Date Created"=w2424:string, "Material"=w2406:string, "Solvent"=w2407:string, "Concentration"=w2408:dbl, "Method"=w2409:string, "Dielectric (nm)"=w2410:dbl, "Treatment"=w2411:string, "Comments"=w2412:string)
                n1288 = local write "Rec: Off I-Sat"(w2420) -> ()
                n1289 = local write "Rec: VT-Sat"(w2396) -> ()
                n1290 = local write "Date Created"(w2424) -> ()
                n1291 = local write "Rec: Material"(w2406) -> ()
                n1292 = local write "Rec: Solvent"(w2407) -> ()
                n1293 = local write "Rec: Concentration"(w2408) -> ()
                n1294 = local write "Rec: Method"(w2409) -> ()
                n1295 = local write "Rec: Dielectric (d)"(w2410) -> ()
                n1296 = local write "Surface Treatment:"(w2411) -> ()
                n1297 = local write "Comments"(w2412) -> ()
                n1298 = local write "Index"(w2414) -> ()
                n1299 = local write "Rec: Mobility-Sat"(w2417) -> ()
                n1300 = local write "Rec: Mobility-Lin"(w2418) -> ()
                n1301 = local write "Rec: On/Off"(w2419) -> ()
                n1302 = local write "Rec: STS"(w2421) -> ()
                n1303 = local write "Rec: Trap Density-VT"(w2422) -> ()
                n1304 = local write "Rec: Trap Density-STS"(w2423) -> ()
                n1305 = local write "Date Recorded"(w2413) -> ()
                n1306 = local write "Rec: Length"(w2415) -> ()
                n1307 = local write "Rec: Width"(w2416) -> ()
                n1308 = local write "Rec: Temp"(w2399) -> ()
                n1309 = Equal To 0?(x=w2399) -> (x = 0?=w2400:bool)
                n1310 = case shown="False" w2400 {
                  tunnel: [w2509 w2510] -> w2397
                  tunnel: w2399 -> [w2509 _]
                  frame False {
                  }
                  frame True {
                    n1311 = local read "Room Temp"() -> (w2510:dbl)
                  }
                }
                n1312 = local write "Transfer File"(w2402) -> ()
                n1313 = local read "NumPts 2"() -> (w2446:dbl)
                n1314 = local read "NumPts"() -> (w2435:dbl)
                n1315 = local read "NumPts"() -> (w2447:dbl)
                n1316 = call-poly <vilib>:"Read From Spreadsheet File.vi"("file path (dialog if empty)"=w2402) -> ("all rows"=w2495:string[][])  [unwired: 6 in, 4 out]
                n1317 = call "Mobility-Vt Calculator-File.vi"("NumPts"=w2447, "Path"=w2402) -> ("XY Graph-Sat"=w2448:cluster{dbl[], dbl[]}[], "XY Graph-Lin"=w2430:cluster{dbl[], dbl[]}[], "Output"=w2449:T8, "Index-Sat"=w2427:dbl, "Index-Lin"=w2434:dbl)  [unwired: 4 in, 1 out]
                n1318 = Decimate 1D Array(w2430) -> (w2442:cluster{dbl[], dbl[]}[])  [unwired: 1 out]
                n1319 = Array To Cluster(array=w2442) -> (cluster=w2440:T9)
                n1320 = Unbundle(w2440) -> ("[0]"=w2441:cluster{dbl[], dbl[]})  [unwired: 8 out]
                n1321 = local write "XY Graph-Lin"(w2430) -> ()
                n1322 = Unbundle(w2441) -> (w2439:dbl[], w2438:dbl[])
                n1323 = Array Subset(array=w2438, index=w2434, length=w2435) -> (w2436:dbl[])
                n1324 = Array Subset(array=w2439, index=w2434, length=w2435) -> (w2437:dbl[])
                n1325 = call "STS Calculator-File.vi"("NumPts"=w2446, "Path"=w2402) -> ("STS Index-Sat"=w2445:dbl, "XY Graph-Sat"=w2444:cluster{dbl[], dbl[]}[], "Ouput"=w2443:cluster{"STS-Sat":dbl, "STS-Lin":dbl})  [unwired: 5 in, 2 out]
                n1326 = local read "New: Dielectric"() -> (w2429:dbl)
                n1327 = local write "Lin Id-Used"(w2436) -> ()
                n1328 = local write "Lin-Vg Array-Used"(w2437) -> ()
                n1329 = local write "MobVi Index"(w2427) -> ()
                n1330 = local write "Slide"(w2427) -> ()
                n1331 = local write "XY Graph"(w2448) -> ()
                n1332 = local write "Index 2"(w2445) -> ()
                n1333 = local write "XY Graph 2"(w2444) -> ()
                n1334 = Unbundle By Name(w2449) -> ("Mobility-Sat"=w2433:dbl, "Vt-Sat"=w2394:dbl, "Mobility-Lin"=w2432:dbl, "Mobility-Lin"=w2431:dbl, "Off I-Sat"=w2425:dbl, "On/Off I-Sat"=w2395:dbl)
                n1335 = Array Size(array=w2495) -> (size(s)=w2494:i32[])
                n1336 = local write "New: Temp"(w2397) -> ()
                n1337 = Unbundle By Name(w2443) -> ("STS-Sat"=w2428:dbl)
                n1338 = call "Trap Density_STS.vi"("Temp (T) [K]"=w2397, "S.T.S. (S)"=w2428, "Dielectric"=w2429) -> ("Trap Density (N)"=w2401:dbl)  [unwired: 8 in]
                n1339 = local write "Calc: Mobility-Lin"(w2432) -> ()
                n1340 = local write "Calc: Mobility-Sat"(w2433) -> ()
                n1341 = local write "Calc: Off I-Sat"(w2425) -> ()
                n1342 = local write "Calc: VT-Sat"(w2394) -> ()
                n1343 = local write "New: VT-Lin"(w2431) -> ()
                n1344 = local write "New: Trap Density-STS"(w2401) -> ()
                n1345 = local write "Calc: Trap Density-STS"(w2401) -> ()
                n1346 = local read "Image Folder"() -> (w2483:path)
                n1347 = local read "New: Dielectric"() -> (w2426:dbl)
                n1348 = Decimate 1D Array(w2448) -> (w2478:cluster{dbl[], dbl[]}[])  [unwired: 1 out]
                n1349 = Decimate 1D Array(w2444) -> (w2468:cluster{dbl[], dbl[]}[])  [unwired: 1 out]
                n1350 = Index Array(array=w2494, index=w2493) -> (element=w2474:i32)
                n1351 = Array Subset(array=w2495, index (row)=w2493, index (col)=w2493, length (col)=3) -> (w2496:string[][])  [unwired: 1 in]
                n1352 = local write "Calc: STS"(w2428) -> ()
                n1353 = local write "New: VT-Sat"(w2394) -> ()
                n1354 = local write "New: Mobility-Sat"(w2433) -> ()
                n1355 = local write "Calc: On/Off"(w2395) -> ()
                n1356 = local write "New: Mobility-Lin"(w2432) -> ()
                n1357 = List Folder(path=w2483) -> (filenames=w2488:string[])  [unwired: 3 in, 3 out]
                n1358 = local write "New: VT-Lin"(w2431) -> ()
                n1359 = Array To Cluster(array=w2478) -> (cluster=w2480:T9)
                n1360 = Array To Cluster(array=w2468) -> (cluster=w2466:T9)
                n1361 = Reshape Array(w2496, w2474) -> (w2481:string[])
                n1362 = Subtract(x=w2474, y=20) -> (x-y=w2473:i32)
                n1363 = local write "New: STS"(w2428) -> ()
                n1364 = property on="Slide" class="Slide (strict)"("Scale.Maximum"=w2473) -> ()  [unwired: 2 in, 2 out]
                n1365 = call "Trap Density_VT.vi"("VT"=w2394, "Dielectric"=w2426) -> ("Trap Density-VT"=w2398:dbl)
                n1366 = Unbundle(w2480) -> ("[0]"=w2479:cluster{dbl[], dbl[]})  [unwired: 8 out]
                n1367 = Unbundle(w2466) -> ("[0]"=w2467:cluster{dbl[], dbl[]})  [unwired: 8 out]
                n1368 = Search 1D Array(1D array=w2481, element="Index:") -> (index of element=w2490:i32)  [unwired: 1 in]
                n1369 = local write "New: Trap Density-VT"(w2398) -> ()
                n1370 = local write "Calc: Trap Density-VT"(w2398) -> ()
                n1371 = Unbundle(w2479) -> (w2470:dbl[], w2469:dbl[])
                n1372 = Unbundle(w2467) -> (w2465:dbl[], w2464:dbl[])
                n1373 = Increment(x=w2490) -> (x+1=w2491:i32)
                n1374 = Array Subset(array=w2470, index=w2427, length=w2447) -> (w2477:dbl[])
                n1375 = Array Subset(array=w2469, index=w2427, length=w2447) -> (w2476:dbl[])
                n1376 = Array Subset(array=w2465, index=w2445, length=w2446) -> (w2472:dbl[])
                n1377 = Array Subset(array=w2464, index=w2445, length=w2446) -> (w2471:dbl[])
                n1378 = Index Array(array=w2481, index=w2491) -> (element=w2486:string)
                n1379 = local write "Vg Array-Log-Used"(w2471) -> ()
                n1380 = local write "Sat Id-Log-Used"(w2472) -> ()
                n1381 = local write "Sat Id-Used"(w2476) -> ()
                n1382 = local write "Index"(w2486) -> ()
                n1383 = local write "Sat Vg Array-Used"(w2477) -> ()
                n1384 = while {
                  tunnel: w2488 -> [w2518]
                  tunnel: w2486 -> [w2516]
                  tunnel: [w2515] -> _
                  tunnel: [w2515] -> w2487
                  tunnel: w2474 -> [w2514]
                  i -> [w2515]
                  stop <- w2511 stop-if-true
                  n1385 = Index Array(array=w2518, index=w2515) -> (element=w2519:string)
                  n1386 = xnode "Match Regular Expression"("input string"=w2519, "regular expression"=w2516) -> ("whole match"=w2517:string)  [unwired: 4 in, 4 out]
                  n1387 = Equal?(x=w2517, y=w2516) -> (x = y?=w2513:bool)
                  n1388 = Equal?(x=w2514, y=w2515) -> (x = y?=w2512:bool)
                  n1389 = Or(x=w2513, y=w2512) -> (x .or. y?=w2511:bool)
                }
                n1390 = Path To String(path=w2483) -> (string=w2485:string)
                n1391 = Index Array(array=w2488, index=w2487) -> (element=w2462:string)
                n1392 = local write "Image Name"(w2462) -> ()
                n1393 = Empty String/Path?(string/path=w2462) -> (empty?=w2463:bool)
                n1394 = Concatenate Strings(w2485, "\\", w2462) -> (w2484:string)
                n1395 = String To Path(string=w2484) -> (path=w2461:path)
                n1396 = local read "No Image File"() -> (w2460:path)
                n1397 = Select(t=w2460, s=w2463, f=w2461) -> (s? t:f=w2454:path)
                n1398 = local write "Image File"(w2454) -> ()
                n1399 = local read "Image Out"() -> (w2452:T2)
                n1400 = call "IMAQ ReadFile"("File Path"=w2454, "Image"=w2452) -> ("Image Out"=w2453:T2)  [unwired: 5 in, 4 out]
                n1401 = local write "Image Out"(w2453) -> ()
                n1402 = local write "Image Out 2"(w2453) -> ()
              }
              frame #4 {
                # "Output ROI data"
                n1403 = local read "Image Folder"() -> (w2634:path)
                n1404 = Build Path(base path=w2634, name or relative path="ROI") -> (appended path=w2636:path)
                n1405 = local read "Index"() -> (w2635:string)
                n1406 = Build Path(base path=w2636, name or relative path=w2635) -> (appended path=w2641:path)
                n1407 = invoke on="Image Out" class="ImageControl" method="Clear ROI"() -> (error out=w2640:errorcluster)  [unwired: 3 in, 2 out]
                n1408 = call <vilib>:"Check if File or Folder Exists.vi"("error in (no error)"=w2640, "path"=w2641) -> ("file or folder exists?"=w2638:bool, "dup path"=w2639:path)  [unwired: 7 in, 1 out]
                n1409 = case shown="True" w2638 {
                  tunnel: w2639 -> [_ w2642]
                  frame False {
                  }
                  frame True {
                    n1410 = Read from Text File(file (use dialog)=w2642) -> (text=w2646:string)  [unwired: 3 in, 3 out]
                    n1411 = property on="Image Out" class="ImageControl"() -> ("ROI"=w2643:T10)  [unwired: 2 in, 2 out]
                    n1412 = Unflatten From String(type=w2643, binary string=w2646) -> (value=w2644:T10, error out=w2645:errorcluster)  [unwired: 3 in, 1 out]
                    n1413 = property on="Image Out" class="ImageControl"(error in=w2645, "ROI"=w2644) -> ()  [unwired: 1 in, 2 out]
                  }
                }
              }
            }
            n1414 = flat-sequence {
              tunnel: [w2089] -> w2076
              tunnel: w2076 -> [w2103]
              frame #0 {
                # "Makes Empty File for Transformer Data"
                n1415 = local read "Transfer Folder"() -> (w2078:path)
                n1416 = Build Path(base path=w2078, name or relative path="Stats") -> (appended path=w2080:path)
                n1417 = call <vilib>:"Check if File or Folder Exists.vi"("path"=w2080) -> ("file or folder exists?"=w2081:bool, "dup path"=w2082:path)  [unwired: 8 in, 1 out]
                n1418 = case shown="False" w2081 {
                  tunnel: [w2086 w2088] -> w2083
                  tunnel: w2082 -> [w2087 w2088]
                  frame False {
                    n1419 = Create Folder(path (use dialog)=w2087) -> (created path=w2086:path)  [unwired: 2 in, 2 out]
                  }
                  frame True {
                  }
                }
                n1420 = Build Path(base path=w2083, name or relative path="Tranformer Data.txt") -> (appended path=w2085:path)
                n1421 = call-poly <vilib>:"Write To Spreadsheet File.vi"("append to file? (new file:F)"=TRUE, "file path (dialog if empty)"=w2085) -> ()  [unwired: 6 in, 1 out]
              }
              frame #1 {
                # "Adds Headers if they don't exist"
                n1422 = local read "Transfer Folder"() -> (w2095:path)
                n1423 = Concatenate Strings("Stats\\", "Tranformer Data.txt") -> (w2096:string)
                n1424 = Build Path(base path=w2095, name or relative path=w2096) -> (appended path=w2089:path)
                n1425 = call-poly <vilib>:"Read From Spreadsheet File.vi"("file path (dialog if empty)"=w2089) -> ("first row"=w2094:string[])  [unwired: 6 in, 4 out]
                n1426 = Search 1D Array(1D array=w2094, element="DeviceID") -> (index of element=w2092:i32)  [unwired: 1 in]
                n1427 = Equal?(x=w2092, y=0) -> (x = y?=w2090:bool)
                n1428 = case shown="False" w2090 {
                  tunnel: w2089 -> [w2100 _]
                  frame False {
                    n1429 = local read "Transformer \nHeaders"() -> (w2099:string[])
                    n1430 = call-poly <vilib>:"Write To Spreadsheet File.vi"("1D data"=w2099, "file path (dialog if empty)"=w2100) -> ()  [unwired: 6 in, 1 out]
                  }
                  frame True {
                  }
                }
              }
              frame #2 {
                # "Adds current device if it doesn't exist"
                n1431 = local read "Current \nRecord"() -> (w2106:string[])
                n1432 = Index Array(array=w2106, index=0) -> (element=w2105:string)
                n1433 = local read "Transfer Folder"() -> (w2108:path)
                n1434 = Concatenate Strings("Stats\\", "Tranformer Data.txt") -> (w2109:string)
                n1435 = local write "Current Device ID"(w2105) -> ()
                n1436 = local read "Current Device ID"() -> (w2115:string)
                n1437 = Build Path(base path=w2108, name or relative path=w2109) -> (appended path=w2107:path)
                n1438 = call-poly <vilib>:"Read From Spreadsheet File.vi"("file path (dialog if empty)"=w2107) -> ("all rows"=w2102:string[][])  [unwired: 6 in, 4 out]
                n1439 = Index Array(array=w2102, index (col)=0) -> (element=w2113:string[])  [unwired: 1 in]
                n1440 = Search 1D Array(1D array=w2113, element=w2115) -> (index of element=w2101:i32)  [unwired: 1 in]
                n1441 = Equal?(x=w2101, y=-1) -> (x = y?=w2104:bool)
                n1442 = case shown="False" w2104 {
                  tunnel: w2103 -> [w2117 w2130]
                  tunnel: w2101 -> [w2122 _]
                  tunnel: w2102 -> [w2123 _]
                  frame False {
                    n1443 = local read "Current \nRecord"() -> (w2121:string[])
                    n1444 = Replace Array Subset(array=w2123, new element=w2121, index (row)=w2122) -> (w2118:string[][])  [unwired: 1 in]
                    n1445 = flat-sequence {
                      tunnel: [w2124] -> _
                      tunnel: [w2125] -> _
                      tunnel: [w2125] -> w2120
                      tunnel: [w2124] -> w2119
                      tunnel: w2118 -> [w2125]
                      tunnel: w2117 -> [w2124]
                      tunnel: w2120 -> [w2127]
                      tunnel: w2119 -> [w2126]
                      frame #0 {
                        n1446 = Delete(path (use dialog)=w2124) -> ()  [unwired: 4 in, 3 out]
                      }
                      frame #1 {
                        n1447 = call-poly <vilib>:"Write To Spreadsheet File.vi"("append to file? (new file:F)"=TRUE, "2D data"=w2127, "file path (dialog if empty)"=w2126) -> ()  [unwired: 5 in, 1 out]
                      }
                    }
                  }
                  frame True {
                    n1448 = local read "Current \nRecord"() -> (w2129:string[])
                    n1449 = call-poly <vilib>:"Write To Spreadsheet File.vi"("append to file? (new file:F)"=TRUE, "1D data"=w2129, "file path (dialog if empty)"=w2130) -> ()  [unwired: 5 in, 1 out]
                  }
                }
              }
            }
          }
          event "Export": Mouse Down {
            n1450 = event-data() -> ()  [unwired: 1 in, 7 out]
            n1451 = flat-sequence {
              frame #0 {
                n1452 = stacked-sequence {
                  frame #0 {
                    n1453 = local read "Independant Variable"() -> (w2648:string)
                    n1454 = Equal?(x=w2648, y="Length (um):") -> (x = y?=w2649:bool)
                    n1455 = case shown="True" w2649 {
                      frame False {
                      }
                      frame True {
                        n1456 = local write "Opj X Axis"("2") -> ()
                      }
                    }
                  }
                  frame #1 {
                    n1457 = local read "Independant Variable"() -> (w2652:string)
                    n1458 = Equal?(x=w2652, y="Sample Temp (K):") -> (x = y?=w2653:bool)
                    n1459 = case shown="True" w2653 {
                      frame False {
                      }
                      frame True {
                        n1460 = local write "Opj X Axis"("1") -> ()
                      }
                    }
                  }
                  frame #2 {
                    n1461 = local read "Independant Variable"() -> (w2656:string)
                    n1462 = Equal?(x=w2656, y="Mobility-Sat (cm^2/Vs):") -> (x = y?=w2657:bool)
                    n1463 = case shown="True" w2657 {
                      frame False {
                      }
                      frame True {
                        n1464 = local write "Opj X Axis"("2") -> ()
                      }
                    }
                  }
                  frame #3 {
                    n1465 = local read "Independant Variable"() -> (w2660:string)
                    n1466 = Equal?(x=w2660, y="Mobility-Lin (cm^2/Vs):") -> (x = y?=w2661:bool)
                    n1467 = case shown="True" w2661 {
                      frame False {
                      }
                      frame True {
                        n1468 = local write "Opj X Axis"("2") -> ()
                      }
                    }
                  }
                  frame #4 {
                    n1469 = local read "Independant Variable"() -> (w2664:string)
                    n1470 = Equal?(x=w2664, y="On/Off I-Sat:") -> (x = y?=w2665:bool)
                    n1471 = case shown="True" w2665 {
                      frame False {
                      }
                      frame True {
                        n1472 = local write "Opj X Axis"("2") -> ()
                      }
                    }
                  }
                  frame #5 {
                    n1473 = local read "Independant Variable"() -> (w2668:string)
                    n1474 = Equal?(x=w2668, y="Off I-Sat (A):") -> (x = y?=w2669:bool)
                    n1475 = case shown="True" w2669 {
                      frame False {
                      }
                      frame True {
                        n1476 = local write "Opj X Axis"("2") -> ()
                      }
                    }
                  }
                  frame #6 {
                    n1477 = local read "Independant Variable"() -> (w2672:string)
                    n1478 = Equal?(x=w2672, y="Vt-Sat (V):") -> (x = y?=w2673:bool)
                    n1479 = case shown="True" w2673 {
                      frame False {
                      }
                      frame True {
                        n1480 = local write "Opj X Axis"("1") -> ()
                      }
                    }
                  }
                  frame #7 {
                    n1481 = local read "Independant Variable"() -> (w2676:string)
                    n1482 = Equal?(x=w2676, y="STS-Sat (V/decade):") -> (x = y?=w2677:bool)
                    n1483 = case shown="True" w2677 {
                      frame False {
                      }
                      frame True {
                        n1484 = local write "Opj X Axis"("1") -> ()
                      }
                    }
                  }
                  frame #8 {
                    n1485 = local read "Independant Variable"() -> (w2680:string)
                    n1486 = Equal?(x=w2680, y="Trap Density-VT (Traps/Vcm^2):") -> (x = y?=w2681:bool)
                    n1487 = case shown="True" w2681 {
                      frame False {
                      }
                      frame True {
                        n1488 = local write "Opj X Axis"("2") -> ()
                      }
                    }
                  }
                  frame #9 {
                    n1489 = local read "Independant Variable"() -> (w2684:string)
                    n1490 = Equal?(x=w2684, y="Trap Density-STS (Traps/Vcm^2):") -> (x = y?=w2685:bool)
                    n1491 = case shown="True" w2685 {
                      frame False {
                      }
                      frame True {
                        n1492 = local write "Opj X Axis"("2") -> ()
                      }
                    }
                  }
                }
              }
              frame #1 {
                n1493 = local read "Transfer Folder"() -> (w2692:path)
                n1494 = Build Path(base path=w2692, name or relative path="Stats") -> (appended path=w2693:path)
                n1495 = local read "Origin Project File"() -> (w2704:path)
                n1496 = call <vilib>:"Check if File or Folder Exists.vi"("path"=w2693) -> ("file or folder exists?"=w2708:bool, "dup path"=w2707:path)  [unwired: 8 in, 1 out]
                n1497 = call <userlib>:"OA_ConnectToOrigin.vi"() -> ("error out"=w2705:errorcluster, "Origin.IOApplication"=w2706:refnum<k7>)  [unwired: 8 in]
                n1498 = case shown="False" w2708 {
                  tunnel: w2707 -> [w2865 w2866]
                  tunnel: [w2864 w2866] -> w2691
                  frame False {
                    n1499 = Create Folder(path (use dialog)=w2865) -> (created path=w2864:path)  [unwired: 2 in, 2 out]
                  }
                  frame True {
                  }
                }
                n1500 = call <userlib>:"OA_Load.vi"("error in (no error)"=w2705, "Path"=w2704, "Origin.IOApplication"=w2706) -> ("error out"=w2702:errorcluster, "Origin.IOApplication"=w2703:refnum<k7>)  [unwired: 1 out]
                n1501 = call <userlib>:"OAExecute.vi"("script"="document -m 3;", "Error IO"=w2702, "Origin.IOApplication"=w2703) -> ("Error IO Out"=w2700:errorcluster, "Origin.IOApplication"=w2701:refnum<k7>)  [unwired: 1 in, 1 out]
                n1502 = call "File Dialog"("start path"=w2693) -> ("selected path"=w2695:path)  [unwired: 11 in, 3 out]
                n1503 = local read "Independant Variable"() -> (w2688:string)
                n1504 = stacked-sequence {
                  tunnel: w2692 -> [w2717 w2745 w2755 w2775 w2793 w2812 w2831 w2852]
                  tunnel: w2691 -> [w2718 w2744 w2756 w2774 w2794 w2813 w2832 w2853]
                  tunnel: w2701 -> [w2720 w2742 w2758 w2777 w2796 w2815 w2834 w2855]
                  tunnel: w2700 -> [w2719 w2743 w2757 w2776 w2795 w2814 w2833 w2854]
                  tunnel: [_ _ _ _ _ _ _ w2850] -> w2690
                  tunnel: [_ _ _ _ _ _ _ w2851] -> w2689
                  tunnel: w2688 -> [w2716 w2735 w2754 w2773 w2792 w2811 w2830 w2849]
                  frame #0 {
                    n1505 = local read "Opj X Axis"() -> (w2712:string)
                    n1506 = Concatenate Strings("window -a MOBLGraph;\nlayer.x.type=", w2712, ";", "window -a MOBLTable;\nwindow -s TV;") -> (w2710:string)
                    n1507 = call "Param_Analysis_7_24b_JW.vi"("Independant Variable"=w2716, "error in (no error)"=w2719, "Data Folder"=w2717, "Parameter String"="Mobility-Lin (cm^2/Vs):", "Parameter Name"="Mobility-Lin", "Stats Folder"=w2718) -> ("error out"=w2722:errorcluster, "Output Array"=w2724:string[][], "Variables"=w2715:T16)  [unwired: 2 in, 1 out]
                    n1508 = call "Origin_Export_7_27a_JW.vi"("Input Conditions"=w2715, "Analysis Array"=w2724, "error in (no error)"=w2722, "Parameter Worksheet Name"="[MOBLTable]Mobilities", "Parameter Folder Script"="pe_cd \"Mobility-Lin\";", "Origin.IOApplication"=w2720) -> ("error out"=w2721:errorcluster, "reference out"=w2723:refnum<k7>)  [unwired: 3 in, 1 out]
                    n1509 = call <userlib>:"OAExecute.vi"("script"=w2710, "Error IO"=w2721, "Origin.IOApplication"=w2723) -> ()  [unwired: 1 in, 3 out]
                  }
                  frame #1 {
                    n1510 = local read "Opj X Axis"() -> (w2731:string)
                    n1511 = Concatenate Strings("window -a MOBSGraph;\nlayer.x.type=", w2731, ";", "window -a MOBSTable;\nwindow -s TV;") -> (w2729:string)
                    n1512 = call "Param_Analysis_7_24b_JW.vi"("Independant Variable"=w2735, "error in (no error)"=w2743, "Data Folder"=w2745, "Parameter String"="Mobility-Sat (cm^2/Vs):", "Parameter Name"="Mobility-Sat", "Stats Folder"=w2744) -> ("error out"=w2738:errorcluster, "Output Array"=w2736:string[][], "Variables"=w2734:T16)  [unwired: 2 in, 1 out]
                    n1513 = call "Origin_Export_7_27a_JW.vi"("Input Conditions"=w2734, "Analysis Array"=w2736, "error in (no error)"=w2738, "Parameter Worksheet Name"="[MOBSTable]Mobilities", "Parameter Folder Script"="pe_cd \"Mobility-Sat\";", "Origin.IOApplication"=w2742) -> ("error out"=w2737:errorcluster, "reference out"=w2739:refnum<k7>)  [unwired: 3 in, 1 out]
                    n1514 = call <userlib>:"OAExecute.vi"("script"=w2729, "Error IO"=w2737, "Origin.IOApplication"=w2739) -> ()  [unwired: 1 in, 3 out]
                  }
                  frame #2 {
                    n1515 = local read "Opj X Axis"() -> (w2750:string)
                    n1516 = Concatenate Strings("window -a NSTSGraph;\nlayer.x.type=", w2750, ";", "window -a NSTSTable;\nwindow -s TV;") -> (w2748:string)
                    n1517 = call "Param_Analysis_7_24b_JW.vi"("Independant Variable"=w2754, "error in (no error)"=w2757, "Data Folder"=w2755, "Parameter String"="Trap Density-STS (Traps/Vcm^2):", "Parameter Name"="Trap Density-STS", "Stats Folder"=w2756) -> ("error out"=w2761:errorcluster, "Output Array"=w2759:string[][], "Variables"=w2753:T16)  [unwired: 2 in, 1 out]
                    n1518 = call "Origin_Export_7_27a_JW.vi"("Input Conditions"=w2753, "Analysis Array"=w2759, "error in (no error)"=w2761, "Parameter Worksheet Name"="[NSTSTable]Trap Densities", "Parameter Folder Script"="pe_cd \"N-STS\";", "Origin.IOApplication"=w2758) -> ("error out"=w2760:errorcluster, "reference out"=w2762:refnum<k7>)  [unwired: 3 in, 1 out]
                    n1519 = call <userlib>:"OAExecute.vi"("script"=w2748, "Error IO"=w2760, "Origin.IOApplication"=w2762) -> ()  [unwired: 1 in, 3 out]
                  }
                  frame #3 {
                    n1520 = local read "Opj X Axis"() -> (w2769:string)
                    n1521 = call "Param_Analysis_7_24b_JW.vi"("Independant Variable"=w2773, "error in (no error)"=w2776, "Data Folder"=w2775, "Parameter String"="Trap Density-VT (Traps/Vcm^2):", "Parameter Name"="Trap Density-Vt", "Stats Folder"=w2774) -> ("error out"=w2780:errorcluster, "Output Array"=w2778:string[][], "Variables"=w2772:T16)  [unwired: 2 in, 1 out]
                    n1522 = Concatenate Strings("window -a NVtGraph;\nlayer.x.type=", w2769, ";", "window -a NVtTable;\nwindow -s TV;") -> (w2767:string)
                    n1523 = call "Origin_Export_7_27a_JW.vi"("Input Conditions"=w2772, "Analysis Array"=w2778, "error in (no error)"=w2780, "Parameter Worksheet Name"="[NVTTable]Trap Densities", "Parameter Folder Script"="pe_cd \"N-Vt\";", "Origin.IOApplication"=w2777) -> ("error out"=w2779:errorcluster, "reference out"=w2781:refnum<k7>)  [unwired: 3 in, 1 out]
                    n1524 = call <userlib>:"OAExecute.vi"("script"=w2767, "Error IO"=w2779, "Origin.IOApplication"=w2781) -> ()  [unwired: 1 in, 3 out]
                  }
                  frame #4 {
                    n1525 = local read "Opj X Axis"() -> (w2788:string)
                    n1526 = Concatenate Strings("window -a OffIGraph;\nlayer.x.type=", w2788, ";", "window -a OffITable;\nwindow -s TV;") -> (w2786:string)
                    n1527 = call "Param_Analysis_7_24b_JW.vi"("Independant Variable"=w2792, "error in (no error)"=w2795, "Data Folder"=w2793, "Parameter String"="Off I-Sat (A):", "Parameter Name"="Off I-Sat", "Stats Folder"=w2794) -> ("error out"=w2799:errorcluster, "Output Array"=w2797:string[][], "Variables"=w2791:T16)  [unwired: 2 in, 1 out]
                    n1528 = call "Origin_Export_7_27a_JW.vi"("Input Conditions"=w2791, "Analysis Array"=w2797, "error in (no error)"=w2799, "Parameter Worksheet Name"="[OffItable]OffCurrents", "Parameter Folder Script"="pe_cd \"OffI-Sat\";", "Origin.IOApplication"=w2796) -> ("error out"=w2798:errorcluster, "reference out"=w2800:refnum<k7>)  [unwired: 3 in, 1 out]
                    n1529 = call <userlib>:"OAExecute.vi"("script"=w2786, "Error IO"=w2798, "Origin.IOApplication"=w2800) -> ()  [unwired: 1 in, 3 out]
                  }
                  frame #5 {
                    n1530 = local read "Opj X Axis"() -> (w2807:string)
                    n1531 = Concatenate Strings("window -a OnOffGraph;\nlayer.x.type=", w2807, ";", "window -a OnOffTable;\nwindow -s TV;") -> (w2805:string)
                    n1532 = call "Param_Analysis_7_24b_JW.vi"("Independant Variable"=w2811, "error in (no error)"=w2814, "Data Folder"=w2812, "Parameter String"="On/Off I-Sat:", "Parameter Name"="OnOff Ratio", "Stats Folder"=w2813) -> ("error out"=w2818:errorcluster, "Output Array"=w2816:string[][], "Variables"=w2810:T16)  [unwired: 2 in, 1 out]
                    n1533 = call "Origin_Export_7_27a_JW.vi"("Input Conditions"=w2810, "Analysis Array"=w2816, "error in (no error)"=w2818, "Parameter Worksheet Name"="[OnOffTable]On/Off Ratios", "Parameter Folder Script"="pe_cd \"OnOff-Ratio\";", "Origin.IOApplication"=w2815) -> ("error out"=w2817:errorcluster, "reference out"=w2819:refnum<k7>)  [unwired: 3 in, 1 out]
                    n1534 = call <userlib>:"OAExecute.vi"("script"=w2805, "Error IO"=w2817, "Origin.IOApplication"=w2819) -> ()  [unwired: 1 in, 3 out]
                  }
                  frame #6 {
                    n1535 = local read "Opj X Axis"() -> (w2826:string)
                    n1536 = call "Param_Analysis_7_24b_JW.vi"("Independant Variable"=w2830, "error in (no error)"=w2833, "Data Folder"=w2831, "Parameter String"="STS-Sat (V/decade):", "Parameter Name"="STS-Sat", "Stats Folder"=w2832) -> ("error out"=w2837:errorcluster, "Output Array"=w2835:string[][], "Variables"=w2829:T16)  [unwired: 2 in, 1 out]
                    n1537 = Concatenate Strings("window -a SGraph;\nlayer.x.type=", w2826, ";", "window -a STable;\nwindow -s TV;") -> (w2824:string)
                    n1538 = call "Origin_Export_7_27a_JW.vi"("Input Conditions"=w2829, "Analysis Array"=w2835, "error in (no error)"=w2837, "Parameter Worksheet Name"="[STable]Threshold Swing", "Parameter Folder Script"="pe_cd \"STS-Sat\";", "Origin.IOApplication"=w2834) -> ("error out"=w2836:errorcluster, "reference out"=w2838:refnum<k7>)  [unwired: 3 in, 1 out]
                    n1539 = call <userlib>:"OAExecute.vi"("script"=w2824, "Error IO"=w2836, "Origin.IOApplication"=w2838) -> ()  [unwired: 1 in, 3 out]
                  }
                  frame #7 {
                    n1540 = local read "Opj X Axis"() -> (w2845:string)
                    n1541 = Concatenate Strings("window -a VtGraph;\nlayer.x.type=", w2845, ";", "window -a VtTable;\nwindow -s TV;") -> (w2843:string)
                    n1542 = call "Param_Analysis_7_24b_JW.vi"("Independant Variable"=w2849, "error in (no error)"=w2854, "Data Folder"=w2852, "Parameter String"="Vt-Sat (V):", "Parameter Name"="Vt-Sat", "Stats Folder"=w2853) -> ("error out"=w2858:errorcluster, "Output Array"=w2856:string[][], "Variables"=w2848:T16)  [unwired: 2 in, 1 out]
                    n1543 = call "Origin_Export_7_27a_JW.vi"("Input Conditions"=w2848, "Analysis Array"=w2856, "error in (no error)"=w2858, "Parameter Worksheet Name"="[VtTable]Threshold Voltages", "Parameter Folder Script"="pe_cd \"Vt-Sat\";", "Origin.IOApplication"=w2855) -> ("error out"=w2857:errorcluster, "reference out"=w2859:refnum<k7>)  [unwired: 3 in, 1 out]
                    n1544 = call <userlib>:"OAExecute.vi"("script"=w2843, "Error IO"=w2857, "Origin.IOApplication"=w2859) -> ("Error IO Out"=w2850:errorcluster, "Origin.IOApplication"=w2851:refnum<k7>)  [unwired: 1 in, 1 out]
                  }
                }
                n1545 = Path To String(path=w2695) -> (string=w2694:string)
                n1546 = call <userlib>:"OAExecute.vi"("script"="pe_cd /; ", "Error IO"=w2690, "Origin.IOApplication"=w2689) -> ("Error IO Out"=w2696:errorcluster, "Origin.IOApplication"=w2697:refnum<k7>)  [unwired: 1 in, 1 out]
                n1547 = call <userlib>:"OASaveProject.vi"("path"=w2694, "Error IO"=w2696, "Origin.IOApplication"=w2697) -> ()  [unwired: 3 out]
              }
            }
          }
          event "Blank Button": Mouse Down {
            n1548 = event-data() -> ()  [unwired: 1 in, 7 out]
            n1549 = local read "Transfer File"() -> (w2874:path)
            n1550 = disable-structure shown="Disabled" {
              frame Disabled {
                n1551 = local read "Folder Index"() -> (w2875:dbl)
                n1552 = Decrement(x=w2875) -> (x-1=w2876:dbl)
                n1553 = local write "Folder Index"(w2876) -> ()
              }
              frame Enabled {
              }
            }
            n1554 = Strip Path(path=w2874) -> (stripped path=w2870:path, name=w2872:string)
            n1555 = Path To String(path=w2870) -> (string=w2869:string)
            n1556 = Concatenate Strings(w2869, "\\", "X_", w2872) -> (w2868:string)
            n1557 = String To Path(string=w2868) -> (path=w2867:path)
            n1558 = Move(source path=w2874, 10:w2867) -> ()  [unwired: 3 in, 3 out]
            n1559 = local write "Transfer File"(w2867) -> ()
          }
          event "Cancel Button": Mouse Down {
            (unwired) 6
            n1560 = event-data() -> ()  [unwired: 1 in, 7 out]
            n1561 = call "Simulate_Keyboard.vi"("Action"=2, "Virtual Key"=162) -> ()  [unwired: 7 in, 1 out]
          }
        }
        n1562 = Multiply(x=w525, y=10) -> (x*y=w527:sgl)
        n1563 = case shown="\"0\"" w566 {
          tunnel: w540 -> [w620 w626 w630 w632 w636 w638 w640 w642 w644 w646 w648 w650 w652 w654 w656 w658 w660 w662 w664 w666 w668 w670 w672 w674 w676 w678 w680 w682 w684 w686 w688 w690 w692 w694 w696 w698 w700 w702 w704 w706 w708 w710 w712 w714 w716 w718 w720 w722 w724 w726 w728 w730 w732 w734 w736 w738 w740 w742 w744 w746 w748 w750 w752 w754 w756 w758 w760 w762 w764 w766 w768 w770 w772 w774 w776 w778 w780 w782 w784 w786 w788 w790 w792 w794 w796 w798 w800 w802 w804 w806 w808 w810 w812 w814 w816 w818 w820 w822 w824 w826 w828 w830 w832 w834 w836]
          tunnel: [w620 w625 w629 w632 w636 w638 w640 w642 w644 w646 w648 w650 w652 w654 w656 w658 w660 w662 w664 w666 w668 w670 w672 w674 w676 w678 w680 w682 w684 w686 w688 w690 w692 w694 w696 w698 w700 w702 w704 w706 w708 w710 w712 w714 w716 w718 w720 w722 w724 w726 w728 w730 w732 w734 w736 w738 w740 w742 w744 w746 w748 w750 w752 w754 w756 w758 w760 w762 w764 w766 w768 w770 w772 w774 w776 w778 w780 w782 w784 w786 w788 w790 w792 w794 w796 w798 w800 w802 w804 w806 w808 w810 w812 w814 w816 w818 w820 w822 w824 w826 w828 w830 w832 w834 w836] -> w565
          tunnel: w541 -> [w622 w624 w628 w634 w635 w637 w639 w641 w643 w645 w647 w649 w651 w653 w655 w657 w659 w661 w663 w665 w667 w669 w671 w673 w675 w677 w679 w681 w683 w685 w687 w689 w691 w693 w695 w697 w699 w701 w703 w705 w707 w709 w711 w713 w715 w717 w719 w721 w723 w725 w727 w729 w731 w733 w735 w737 w739 w741 w743 w745 w747 w749 w751 w753 w755 w757 w759 w761 w763 w765 w767 w769 w771 w773 w775 w777 w779 w781 w783 w785 w787 w789 w791 w793 w795 w797 w799 w801 w803 w805 w807 w809 w811 w813 w815 w817 w819 w821 w823 w825 w827 w829 w831 w833 w835]
          tunnel: [w621 w624 w628 w633 w635 w637 w639 w641 w643 w645 w647 w649 w651 w653 w655 w657 w659 w661 w663 w665 w667 w669 w671 w673 w675 w677 w679 w681 w683 w685 w687 w689 w691 w693 w695 w697 w699 w701 w703 w705 w707 w709 w711 w713 w715 w717 w719 w721 w723 w725 w727 w729 w731 w733 w735 w737 w739 w741 w743 w745 w747 w749 w751 w753 w755 w757 w759 w761 w763 w765 w767 w769 w771 w773 w775 w777 w779 w781 w783 w785 w787 w789 w791 w793 w795 w797 w799 w801 w803 w805 w807 w809 w811 w813 w815 w817 w819 w821 w823 w825 w827 w829 w831 w833 w835] -> w564
          tunnel: w527 -> [w619 w623 w627 w631 _ _ _ _ _ _ _ _ _ _ _ _ _ _ _ _ _ _ _ _ _ _ _ _ _ _ _ _ _ _ _ _ _ _ _ _ _ _ _ _ _ _ _ _ _ _ _ _ _ _ _ _ _ _ _ _ _ _ _ _ _ _ _ _ _ _ _ _ _ _ _ _ _ _ _ _ _ _ _ _ _ _ _ _ _ _ _ _ _ _ _ _ _ _ _ _ _ _ _ _ _]
          frame "DOWN" {
            n1564 = Add(x=w622, y=w619) -> (x+y=w621:sgl)
          }
          frame "LEFT" {
            n1565 = Subtract(x=w626, y=w623) -> (x-y=w625:sgl)
          }
          frame "RIGHT" {
            n1566 = Add(x=w630, y=w627) -> (x+y=w629:sgl)
          }
          frame "UP" {
            n1567 = Subtract(x=w634, y=w631) -> (x-y=w633:sgl)
          }
          frame "ENTER (num pad)" {
          }
          frame "' (quote)" {
          }
          frame "END" {
          }
          frame "EQUALS" {
          }
          frame "ESCAPE" {
          }
          frame "GRAVE (`)" {
          }
          frame "HOME" {
          }
          frame "INSERT" {
          }
          frame "LBRACKET" {
          }
          frame "LCONTROL" {
          }
          frame "L ALT" {
          }
          frame "LSHIFT" {
          }
          frame "LWIN" {
          }
          frame "MINUS" {
          }
          frame "MULTIPLY" {
          }
          frame "NEXT" {
          }
          frame "NUMLOCK" {
          }
          frame "NUMPAD_0" {
          }
          frame "NUMPAD_1" {
          }
          frame "NUMPAD_2" {
          }
          frame "NUMPAD_3" {
          }
          frame "NUMPAD_4" {
          }
          frame "NUMPAD_5" {
          }
          frame "NUMPAD_6" {
          }
          frame "NUMPAD_7" {
          }
          frame "NUMPAD_8" {
          }
          frame "NUMPAD_9" {
          }
          frame "PAUSE" {
          }
          frame "PERIOD" {
          }
          frame "PRIOR (PG UP)" {
          }
          frame "RBRACKET" {
          }
          frame "RCONTROL" {
          }
          frame "RETURN" {
          }
          frame "R ALT" {
          }
          frame "RSHIFT" {
          }
          frame "RWIN" {
          }
          frame "SCROLL" {
          }
          frame "SEMICOLON" {
          }
          frame "SLASH" {
          }
          frame "SPACE" {
          }
          frame "SUBTRACT" {
          }
          frame "TAB" {
          }
          frame "DIVIDE" {
          }
          frame "DELETE" {
          }
          frame "DECIMAL" {
          }
          frame "COMMA" {
          }
          frame "CAPITAL" {
          }
          frame "BACKSLASH" {
          }
          frame "BACK" {
          }
          frame "ADD" {
          }
          frame "F15" {
          }
          frame "F14" {
          }
          frame "F13" {
          }
          frame "F12" {
          }
          frame "F11" {
          }
          frame "F10" {
          }
          frame "F9" {
          }
          frame "F8" {
          }
          frame "F7" {
          }
          frame "F6" {
          }
          frame "F5" {
          }
          frame "F4" {
          }
          frame "F3" {
          }
          frame "F2" {
          }
          frame "F1" {
          }
          frame "Z" {
          }
          frame "Y" {
          }
          frame "X" {
          }
          frame "W" {
          }
          frame "V" {
          }
          frame "U" {
          }
          frame "T" {
          }
          frame "S" {
          }
          frame "R" {
          }
          frame "Q" {
          }
          frame "P" {
          }
          frame "O" {
          }
          frame "N" {
          }
          frame "M" {
          }
          frame "L" {
          }
          frame "K" {
          }
          frame "J" {
          }
          frame "I" {
          }
          frame "H" {
          }
          frame "G" {
          }
          frame "F" {
          }
          frame "E" {
          }
          frame "D" {
          }
          frame "C" {
          }
          frame "B" {
          }
          frame "A" {
          }
          frame "9" {
          }
          frame "8" {
          }
          frame "7" {
          }
          frame "6" {
          }
          frame "5" {
          }
          frame "4" {
          }
          frame "3" {
          }
          frame "2" {
          }
          frame "1" {
          }
          frame "0" {
          }
        }
        n1568 = Bundle(w543, w542, w557, w556, 0.0) -> (w555:cluster{dbl, dbl, dbl, dbl, dbl})  [unwired: 1 in]
        n1569 = Bundle("X"=w565, "Y"=w564) -> (w559:cluster{"X":sgl, "Y":sgl})  [unwired: 1 in]
        n1570 = Divide(x=20, y=w526) -> (x/y=w529:sgl)
        n1571 = property on="Image Out" class="ImageControl"("Image Center Position"=w559) -> ()  [unwired: 2 in, 2 out]
        n1572 = call "IMAQ Convert Rectangle to ROI (Polygon)"("Rectangle"=w555) -> ("ROI Descriptor"=w553:T3)  [unwired: 7 in, 2 out]
        n1573 = Bundle("Application Font", w529, w533, w533, w533, w533, w533, TRUE, w531) -> (w535:T17)  [unwired: 1 in]
        n1574 = property on="Image Out 2" class="ImageControl"("ROI"=w553) -> ()  [unwired: 2 in, 2 out]
        n1575 = Bundle(w531, w535, w531, w531) -> (w534:T18)  [unwired: 1 in]
        n1576 = property on="Image Out" class="ImageControl"() -> ("ROI"=w518:T10)  [unwired: 2 in, 2 out]
        n1577 = Unbundle By Name(w518) -> ("Contours"=w582:T14)
        n1578 = local read "Image Out"() -> (w537:T2)
        n1579 = call "IMAQ Clear Overlay"("Image"=w537) -> ("Image Out"=w536:T2)  [unwired: 9 in, 1 out]
        n1580 = Initialize Array(0) -> (w580:i32[])  [unwired: 1 in]
        n1581 = local read "Magnification"() -> (w571:u16)
        n1582 = Array Size(array=w582) -> (size(s)=w581:i32)
        n1583 = Build Array(0.505025, 0.252522, 0.127742, 0.050345, 0.031129) -> (w572:dbl[])
        n1584 = Array Subset(array=w572, index=w571, length=1) -> (w569:dbl[])
        n1585 = property on="Image Out" class="ImageControl"() -> ("ZoomInteger"=w561:cluster{"X":i32, "Y":i32})  [unwired: 2 in, 2 out]
        n1586 = To Double Precision Float(number=w569) -> (double precision float=w568:dbl[])
        n1587 = for {
          N: w581 -> [_]
          shift-right: [w859] -> _
          shift-left: w582 -> [w859]
          shift-right: [w857] -> w567
          shift-left: w580 -> [w856]
          tunnel: w568 -> [w855]
          shift-right: [w852] -> _
          shift-left: w536 -> [w854]
          tunnel: w534 -> [w847]
          i -> [w851]
          n1588 = Index Array(array=w859, index=w851) -> (element=w868:T19)
          n1589 = Unbundle(w868) -> ("Points"=w867:i32[])  [unwired: 2 out]
          n1590 = Array To Cluster(array=w867) -> (cluster=w866:T20)
          n1591 = Unbundle(w866) -> ("Points[0]"=w846:i32, "Points[1]"=w843:i32, "Points[2]"=w858:i32, "Points[3]"=w864:i32)  [unwired: 5 out]
          n1592 = Add(x=w846, y=10) -> (x+y=w844:i32)
          n1593 = Subtract(x=w843, y=w864) -> (x-y=w863:i32)
          n1594 = Subtract(x=w846, y=w858) -> (x-y=w865:i32)
          n1595 = Square(x=w863) -> (x^2=w861:i32)
          n1596 = Square(x=w865) -> (x^2=w862:i32)
          n1597 = Add(x=w862, y=w861) -> (x+y=w860:i32)
          n1598 = Square Root(x=w860) -> (sqrt(x)=w837:dbl)
          n1599 = Multiply(x=w837, y=0.5) -> (x*y=w840:dbl)
          n1600 = Add(x=w840, y=w843) -> (x+y=w842:dbl)
          n1601 = Bundle(w844, w842) -> (w853:cluster{i32, dbl})  [unwired: 1 in]
          n1602 = Multiply(x=w837, y=w855) -> (x*y=w850:dbl[])
          n1603 = Index Array(array=w850) -> (element=w849:dbl)  [unwired: 1 in]
          n1604 = Number To Fractional String(number=w849) -> (F-format string=w848:string)  [unwired: 3 in]
          n1605 = call "IMAQ Overlay Text"("BG Color (Transparent)"=u32 0, "Text Color (black)"=u32 16448250, "Font, Size & Style"=w847, "String"=w848, "Origin"=w853, "Image"=w854) -> ("Image Out"=w852:T2)  [unwired: 4 in, 1 out]
          n1606 = Build Array (concatenate)(w856, w850) -> (w857:dbl[])
          n1607 = local write "Numeric 3"(w837) -> ()
        }
        n1608 = local write "ROI Descriptor"(w518) -> ()
        n1609 = Unbundle(w561) -> ("X"=w560:i32)  [unwired: 1 out]
        n1610 = Add Array Elements(numeric array=w567) -> (sum=w578:dbl)
        n1611 = local write "Distances"(w567) -> ()
        n1612 = local write "Total Width"(w578) -> ()
        n1613 = local write "Zoom"(w560) -> ()
        n1614 = local read "Manual-Width"() -> (w517:bool)
        n1615 = local read "Total Width"() -> (w521:dbl)
        n1616 = local read "Rec: Width"() -> (w519:dbl)
        n1617 = Not(x=w517) -> (.not. x?=w515:bool)
        n1618 = Equal To 0?(x=w521) -> (x = 0?=w516:bool)
        n1619 = Or(x=w516, y=w517) -> (x .or. y?=w520:bool)
        n1620 = And(x=w516, y=w515) -> (x .and. y?=w514:bool)
        n1621 = case shown="True" w514 {
          tunnel: w519 -> [_ w597]
          frame False {
          }
          frame True {
            n1622 = local write "New: Width"(w597) -> ()
          }
        }
        n1623 = case shown="False" w520 {
          tunnel: w521 -> [w598 _]
          frame False {
            n1624 = local write "New: Width"(w598) -> ()
          }
          frame True {
          }
        }
        n1625 = local read "Manuel-Dielectric"() -> (w443:bool)
        n1626 = local read "Rec: Dielectric (d)"() -> (w442:dbl)
        n1627 = local read "Manuel-Length"() -> (w444:bool)
        n1628 = local read "Manual-Temp"() -> (w416:bool)
        n1629 = local read "Rec: Length"() -> (w445:dbl)
        n1630 = local read "Rec: Temp"() -> (w417:dbl)
        n1631 = case shown="False" w444 {
          tunnel: w445 -> [w588 _]
          frame False {
            n1632 = local write "New: Length"(w588) -> ()
          }
          frame True {
          }
        }
        n1633 = case shown="False" w443 {
          tunnel: w442 -> [w587 _]
          frame False {
            n1634 = local write "New: Dielectric"(w587) -> ()
          }
          frame True {
          }
        }
        n1635 = case shown="False" w416 {
          tunnel: w417 -> [w584 _]
          frame False {
            n1636 = local write "New: Temp"(w584) -> ()
          }
          frame True {
          }
        }
      }
    }
  }
  n1637 = Build Array("DeviceID", "Fabricator", "Deposition", "Date", "Sample", "Row", "Column", "L (um)", "W (um)", "Material", "Treatment", "TC (mM)", "Solvent", "C (%)", "ST (C)", "Drops", "Wait (s)", "RT (F)", "RH (%)", "Ramp (s)", "RPM", "Accel (RPM/s)", "Time (s)", "Mobility", "On/Off", "Vt", "S.T.S") -> (→"Transformer \nHeaders":string[])
